vi "WVDIAL+HSRL_v4.5.vi"() -> ()   [LabVIEW 2012]
uses:
  C:/Users/H2ODial/Desktop/Shared Telescope WV DIAL Code/Libraries and VIs/PowerMeterCommands.dll
  Shared Telescope WV DIAL Code/Libraries and VIs/PowerMeterCommands.dll
  <vilib>/DAQmx/write.llb/DAQmx Write (Digital 1D Bool NChan 1Samp 1Line).vi
  <vilib>/DAQmx/miscellaneous.llb/DAQmx Fill In Error Info.vi
  <vilib>/Analysis/baseanly.llb/Mean (DBL).vi
  NCAR_DIAL_Labview/AMCS_Data.vi
  Shared Telescope WV DIAL Code/Libraries and VIs/Scalar_Data.vi
  <vilib>/Analysis/NI_AALBase.lvlib
  Shared Telescope WV DIAL Code/Libraries and VIs/Scalar_Data_2.vi
  Shared Telescope WV DIAL Code/Libraries and VIs/Scalar_Data_4.vi
  Shared Telescope WV DIAL Code/Libraries and VIs/Scalar_Data_3.vi
  Shared Telescope WV DIAL Code/bristol/CLDevIFace.dll
panel:
  out "FileHour":i32=22
  out "L_Count":i32=26
  out "background start":u32=534
  in  "Tab Control 2":enum32{"WV ND narrow", "WV ND wide"}(tab)
  out "CH3 RingBuffer long":dbl[][](array[numeric])
  out "CH3 RingBuffer short":dbl[][](array[numeric])
  in  "?":T1(tab)=enum."Raw Counts WV offline"
  out "NRB":dbl[][](graph) caption="Water Vapor Number Density"
  out "NRB 2":dbl[][](graph) caption="Water Vapor Number Density"
  out "CH 1 (WV off) counts display":dbl[][](graph)=[[72.12, 61.12, 47.12, 35.12, 44.12, 29.119999999999997, 55.12, 61.12, 47.12, 50.12, 55.12, 52.12, 68.12, 67.12, 90.12, 116.12, 122.12, 143.12, 189.12, 221.12, 229.12, 278.12, 272.12, 337.12, 351.12, 384.12, 391.12, 406.12, 455.12, 483.12, 506.12, 561.12, 539.12, 595.12, 572.12, 618.12, 622.12, 629.12, 627.12, 625.12, 613.12, 546.12, 551.12, 501.12, 476.12, 497.12, 468.12, 447.12, 391.12, 371.12, 370.12, 307.12, 290.12, 246.12, 236.12, 202.12, 237.12, 195.12, 179.12, 160.12, 142.12, 148.12, 128.12, 146.12, 132.12, 115.12, 128.12, 110.12, 91.12, 101.12, 91.12, 110.12, 101.12, 107.12, 70.12, 79.12, 81.12, 83.12, 73.12, 85.12, 77.12, 81.12, 80.12, 59.12, 76.12, 83.12, 62.12, 78.12, 75.12, 67.12, 38.12, 41.12, 47.12, 63.12, 51.12, 54.12, 58.12, 30.119999999999997, 23.119999999999997, 28.119999999999997, 23.119999999999997, 27.119999999999997, 16.119999999999997, 32.12, 40.12, 31.119999999999997, 19.119999999999997, 23.119999999999997, 26.119999999999997, 22.119999999999997, 29.119999999999997, 21.119999999999997, 8.119999999999997, 24.119999999999997, 18.119999999999997, 19.119999999999997, 33.12, 17.119999999999997, 24.119999999999997, 19.119999999999997, 12.119999999999997, 14.119999999999997, 17.119999999999997, 9.119999999999997, 24.119999999999997, 22.119999999999997, 31.119999999999997, 17.119999999999997, 9.119999999999997, 17.119999999999997, 24.119999999999997, 13.119999999999997, 4.119999999999997, 26.119999999999997, 16.119999999999997, 18.119999999999997, 11.119999999999997, 14.119999999999997, 9.119999999999997, 24.119999999999997, 6.119999999999997, 12.119999999999997, 7.119999999999997, 22.119999999999997, 3.1199999999999974, 9.119999999999997, 8.119999999999997, 16.119999999999997, 11.119999999999997, 10.119999999999997, 4.119999999999997, 0.11999999999999744, 8.119999999999997, 17.119999999999997, 3.1199999999999974, 15.119999999999997, 8.119999999999997, 4.119999999999997, 10.119999999999997, -1.8800000000000026, 7.119999999999997, 10.119999999999997, 5.119999999999997, -7.880000000000003, 2.1199999999999974, 6.119999999999997, 4.119999999999997, 13.119999999999997, 21.119999999999997, 11.119999999999997, 10.119999999999997, 3.1199999999999974, 18.119999999999997, 20.119999999999997, 10.119999999999997, 13.119999999999997, -4.880000000000003, 5.119999999999997, 9.119999999999997, 6.119999999999997, -4.880000000000003, 0.11999999999999744, 1.1199999999999974, 8.119999999999997, 5.119999999999997, 4.119999999999997, 2.1199999999999974, 3.1199999999999974, 21.119999999999997, 8.119999999999997, -0.8800000000000026, 1.1199999999999974, 9.119999999999997, 8.119999999999997, 8.119999999999997, 5.119999999999997, 1.1199999999999974, 2.1199999999999974, 2.1199999999999974, -4.880000000000003, 7.119999999999997, 2.1199999999999974, 9.119999999999997, 1.1199999999999974, -1.8800000000000026, -2.8800000000000026, -2.8800000000000026, 3.1199999999999974, 8.119999999999997, 8.119999999999997, -0.8800000000000026, 2.1199999999999974, 12.119999999999997, 8.119999999999997, -1.8800000000000026, 10.119999999999997, 1.1199999999999974, 9.119999999999997, 3.1199999999999974, 14.119999999999997, 11.119999999999997, 3.1199999999999974, 3.1199999999999974, -0.8800000000000026, -2.8800000000000026, 1.1199999999999974, 2.1199999999999974, -0.8800000000000026, 9.119999999999997, 4.119999999999997, 5.119999999999997, -7.880000000000003, -2.8800000000000026, 1.1199999999999974, -2.8800000000000026, 13.119999999999997, 26.119999999999997, 0.11999999999999744, 1.1199999999999974, 1.1199999999999974, 7.119999999999997, 3.1199999999999974, -2.8800000000000026, -8.880000000000003, 5.119999999999997, -2.8800000000000026, 2.1199999999999974, 0.11999999999999744, -1.8800000000000026, -4.880000000000003, 0.11999999999999744, 3.1199999999999974, 2.1199999999999974, 0.11999999999999744, 2.1199999999999974, 11.119999999999997, -7.880000000000003, 6.119999999999997, 10.119999999999997, 2.1199999999999974, 5.119999999999997, 2.1199999999999974, -6.880000000000003, 6.119999999999997, 8.119999999999997, 6.119999999999997, 9.119999999999997, -7.880000000000003, -0.8800000000000026, 6.119999999999997, 1.1199999999999974, 3.1199999999999974, -6.880000000000003, -7.880000000000003, 7.119999999999997, 2.1199999999999974, 5.119999999999997, 1.1199999999999974, -8.880000000000003, 0.11999999999999744, 0.11999999999999744, 8.119999999999997, 1.1199999999999974, 0.11999999999999744, 13.119999999999997, 0.11999999999999744, -0.8800000000000026, -2.8800000000000026, 2.1199999999999974, 5.119999999999997, 16.119999999999997, 10.119999999999997, 16.119999999999997, 6.119999999999997, -1.8800000000000026, 3.1199999999999974, -6.880000000000003, 7.119999999999997, -3.8800000000000026, -2.8800000000000026, -2.8800000000000026, -0.8800000000000026, -12.880000000000003, 2.1199999999999974, -4.880000000000003, -0.8800000000000026, -2.8800000000000026, 7.119999999999997, -5.880000000000003, -5.880000000000003, 2.1199999999999974, -7.880000000000003, 8.119999999999997, -3.8800000000000026, 1.1199999999999974, 0.11999999999999744, 5.119999999999997, -0.8800000000000026, 0.11999999999999744, 6.119999999999997, -2.8800000000000026, -4.880000000000003, -1.8800000000000026, 1.1199999999999974, -6.880000000000003, -0.8800000000000026, 1.1199999999999974, 8.119999999999997, 6.119999999999997, 9.119999999999997, 11.119999999999997, -2.8800000000000026, -5.880000000000003, -1.8800000000000026, 11.119999999999997, 13.119999999999997, 4.119999999999997, -7.880000000000003, 6.119999999999997, -5.880000000000003, -6.880000000000003, 2.1199999999999974, 4.119999999999997, 1.1199999999999974, 0.11999999999999744, 4.119999999999997, 1.1199999999999974, 12.119999999999997, -5.880000000000003, 4.119999999999997, -3.8800000000000026, 2.1199999999999974, 4.119999999999997, 8.119999999999997, 3.1199999999999974, 3.1199999999999974, 13.119999999999997, 1.1199999999999974, 11.119999999999997, -12.880000000000003, 5.119999999999997, -0.8800000000000026, -2.8800000000000026, -0.8800000000000026, -9.880000000000003, 7.119999999999997, -3.8800000000000026, 10.119999999999997, -2.8800000000000026, 4.119999999999997, 3.1199999999999974, 5.119999999999997, -2.8800000000000026, 5.119999999999997, 3.1199999999999974, 7.119999999999997, -11.880000000000003, 5.119999999999997, -0.8800000000000026, -2.8800000000000026, 0.11999999999999744, 1.1199999999999974, 13.119999999999997, 7.119999999999997, 2.1199999999999974, 1.1199999999999974, 1.1199999999999974, -0.8800000000000026, -5.880000000000003, 7.119999999999997, 6.119999999999997, -0.8800000000000026, -2.8800000000000026, 0.11999999999999744, -1.8800000000000026, -9.880000000000003, 2.1199999999999974, -1.8800000000000026, -3.8800000000000026, 3.1199999999999974, -3.8800000000000026, 2.1199999999999974, 2.1199999999999974, -2.8800000000000026, -4.880000000000003, -2.8800000000000026, 2.1199999999999974, -7.880000000000003, 13.119999999999997, 0.11999999999999744, 4.119999999999997, 3.1199999999999974, -0.8800000000000026, -8.880000000000003, 2.1199999999999974, -1.8800000000000026, -1.8800000000000026, 4.119999999999997, 2.1199999999999974, 2.1199999999999974, -6.880000000000003, -6.880000000000003, -8.880000000000003, -0.8800000000000026, -0.8800000000000026, 1.1199999999999974, -0.8800000000000026, -1.8800000000000026, 0.11999999999999744, 4.119999999999997, -2.8800000000000026, -4.880000000000003, -3.8800000000000026, -3.8800000000000026, 5.119999999999997, 5.119999999999997, 2.1199999999999974, -5.880000000000003, -0.8800000000000026, -7.880000000000003, -1.8800000000000026, -6.880000000000003, -7.880000000000003, 10.119999999999997, 8.119999999999997, 4.119999999999997, 5.119999999999997, 3.1199999999999974, -0.8800000000000026, -1.8800000000000026, -12.880000000000003, -7.880000000000003, 2.1199999999999974, 1.1199999999999974, -4.880000000000003, -7.880000000000003, 1.1199999999999974, 0.11999999999999744, -3.8800000000000026, 0.11999999999999744, -5.880000000000003, 0.11999999999999744, 3.1199999999999974, 16.119999999999997, 2.1199999999999974, 3.1199999999999974, 0.11999999999999744, -2.8800000000000026, 2.1199999999999974, 6.119999999999997, 1.1199999999999974, -4.880000000000003, 3.1199999999999974, 15.119999999999997, -13.880000000000003, 9.119999999999997, -0.8800000000000026, -2.8800000000000026, 10.119999999999997, 7.119999999999997, 4.119999999999997, -1.8800000000000026, 11.119999999999997, 8.119999999999997, 0.11999999999999744, 3.1199999999999974, 8.119999999999997, 1.1199999999999974, 2.1199999999999974, -11.880000000000003, 3.1199999999999974, 10.119999999999997, -2.8800000000000026, 3.1199999999999974, 7.119999999999997, -2.8800000000000026, -2.8800000000000026, -2.8800000000000026, -1.8800000000000026, 5.119999999999997, 0.11999999999999744, -2.8800000000000026, 5.119999999999997, -1.8800000000000026, -4.880000000000003, 0.11999999999999744, -7.880000000000003, -10.880000000000003, -1.8800000000000026, -2.8800000000000026, -3.8800000000000026, 1.1199999999999974, -2.8800000000000026, -0.8800000000000026, -7.880000000000003, -2.8800000000000026, 9.119999999999997, 0.11999999999999744, -5.880000000000003, 6.119999999999997, -1.8800000000000026, -0.8800000000000026, 1.1199999999999974, 5.119999999999997, 12.119999999999997, 14.119999999999997, 9.119999999999997, -2.8800000000000026, -3.8800000000000026, -7.880000000000003, -1.8800000000000026, 9.119999999999997, -8.880000000000003, 5.119999999999997, -2.8800000000000026, -5.880000000000003, -0.8800000000000026, -8.880000000000003, -1.8800000000000026, -5.880000000000003, 12.119999999999997, -2.8800000000000026, 4.119999999999997, 1.1199999999999974, 10.119999999999997, 4.119999999999997, -4.880000000000003, -3.8800000000000026, -1.8800000000000026, 8.119999999999997, 1.1199999999999974, -0.8800000000000026, -5.880000000000003, 3.1199999999999974, -9.880000000000003, -3.8800000000000026, 5.119999999999997, 2.1199999999999974, 9.119999999999997, 0.0]] caption="Water Vapor Number Density"
  out "CH 3 (HSRL comb) counts display":dbl[][](graph)=[[191.68, 101.68, 62.68000000000001, 122.68, 46.68000000000001, 67.68, 96.68, 112.68, 96.68, 178.68, 157.68, 156.68, 268.68, 230.68, 382.68, 361.68, 473.68, 521.6800000000001, 591.6800000000001, 641.6800000000001, 732.6800000000001, 820.6800000000001, 938.6800000000001, 1045.68, 1138.68, 1222.68, 1329.68, 1319.68, 1345.68, 1475.68, 1466.68, 1519.68, 1569.68, 1698.68, 1666.68, 1581.68, 1707.68, 1691.68, 1629.68, 1560.68, 1616.68, 1487.68, 1526.68, 1348.68, 1236.68, 1209.68, 1105.68, 1027.68, 970.6800000000001, 878.6800000000001, 821.6800000000001, 781.6800000000001, 646.6800000000001, 643.6800000000001, 521.6800000000001, 577.6800000000001, 505.68, 511.68, 457.68, 406.68, 391.68, 343.68, 300.68, 360.68, 268.68, 246.68, 294.68, 246.68, 241.68, 249.68, 210.68, 201.68, 201.68, 198.68, 216.68, 177.68, 157.68, 140.68, 184.68, 163.68, 154.68, 156.68, 178.68, 176.68, 137.68, 206.68, 174.68, 182.68, 148.68, 153.68, 116.68, 133.68, 117.68, 118.68, 134.68, 120.68, 110.68, 76.68, 105.68, 75.68, 147.68, 34.68000000000001, 41.68000000000001, 65.68, 54.68000000000001, 87.68, 57.68000000000001, 61.68000000000001, 59.68000000000001, 25.680000000000007, 71.68, 88.68, 31.680000000000007, 32.68000000000001, 51.68000000000001, 66.68, 75.68, 51.68000000000001, 39.68000000000001, 51.68000000000001, 40.68000000000001, 55.68000000000001, 38.68000000000001, 22.680000000000007, 20.680000000000007, 50.68000000000001, 12.680000000000007, 40.68000000000001, 11.680000000000007, 28.680000000000007, 26.680000000000007, 23.680000000000007, 28.680000000000007, 8.680000000000007, 34.68000000000001, 20.680000000000007, 57.68000000000001, -17.319999999999993, 48.68000000000001, 40.68000000000001, 83.68, -1.3199999999999932, 33.68000000000001, 42.68000000000001, 29.680000000000007, 13.680000000000007, 25.680000000000007, 10.680000000000007, 31.680000000000007, 31.680000000000007, 4.680000000000007, 15.680000000000007, 36.68000000000001, 20.680000000000007, -0.3199999999999932, 40.68000000000001, -2.319999999999993, 21.680000000000007, 19.680000000000007, -14.319999999999993, 32.68000000000001, 39.68000000000001, 48.68000000000001, 17.680000000000007, -5.319999999999993, 13.680000000000007, 0.6800000000000068, 23.680000000000007, 26.680000000000007, -14.319999999999993, -7.319999999999993, 15.680000000000007, 20.680000000000007, -19.319999999999993, 14.680000000000007, 38.68000000000001, 5.680000000000007, 11.680000000000007, 18.680000000000007, 12.680000000000007, -5.319999999999993, 40.68000000000001, -11.319999999999993, 15.680000000000007, -17.319999999999993, -12.319999999999993, 9.680000000000007, 13.680000000000007, -23.319999999999993, -6.319999999999993, 28.680000000000007, 8.680000000000007, 24.680000000000007, 34.68000000000001, -24.319999999999993, 24.680000000000007, -32.31999999999999, 13.680000000000007, 29.680000000000007, 9.680000000000007, -16.319999999999993, -4.319999999999993, -15.319999999999993, 22.680000000000007, 13.680000000000007, 17.680000000000007, 21.680000000000007, 30.680000000000007, 1.6800000000000068, 60.68000000000001, -6.319999999999993, 1.6800000000000068, -11.319999999999993, 20.680000000000007, 31.680000000000007, 18.680000000000007, 0.6800000000000068, 16.680000000000007, 21.680000000000007, -11.319999999999993, -3.319999999999993, -8.319999999999993, 12.680000000000007, -10.319999999999993, 31.680000000000007, 11.680000000000007, 32.68000000000001, 21.680000000000007, 26.680000000000007, -24.319999999999993, 0.6800000000000068, -2.319999999999993, -6.319999999999993, -1.3199999999999932, -10.319999999999993, 12.680000000000007, 1.6800000000000068, 7.680000000000007, 14.680000000000007, 1.6800000000000068, -5.319999999999993, -27.319999999999993, 9.680000000000007, -0.3199999999999932, -8.319999999999993, 30.680000000000007, -9.319999999999993, 1.6800000000000068, -4.319999999999993, 18.680000000000007, 26.680000000000007, 3.680000000000007, -12.319999999999993, 14.680000000000007, -12.319999999999993, 58.68000000000001, -10.319999999999993, 18.680000000000007, 13.680000000000007, -12.319999999999993, 31.680000000000007, -37.31999999999999, -23.319999999999993, 8.680000000000007, -5.319999999999993, 28.680000000000007, 17.680000000000007, 12.680000000000007, -4.319999999999993, 25.680000000000007, 18.680000000000007, -10.319999999999993, -4.319999999999993, -23.319999999999993, 10.680000000000007, -20.319999999999993, 8.680000000000007, 22.680000000000007, 10.680000000000007, 39.68000000000001, -20.319999999999993, -16.319999999999993, 13.680000000000007, 13.680000000000007, -27.319999999999993, 10.680000000000007, -8.319999999999993, 65.68, -4.319999999999993, 26.680000000000007, 2.680000000000007, -4.319999999999993, 5.680000000000007, -2.319999999999993, 19.680000000000007, 8.680000000000007, -36.31999999999999, -21.319999999999993, -6.319999999999993, -11.319999999999993, 6.680000000000007, 3.680000000000007, -8.319999999999993, 17.680000000000007, 26.680000000000007, 16.680000000000007, -11.319999999999993, 22.680000000000007, 0.6800000000000068, 13.680000000000007, 10.680000000000007, -23.319999999999993, 11.680000000000007, 16.680000000000007, -17.319999999999993, 9.680000000000007, -45.31999999999999, 8.680000000000007, 45.68000000000001, 16.680000000000007, -24.319999999999993, -26.319999999999993, 13.680000000000007, 2.680000000000007, -2.319999999999993, 1.6800000000000068, 33.68000000000001, -12.319999999999993, 0.6800000000000068, -2.319999999999993, 25.680000000000007, -46.31999999999999, 48.68000000000001, -30.319999999999993, 5.680000000000007, 11.680000000000007, 11.680000000000007, -14.319999999999993, -26.319999999999993, 40.68000000000001, 29.680000000000007, -3.319999999999993, -5.319999999999993, 17.680000000000007, -19.319999999999993, -12.319999999999993, -19.319999999999993, -14.319999999999993, 0.6800000000000068, 1.6800000000000068, 4.680000000000007, 4.680000000000007, -9.319999999999993, 26.680000000000007, -10.319999999999993, -4.319999999999993, -2.319999999999993, 32.68000000000001, 12.680000000000007, -9.319999999999993, 31.680000000000007, 33.68000000000001, -6.319999999999993, 14.680000000000007, 38.68000000000001, -15.319999999999993, -0.3199999999999932, 26.680000000000007, -21.319999999999993, 7.680000000000007, -22.319999999999993, 0.6800000000000068, 30.680000000000007, -11.319999999999993, 18.680000000000007, 8.680000000000007, 2.680000000000007, 18.680000000000007, 7.680000000000007, 31.680000000000007, 25.680000000000007, 37.68000000000001, 3.680000000000007, -22.319999999999993, -7.319999999999993, -22.319999999999993, 2.680000000000007, 23.680000000000007, 12.680000000000007, -38.31999999999999, 3.680000000000007, 27.680000000000007, -0.3199999999999932, -18.319999999999993, 5.680000000000007, -10.319999999999993, 17.680000000000007, -17.319999999999993, 35.68000000000001, 20.680000000000007, 14.680000000000007, -2.319999999999993, -10.319999999999993, 3.680000000000007, -25.319999999999993, 18.680000000000007, -6.319999999999993, -11.319999999999993, 11.680000000000007, 3.680000000000007, 34.68000000000001, -5.319999999999993, -19.319999999999993, 29.680000000000007, -21.319999999999993, 17.680000000000007, -11.319999999999993, 18.680000000000007, 13.680000000000007, -12.319999999999993, 16.680000000000007, -14.319999999999993, 5.680000000000007, -19.319999999999993, -15.319999999999993, 6.680000000000007, 14.680000000000007, -14.319999999999993, 25.680000000000007, 32.68000000000001, -35.31999999999999, 34.68000000000001, 15.680000000000007, -15.319999999999993, 36.68000000000001, -13.319999999999993, 4.680000000000007, 1.6800000000000068, -16.319999999999993, -20.319999999999993, 14.680000000000007, 20.680000000000007, -14.319999999999993, -22.319999999999993, -36.31999999999999, -10.319999999999993, 16.680000000000007, -10.319999999999993, 28.680000000000007, 8.680000000000007, -9.319999999999993, 9.680000000000007, 13.680000000000007, -2.319999999999993, 31.680000000000007, 36.68000000000001, -3.319999999999993, 7.680000000000007, -16.319999999999993, -14.319999999999993, 27.680000000000007, 34.68000000000001, 15.680000000000007, -48.31999999999999, 0.6800000000000068, -11.319999999999993, -7.319999999999993, -15.319999999999993, -13.319999999999993, 15.680000000000007, -27.319999999999993, 0.6800000000000068, -13.319999999999993, -9.319999999999993, -12.319999999999993, 1.6800000000000068, 4.680000000000007, -1.3199999999999932, 17.680000000000007, -6.319999999999993, 15.680000000000007, 9.680000000000007, 51.68000000000001, -13.319999999999993, -0.3199999999999932, 43.68000000000001, -17.319999999999993, 10.680000000000007, 1.6800000000000068, -16.319999999999993, -5.319999999999993, -31.319999999999993, 38.68000000000001, 17.680000000000007, -24.319999999999993, 36.68000000000001, -22.319999999999993, -7.319999999999993, -41.31999999999999, 23.680000000000007, -0.3199999999999932, 38.68000000000001, -12.319999999999993, 40.68000000000001, 16.680000000000007, -0.3199999999999932, 4.680000000000007, -18.319999999999993, -3.319999999999993, -20.319999999999993, 20.680000000000007, -32.31999999999999, -37.31999999999999, -5.319999999999993, -25.319999999999993, -12.319999999999993, 27.680000000000007, -17.319999999999993, -23.319999999999993, 20.680000000000007, 45.68000000000001, -23.319999999999993, 10.680000000000007, -36.31999999999999, 7.680000000000007, -30.319999999999993, 43.68000000000001, 24.680000000000007, -26.319999999999993, 17.680000000000007, -4.319999999999993, -0.3199999999999932, -45.31999999999999, -1.3199999999999932, 8.680000000000007, -13.319999999999993, -27.319999999999993, -14.319999999999993, 10.680000000000007, -17.319999999999993, -39.31999999999999, 20.680000000000007, -38.31999999999999, 8.680000000000007, -5.319999999999993, 27.680000000000007, -5.319999999999993, 13.680000000000007, -5.319999999999993, -14.319999999999993, 24.680000000000007, 8.680000000000007, 1.6800000000000068, 14.680000000000007, 5.680000000000007, 31.680000000000007, -2.319999999999993, 33.68000000000001, -28.319999999999993, 0.0]] caption="Water Vapor Number Density"
  out "CH3 (HSRL combined) smooth S":dbl[](array[numeric])=[96.57850299401198, 56.5485628742515, 55.743173652694615, 60.75365269461079, 68.32101796407187, 79.13089820359284, 91.49317365269464, 103.12341317365271, 117.9422754491018, 136.07401197604787, 156.80904191616764, 183.49467065868262, 215.12191616766466, 251.2985628742515, 292.9602395209581, 339.6967664670659, 389.76263473053893, 444.4722155688622, 499.4991616766466, 554.9482634730538, 610.9767065868263, 666.3225149700597, 722.5261077844309, 775.5335928143711, 824.4602395209581, 870.2566467065868, 910.9826946107785, 946.3719161676647, 976.2416766467067, 996.7252095808384, 1009.2656287425151, 1012.3225149700601, 1009.514131736527, 996.7431736526947, 977.3794011976049, 952.3314970059882, 918.1353892215569, 883.2297005988024, 842.770119760479, 803.6967664670657, 765.9901796407183, 730.4228143712572, 698.6144311377244, 665.4332934131735, 632.464730538922, 597.6563473053891, 562.395868263473, 527.2476646706585, 490.38389221556884, 453.2596407185628, 416.91982035928146, 384.87790419161684, 359.6308982035929, 339.24916167664674, 323.0964670658683, 306.9407784431138, 290.8943712574851, 275.00814371257485, 259.09497005988027, 245.14586826347306, 232.85544910179638, 219.72820359281437, 209.2985628742515, 199.46173652694605, 190.8764071856287, 184.17880239520954, 177.13538922155684, 171.00514970059874, 164.5335928143712, 159.33748502994007, 153.19077844311371, 146.91532934131732, 140.66682634730535, 133.9497604790419, 127.57850299401198, 121.32850299401197, 116.12790419161676, 111.50814371257485, 107.55305389221559, 105.40335329341318, 100.72970059880242, 97.00215568862279, 93.73269461077848, 89.03808383233537, 85.88538922155692, 82.84347305389224, 78.60844311377248, 74.91832335329343, 71.71473053892218, 67.18628742514973, 64.15634730538923, 60.55305389221558, 58.217724550898204, 55.970718562874254, 54.10694610778443, 51.50065868263473, 49.30604790419162, 48.15335329341319, 45.8165269461078, 44.460239520958105, 41.942275449101814, 40.92131736526947, 39.90035928143714, 39.27610778443116, 38.603952095808395, 37.83149700598804, 36.43329341317367, 35.211736526946126, 34.198263473053906, 32.17730538922157, 31.78359281437127, 30.72670658682636, 30.120419161676665, 29.090479041916193, 27.45275449101798, 27.16083832335331, 26.844970059880254, 26.455748502994023, 26.82850299401199, 25.8734131736527, 24.551556886227544, 23.198263473053885, 22.36892215568862, 22.11592814371257, 21.767125748502984, 21.66383233532933, 21.29556886227544, 19.8180239520958, 18.47970059880239, 17.994670658682626, 16.57850299401197, 17.27161676646706, 17.111437125748495, 17.017125748502988, 17.100958083832328, 16.057544910179637, 16.803053892215566, 16.35844311377245, 16.12041916167664, 15.717724550898199, 14.449760479041911, 14.097964071856282, 13.937784431137722, 12.99766467065868, 12.740179640718562, 12.024610778443115, 11.10994011976048, 11.081497005988027, 11.527604790419161, 11.419820359281436, 12.032095808383232, 12.350958083832333, 11.291077844311376, 10.617425149700598, 10.120419161676647, 9.60245508982036, 9.635389221556888, 10.02610778443114, 9.349461077844314, 8.891377245508984, 8.46622754491018, 7.355449101796408, 7.225209580838324, 7.153353293413174, 7.925808383233534, 8.484191616766466, 7.698263473053894, 8.123413173652695, 7.041077844311378, 7.35994011976048, 7.412335329341318, 6.8404790419161685, 6.994670658682637, 6.331497005988025, 7.01562874251497, 6.918323353293413, 6.858443113772456, 6.587485029940119, 6.332994011976048, 6.319520958083834, 5.9048502994011995, 5.970718562874254, 5.045568862275452, 5.148862275449105, 5.349461077844313, 5.244670658682637, 6.243173652694611, 6.478203592814372, 6.171317365269461, 5.891377245508982, 5.395868263473056, 4.359940119760481, 4.858443113772457, 4.732694610778444, 4.392874251497008, 5.433293413173654, 4.508143712574853, 4.328502994011979, 4.924311377245511, 4.232694610778445, 4.409341317365271, 4.756646706586827, 4.835988023952097, 4.984191616766468, 5.324011976047905, 4.69676646706587, 4.080000000000002, 3.255149700598805, 2.2850898203592838, 3.121916167664673, 2.8554491017964096, 3.1114371257485054, 3.2626347305389243, 2.801556886227547, 1.982694610778445, 1.7686227544910205, 1.1413772455089841, 0.8973652694610804, 1.7386826347305413, 2.3539520958083853, 3.216227544910182, 3.3105389221556907, 3.077005988023955, 2.6773053892215595, 2.3045508982035954, 2.303053892215571, 2.6563473053892235, 2.057544910179643, 1.9782035928143733, 1.376407185628745, 0.844970059880242, 1.2252095808383259, 1.1413772455089846, 1.29107784431138, 1.0829940119760506, 1.2057485029940147, 1.3779041916167691, 0.921317365269464, 1.446766467065871, 1.1204191616766492, 1.1398802395209604, 1.4392814371257507, 1.5755089820359305, 1.5036526946107809, 1.5680239520958112, 1.5051497005988053, 0.9677245508982063, 0.9707185628742541, 0.6518562874251523, 0.6653293413173678, 0.8704191616766495, 0.8240119760479069, 0.5291017964071884, 0.3569461077844339, -0.30473053892215296, -0.3092215568862249, -0.13257485029939847, -0.050239520958081194, 0.28359281437126016, -0.16850299401197344, -0.14155688622754228, 0.4767065868263499, 0.8449700598802421, 1.4647305389221583, 2.258143712574853, 2.856946107784433, 3.120419161676649, 2.608443113772457, 1.3165269461077869, 0.23568862275449384, -0.008323353293410496, -0.22838323353293155, 0.30604790419161926, 0.6563473053892241, 0.5695209580838348, 1.1728143712574877, 1.2596407185628768, 0.8988622754491045, 0.5785029940119788, 0.1907784431137751, -0.5113173652694584, -0.554730538922153, -0.49335329341317097, 0.6368862275449125, 1.9871856287425171, 1.6638323353293438, 2.318023952095811, 1.7521556886227572, 0.8344910179640747, 1.3808982035928172, 0.47670658682635, 0.3344910179640745, 0.5081437125748529, 0.9018562874251522, 1.223712574850302, 0.3644311377245535, 0.2551497005988051, -0.3825748502993984, 0.03359281437126005, 0.6204191616766492, 0.6638323353293438, -0.0023353293413148624, -0.5143113772455064, -0.6355688622754464, 0.024610778443116432, 1.0485628742514996, 1.2087425149700626, 1.011137724550901, 0.37191616766467334, 0.6922754491017991, 0.16233532934132008, 0.7761077844311401, 0.9826946107784456, 0.31802395209581097, 0.44377245508982277, -0.4469461077844284, -0.2822754491017937, -0.45443113772454824, -0.38257485029939853, 0.1862874251497032, -0.2388622754490992, 0.22670658682634998, 0.15485029940120032, 0.20125748502994284, 0.024610778443116488, -0.027784431137721888, -0.4484431137724524, -0.988862275449099, 0.17281437125748766, 0.2222155688622779, 1.002155688622757, 1.6608383233532957, 0.7416766467065893, 0.3674251497006015, -0.28227544910179364, -0.5831736526946081, -0.5697005988023924, -0.5652095808383207, -0.2448502994011949, -0.16401197604790152, -0.021796407185626004, 0.05754491017964346, 0.4662275449101823, 0.19676646706587098, -0.49335329341317097, -0.8092215568862249, -1.1580239520958058, -0.9828742514970034, 0.02910179640718835, 0.14736526946108053, -0.16550898203592546, 0.08748502994012246, -1.4274850299401172, -2.114610778443111, -1.8750898203592792, -2.3571257485029915, -1.4095209580838297, -0.12359281437125474, -0.6385628742514943, -0.49634730538921895, -0.6550299401197578, -0.8122155688622726, -0.7792814371257459, -0.23437125748502746, 0.0006586826347329544, -0.018802395209578465, 0.17580838323353554, -0.7927544910179614, -0.7179041916167637, -1.3211976047904168, -0.5996407185628718, 0.40784431137724786, 0.8689221556886251, 1.3584431137724577, 0.5710179640718589, -0.1131137724550873, -0.9694011976047879, -1.3137125748502967, -0.3571257485029914, 0.4407784431137754, 0.38239520958084117, 0.19976047904191901, -0.6086227544910152, -0.7508383233532909, 0.03508982035928404, 0.13838323353293663, 0.3165269461077869, -0.015808383233530385, -0.5502395209580813, 0.02910179640718824, 0.4722155688622781, 0.11742514970060147, -0.43946107784430866, -1.0307784431137696, -1.1670059880239492, -0.9229940119760451, -0.7463473053892188, -0.8107185628742488, -0.9798802395209553, -0.5113173652694585, -0.06670658682634473, -0.10862275449101527, -0.2568263473053865, -1.0472455089820332, -1.3810778443113745, -0.8571257485029913, -0.3002395209580812, -0.07269461077844042, -0.08616766467065612, -0.9469461077844287, -1.3900598802395185, -0.9319760479041891, -0.7283832335329316, 0.2222155688622781, 0.6189221556886254, 0.7177245508982062, 0.3255089820359307, -0.0667065868263447, -1.3286826347305363, -1.5517365269461052, -0.6685029940119736, -0.3975449101796383, 0.32550898203593065, 0.5814970059880264, 0.08149700598802662, 0.3614371257485056, 0.41233532934132, 0.17580838323353556, 0.7865868263473079, -0.024790419161674015, 0.38988023952096074, -0.07718562874251239, -0.4349700598802369, -0.6325748502993987, -0.4005389221556862, -0.0023353293413149318, 0.008143712574852732, 0.3913772455089847, 0.18928143712575124, -0.17598802395209306, -0.16850299401197333, 0.18628742514970326, -0.2508383233532908, 0.38988023952096074, 0.2446706586826374, 0.8105389221556913, 0.6982634730538947, 0.035089820359283874, 0.07101796407185874, -0.8361676646706562, -0.5921556886227518, 0.5575449101796437, 0.24167664670658967, 0.5216167664670686, 0.28059880239521234, -0.38257485029939864, -0.3256886227544883, -0.3182035928143685, 0.29257485029940394, 0.37640718562874526, 0.31203592814371534, -0.12658682634730267, -0.5367664670658656, -1.4140119760479015, -0.9185029940119734, -1.1400598802395183, -1.0307784431137699, -0.6924550898203566, -0.993353293413171, -0.336167664670656, -0.12808383233532672, -0.02329341317365005, -0.15652694610778173, -0.24335329341317097, -0.366107784431135, -0.20592814371257215, -1.0247904191616741, -1.304730538922153, -2.0113173652694583, -2.0113173652694583, -1.2777844311377216, -0.9454491017964044, -0.8795808383233505, -1.0472455089820332, -0.5307784431137696, -0.40952095808382954, -0.7283832335329314, -1.190958083832333, -1.0786826347305365, -1.2343712574850274, -0.35862275449101566, -0.027784431137721888, -0.6131137724550872, -0.25982035928143454, -0.7523353293413146, -0.06221556886227286, 0.2446706586826374, -0.5951497005987998, 0.3943712574850326, -0.43796407185628466, -0.03227544910179364, -0.2613173652694585, -0.8002395209580812, -1.3960479041916143, -1.7268862275449077, -1.2074251497005961, -1.592155688622752, -0.7762874251496981, -1.7882634730538896, -1.7732934131736504, -1.4963473053892191, -1.2882634730538898, -0.5502395209580812, 0.23568862275449354, 0.4138323353293438, 0.5470658682634756, 1.0455688622754518, 0.7117365269461104, 0.8779041916167689, 0.506646706586829, -0.279281437125746, -0.9095209580838297, -1.2343712574850272, -0.9439520958083806, -0.4753892215568837, -0.6849700598802371, -1.0951497005987998, -0.5547305389221528, -0.008323353293410385, 0.11443113772455371, 0.12041916167664946, -0.39455089820359013, -1.2179041916167639, -0.7508383233532907, -0.1460479041916141, -0.056227544910176994, 0.16083832335329604, 0.38838323353293674, 0.3764071856287451, -0.09814371257484766, 0.10245508982036192, -0.44544910179640457, 0.002155688622757057, 0.909341317365272, 1.1847904191616792, 1.2865868263473081, 0.27011976047904457, 0.42730538922155953, 0.3539520958083858, 0.385389221556889, 0.5755089820359309, -0.5083233532934106, -0.6355688622754465, -0.3526347305389195, -0.42748502994011717]
  out "CH3 (HSRL combined) smooth L":dbl[](array[numeric])=[96.57782268578879, 56.14594524119948, 55.284471968709255, 61.11498044328552, 69.86172099087352, 81.79164276401562, 94.22254237288134, 105.95428943937416, 120.80859191655802, 139.2196088657106, 161.05142112125168, 187.96308996088663, 219.25872229465458, 254.74340286831816, 295.29750977835715, 339.44972620599714, 387.9331029986959, 439.557614080834, 492.626388526727, 545.7593741851365, 598.6410560625811, 650.8597653194263, 702.3239113428945, 752.3959452411998, 799.7212385919167, 845.3190221642766, 887.6149804432855, 925.6192177314208, 958.6068318122551, 983.5452281616683, 998.05109517601, 1003.7929465449799, 1001.847053455019, 990.4963363754885, 973.4963363754883, 949.8855149934805, 917.1824511082133, 879.8979009126463, 837.6052020860495, 792.7179791395049, 748.5243676662326, 706.5592438070411, 668.0256714471974, 632.9888396349417, 601.1919035202087, 570.5113298565839, 539.1003129074313, 505.28805736636207, 470.15409387222905, 434.931799217731, 403.0038331160361, 377.07782268578836, 355.5328422425029, 337.7652411994783, 321.3141329856583, 304.9911212516297, 288.34672750977836, 272.32130378096485, 257.3408604954368, 242.55924380704045, 230.16419817470668, 217.77110821382013, 207.1120469361148, 197.92202086049554, 189.21993481095188, 181.73786179921785, 174.3411864406781, 167.29555410691015, 160.25187744458935, 154.22221642764018, 147.62117340286832, 141.436036505867, 135.21960886571057, 128.45168187744457, 122.80044328552802, 117.3688917861799, 112.34835723598431, 108.21830508474571, 103.87573663624507, 100.31674054758795, 96.02958279009121, 92.06902216427635, 88.6100912646675, 84.78512385919163, 82.11595827900909, 78.76687092568446, 75.46960886571054, 72.14887874837027, 68.71797913950456, 65.30500651890483, 62.1971186440678, 58.821629726206, 56.04196870925686, 53.966675358539774, 51.680821382007835, 49.69516297262062, 48.210482398957, 46.78675358539769, 45.25513689700134, 44.30109517601046, 42.81315514993484, 41.88910039113432, 40.84770534550198, 39.69679269882661, 38.56641460234681, 37.43310299869622, 36.204941329856574, 35.0628292046936, 33.80826597131681, 32.57097783572358, 32.01882659713167, 31.285123859191643, 30.654419817470654, 29.41810951760103, 28.24405475880051, 27.440599739243797, 26.95135593220339, 26.45102998696219, 25.908331160365062, 25.011003911342897, 24.234602346805737, 23.406049543676662, 22.896597131681876, 22.461134289439375, 21.706571056062586, 21.531538461538464, 21.241447196870933, 20.47286831812256, 20.057614080834426, 19.42332464146024, 18.49340286831813, 18.34314211212517, 17.519152542372897, 17.10357235984356, 17.038709256844868, 16.499595827900933, 16.7095045632334, 16.336623207301194, 16.012959582790113, 15.58890482398959, 15.166153846153867, 14.87052151238594, 14.433428943937436, 14.079126466753598, 13.899530638852687, 13.39985658409388, 12.850312907431555, 12.396271186440682, 12.103246414602342, 12.016870925684481, 11.910938722294652, 11.907679269882658, 11.203963494132983, 10.781864406779658, 10.658983050847455, 10.696140808344193, 10.539687092568446, 10.454289439374183, 9.743076923076922, 9.147249022164278, 9.092816166883964, 8.512307692307694, 8.241121251629727, 7.990795306388527, 8.024693611473275, 8.063807040417213, 7.583689700130382, 7.693859191655806, 7.43505867014342, 7.314132985658414, 7.367262059973929, 7.202659713168192, 6.994054758800525, 7.157027379400264, 7.640730117340289, 7.471564537157761, 7.390404172099091, 6.902464146023472, 6.485906127770539, 6.342164276401569, 6.240143415906132, 6.04229465449805, 5.939295958279014, 5.827496740547593, 5.563807040417215, 5.427235984354632, 5.321303780964801, 5.608135593220342, 5.2616558018252935, 5.204289439374185, 5.029908735332463, 4.51915254237288, 4.817718383311605, 4.8503129074315545, 4.795228161668842, 4.866936114732726, 4.5048109517601045, 4.315762711864406, 4.505788787483702, 4.542620599739244, 4.58988265971317, 4.7603520208604975, 4.501225554106912, 4.121825293350717, 4.048161668839635, 4.049791395045632, 4.003833116036505, 3.6361668839634946, 3.225475880052152, 2.966023468057366, 3.0905345501955686, 3.1537679269882672, 3.4057235984354626, 3.0246936114732734, 2.6332333767926985, 2.746010430247718, 2.450052151238593, 2.3770404172099098, 2.4138722294654507, 2.449074315514993, 2.7701303780964786, 2.898552803129073, 2.7968578878748365, 2.467653194263364, 2.3848631029986973, 2.455919165580183, 2.5442503259452414, 2.597705345501956, 2.2691525423728813, 2.211460234680574, 1.8816036505867024, 2.0595697522816176, 2.224823989569754, 2.2183050847457637, 2.374758800521513, 2.011329856584095, 1.962112125162974, 1.7277574967405493, 1.5452281616688417, 1.8050065189048259, 1.6068318122555425, 2.0168709256844854, 2.1873402868318124, 1.804028683181226, 1.919087353324642, 1.579452411994786, 1.4995958279009138, 1.309569752281618, 1.0866232073011743, 1.215371577574968, 1.3362972620599747, 1.6547457627118654, 1.8069621903520212, 1.7147196870925692, 1.4608083441981752, 1.2717601043024775, 1.2750195567144726, 1.0706518904823994, 1.1299739243807048, 1.340208604954368, 1.1078096479791402, 1.2489439374185143, 1.5631551499348122, 1.422346805736638, 1.881929595827902, 1.609439374185138, 1.5732594524119956, 1.6133507170795316, 1.2629595827900923, 1.5533767926988278, 1.3552020860495446, 1.1452933507170804, 1.2812125162972634, 1.1697392438070418, 0.9859061277705361, 1.1237809647979151, 0.9314732724902227, 0.9262581486310311, 0.7900130378096493, 0.7466623207301188, 0.8007692307692322, 0.9507040417209924, 0.9405997392438086, 1.1609387222946557, 1.226453715775751, 1.2329726205997402, 1.2916427640156465, 1.1990743155149945, 0.9298435462842255, 0.5693481095176025, 0.653767926988267, 0.3561799217731434, 0.6273663624511092, 0.730691003911344, 0.5823859191655815, 0.36367666232073137, 0.26100391134289513, 0.22514993481095263, 0.3473794002607571, 0.6795176010430257, 0.6615906127770549, 0.2147196870925699, 0.061199478487615463, 0.2544850065189059, 0.16647979139504684, 0.7222164276401574, 0.8203259452412005, 0.8111994784876152, 0.8222816166883975, 0.8102216427640171, 0.5559843546284239, 0.3610691003911359, 0.15898305084745884, 0.0338200782268591, 0.1289960886571068, -0.21161668839634834, -0.13925684485006382, -0.47074315514993337, -0.591016949152541, -0.17543676662320573, 0.1615906127770549, 0.8193481095176025, 0.7440547588005231, 0.9409256844850078, 0.4334289439374201, -0.001707953063883872, 0.03773142112125308, -0.12393741851368828, 0.13844850065189188, 0.3131551499348121, 0.6857105606258159, 0.7482920469361158, 0.5413168187744469, 0.5325162972620612, 0.33075619295958403, -0.15131681877444444, 0.2166753585397664, 0.05272490221642889, -0.2090091264667523, 0.2952281616688407, 0.12475880052151368, 0.28642764015645494, 0.3568318122555424, -0.02745762711864258, -0.21259452411994617, -0.3742633637548876, -0.011160365058668686, -0.07406779661016809, 0.09607561929595956, -0.1014471968709244, -0.4599869621903506, -0.04179921773141981, -0.52289439374185, -0.43651890482398803, -0.3902346805736622, -0.5770013037809631, -0.1359973924380688, 0.04392438070404332, 0.02697522816167036, 0.01002607561929756, 0.10650586701434292, 0.3512907431551512, 0.261329856584095, 0.3314080834419829, 0.2678487614080848, 0.021760104302478586, 0.37182529335071846, -0.1695697522816152, -0.10079530638852535, -0.3325423728813547, -0.3661147327249009, 0.08662320730117452, 0.17039113428944053, 0.2297131681877457, 0.052724902216428865, 0.044902216427641514, -0.09166883963494009, -0.3273272490221635, -0.12947848761408023, -0.022568448500651497, 0.18897001303781014, 0.25904823989569814, 0.12704041720990966, -0.01930899608865604, -0.29701434159061146, 0.31022164276401726, 0.1671316818774462, 0.45102998696219193, 0.43245110821382166, 0.2958800521512399, 0.4937288135593236, 0.10650586701434303, 0.1967926988265986, -0.21292046936114584, 0.09477183833116126, 0.03414602346805837, -0.25235984354628327, -0.1878226857887864, -0.702164276401563, -0.36741851368969863, -0.1839113428943923, -0.2741981747066478, -0.0417992177314198, -0.08091264667535752, -0.19988265971316715, 0.24666232073011812, 0.24470664928292152, 0.2342764015645385, 0.26458930899608996, -0.12361147327248863, -0.2914732724902201, -0.376544980443284, -0.4309778357235968, -0.2070534550195552, 0.3659582790091282, 0.7082007822685807, 0.5175228161668856, 0.3679139504563249, -0.5372359843546272, -0.9857366362451097, -0.5642894393741837, -0.2859322033898291, 0.2616558018252948, 0.35455019556714606, 0.25578878748370415, 0.19874837027379544, -0.06363754889178452, -0.043754889178616564, -0.042125162972619284, -0.48541069100391054, -0.13860495436766493, -0.3964276401564525, -0.5525554106910027, -0.25333767926988093, -0.27647979139504464, -0.2086831812255527, 0.0647848761408098, 0.002529335071709493, -0.08286831812255367, -0.01637548891786013, 0.11758800521512537, 0.5615254237288151, 0.24829204693611617, 0.32000000000000134, -0.2523598435462828, -0.159139504563232, -0.028109517601041786, 0.04131681877444708, 0.13779661016949246, -0.4319556714471958, -0.5215906127770522, -0.420547588005214, -0.20379400260756056, -0.05288135593220207, 0.5497913950456336, 0.5849934810951773, 0.5621773142112139, 0.5761929595827912, 0.4027900912646684, 0.38486310299869725, 0.16680573663624593, 0.3666101694915264, 0.17593220338983195, -0.2562711864406767, 0.028604954367667676, -0.2826727509778343, -0.2344328552803115, 0.017196870925685802, -0.10829204693611344, 0.17234680573663763, 0.2968578878748384, 0.49340286831812397, 0.5191525423728828, 0.3102216427640171, 0.055332464146024996, 0.013611473272491889, -0.03723598435462702, 0.09053455019556853, -0.07048239895697388, -0.2187874837027366, 0.040990873533248054, -0.027457627118642483, 0.06739243807040571, -0.06559322033898146, -0.023872229465448674, 0.04131681877444714, 0.20657105606258258, 0.28088657105606357, -0.15653194263363612, -0.40327249022164136, -0.2924511082138185, -0.2249804432855264, 0.1514863102998712, 0.4135462842242519, 0.12019556714472128, 0.3656323337679285, 0.19483702737940176, 0.022737940026077152, 0.20461538461538614, 0.0807561929595843, 0.25481095176010554, 0.18897001303781089, -0.043102998696217726, -0.09036505867014194, -0.2683311603650569, 0.027627118644069387, 0.40441981747066635, 0.2874054758800536, 0.19516297262060112, -0.2637679269882647, -0.5580964797913937, -0.5949282920469346, -0.3670925684484992, -0.08352020860495278, 0.14170795306388675, 0.43016949152542483, 0.5709778357235994, 0.7143937418513702, 1.0204563233376807, 0.5413168187744475, 0.3183702737940044, 0.24307692307692474, -0.30353324641460094, -0.1340417209908724, -0.20086049543676554, -0.4296740547587993, -0.46455019556714333, -0.2011864406779647, -0.2741981747066478, -0.23964797913950311, -0.15522816166883818, -0.2647457627118626, -0.3472099087353308, -0.5483181225554093, -0.3703520208604942, -0.3651368970013024, -0.08938722294654361, 0.20917861799217888, 0.09118644067796754, -0.16924380704041583, -0.06331160365058539, -0.16565840938722148, -0.3494915254237274, -0.2816949152542358, 0.02176010430247871, -0.14773142112125043, -0.023546284224248974, 0.15898305084745878, -0.1304563233376782, 0.19157757496740682, 0.46146023468057495, 0.3493350717079545, 0.20363754889178776, 0.2505736636245126, 0.32521512385919304]
  out "CH3 Bin Readings":dbl[](array[numeric])=[573.0, 483.0, 444.0, 504.0, 428.0, 449.0, 478.0, 494.0, 478.0, 560.0, 539.0, 538.0, 650.0, 612.0, 764.0, 743.0, 855.0, 903.0, 973.0, 1023.0, 1114.0, 1202.0, 1320.0, 1427.0, 1520.0, 1604.0, 1711.0, 1701.0, 1727.0, 1857.0, 1848.0, 1901.0, 1951.0, 2080.0, 2048.0, 1963.0, 2089.0, 2073.0, 2011.0, 1942.0, 1998.0, 1869.0, 1908.0, 1730.0, 1618.0, 1591.0, 1487.0, 1409.0, 1352.0, 1260.0, 1203.0, 1163.0, 1028.0, 1025.0, 903.0, 959.0, 887.0, 893.0, 839.0, 788.0, 773.0, 725.0, 682.0, 742.0, 650.0, 628.0, 676.0, 628.0, 623.0, 631.0, 592.0, 583.0, 583.0, 580.0, 598.0, 559.0, 539.0, 522.0, 566.0, 545.0, 536.0, 538.0, 560.0, 558.0, 519.0, 588.0, 556.0, 564.0, 530.0, 535.0, 498.0, 515.0, 499.0, 500.0, 516.0, 502.0, 492.0, 458.0, 487.0, 457.0, 529.0, 416.0, 423.0, 447.0, 436.0, 469.0, 439.0, 443.0, 441.0, 407.0, 453.0, 470.0, 413.0, 414.0, 433.0, 448.0, 457.0, 433.0, 421.0, 433.0, 422.0, 437.0, 420.0, 404.0, 402.0, 432.0, 394.0, 422.0, 393.0, 410.0, 408.0, 405.0, 410.0, 390.0, 416.0, 402.0, 439.0, 364.0, 430.0, 422.0, 465.0, 380.0, 415.0, 424.0, 411.0, 395.0, 407.0, 392.0, 413.0, 413.0, 386.0, 397.0, 418.0, 402.0, 381.0, 422.0, 379.0, 403.0, 401.0, 367.0, 414.0, 421.0, 430.0, 399.0, 376.0, 395.0, 382.0, 405.0, 408.0, 367.0, 374.0, 397.0, 402.0, 362.0, 396.0, 420.0, 387.0, 393.0, 400.0, 394.0, 376.0, 422.0, 370.0, 397.0, 364.0, 369.0, 391.0, 395.0, 358.0, 375.0, 410.0, 390.0, 406.0, 416.0, 357.0, 406.0, 349.0, 395.0, 411.0, 391.0, 365.0, 377.0, 366.0, 404.0, 395.0, 399.0, 403.0, 412.0, 383.0, 442.0, 375.0, 383.0, 370.0, 402.0, 413.0, 400.0, 382.0, 398.0, 403.0, 370.0, 378.0, 373.0, 394.0, 371.0, 413.0, 393.0, 414.0, 403.0, 408.0, 357.0, 382.0, 379.0, 375.0, 380.0, 371.0, 394.0, 383.0, 389.0, 396.0, 383.0, 376.0, 354.0, 391.0, 381.0, 373.0, 412.0, 372.0, 383.0, 377.0, 400.0, 408.0, 385.0, 369.0, 396.0, 369.0, 440.0, 371.0, 400.0, 395.0, 369.0, 413.0, 344.0, 358.0, 390.0, 376.0, 410.0, 399.0, 394.0, 377.0, 407.0, 400.0, 371.0, 377.0, 358.0, 392.0, 361.0, 390.0, 404.0, 392.0, 421.0, 361.0, 365.0, 395.0, 395.0, 354.0, 392.0, 373.0, 447.0, 377.0, 408.0, 384.0, 377.0, 387.0, 379.0, 401.0, 390.0, 345.0, 360.0, 375.0, 370.0, 388.0, 385.0, 373.0, 399.0, 408.0, 398.0, 370.0, 404.0, 382.0, 395.0, 392.0, 358.0, 393.0, 398.0, 364.0, 391.0, 336.0, 390.0, 427.0, 398.0, 357.0, 355.0, 395.0, 384.0, 379.0, 383.0, 415.0, 369.0, 382.0, 379.0, 407.0, 335.0, 430.0, 351.0, 387.0, 393.0, 393.0, 367.0, 355.0, 422.0, 411.0, 378.0, 376.0, 399.0, 362.0, 369.0, 362.0, 367.0, 382.0, 383.0, 386.0, 386.0, 372.0, 408.0, 371.0, 377.0, 379.0, 414.0, 394.0, 372.0, 413.0, 415.0, 375.0, 396.0, 420.0, 366.0, 381.0, 408.0, 360.0, 389.0, 359.0, 382.0, 412.0, 370.0, 400.0, 390.0, 384.0, 400.0, 389.0, 413.0, 407.0, 419.0, 385.0, 359.0, 374.0, 359.0, 384.0, 405.0, 394.0, 343.0, 385.0, 409.0, 381.0, 363.0, 387.0, 371.0, 399.0, 364.0, 417.0, 402.0, 396.0, 379.0, 371.0, 385.0, 356.0, 400.0, 375.0, 370.0, 393.0, 385.0, 416.0, 376.0, 362.0, 411.0, 360.0, 399.0, 370.0, 400.0, 395.0, 369.0, 398.0, 367.0, 387.0, 362.0, 366.0, 388.0, 396.0, 367.0, 407.0, 414.0, 346.0, 416.0, 397.0, 366.0, 418.0, 368.0, 386.0, 383.0, 365.0, 361.0, 396.0, 402.0, 367.0, 359.0, 345.0, 371.0, 398.0, 371.0, 410.0, 390.0, 372.0, 391.0, 395.0, 379.0, 413.0, 418.0, 378.0, 389.0, 365.0, 367.0, 409.0, 416.0, 397.0, 333.0, 382.0, 370.0, 374.0, 366.0, 368.0, 397.0, 354.0, 382.0, 368.0, 372.0, 369.0, 383.0, 386.0, 380.0, 399.0, 375.0, 397.0, 391.0, 433.0, 368.0, 381.0, 425.0, 364.0, 392.0, 383.0, 365.0, 376.0, 350.0, 420.0, 399.0, 357.0, 418.0, 359.0, 374.0, 340.0, 405.0, 381.0, 420.0, 369.0, 422.0, 398.0, 381.0, 386.0, 363.0, 378.0, 361.0, 402.0, 349.0, 344.0, 376.0, 356.0, 369.0, 409.0, 364.0, 358.0, 402.0, 427.0, 358.0, 392.0, 345.0, 389.0, 351.0, 425.0, 406.0, 355.0, 399.0, 377.0, 381.0, 336.0, 380.0, 390.0, 368.0, 354.0, 367.0, 392.0, 364.0, 342.0, 402.0, 343.0, 390.0, 376.0, 409.0, 376.0, 395.0, 376.0, 367.0, 406.0, 390.0, 383.0, 396.0, 387.0, 413.0, 379.0, 415.0, 353.0]
  out "CH2 (molecular) smoothed":dbl[](array[numeric])=[27.15407407407407, 15.154074074074073, 12.274444444444441, 13.200370370370367, 13.404074074074071, 15.29296296296296, 15.367037037037035, 16.848518518518517, 20.265185185185185, 22.357777777777777, 25.255925925925926, 29.27444444444445, 33.53370370370371, 37.95962962962963, 45.50592592592593, 51.94111111111111, 58.209629629629646, 65.83925925925928, 71.66333333333334, 79.7188888888889, 88.08000000000001, 97.94111111111111, 107.96888888888888, 117.43185185185186, 125.44111111111113, 132.60777777777778, 137.9040740740741, 141.75592592592596, 146.52444444444447, 150.58925925925928, 153.9503703703704, 158.38555555555558, 159.4318518518519, 156.79296296296297, 156.25592592592594, 153.70962962962966, 152.09851851851855, 151.48740740740743, 148.13555555555558, 143.37629629629632, 137.16333333333336, 131.97814814814816, 127.47814814814816, 121.30222222222224, 117.24666666666667, 111.97814814814815, 105.9874074074074, 100.5337037037037, 94.68185185185183, 89.12629629629629, 84.90407407407407, 81.7651851851852, 77.94111111111113, 76.8577777777778, 73.53370370370371, 70.4503703703704, 68.01518518518519, 63.487407407407424, 62.839259259259265, 59.635555555555555, 55.904074074074074, 52.95962962962963, 49.172592592592586, 47.34851851851852, 47.617037037037036, 45.95962962962963, 43.47814814814814, 42.39481481481481, 38.172592592592586, 36.06148148148148, 33.931851851851846, 32.691111111111105, 33.72814814814815, 32.22814814814815, 32.26518518518519, 30.01518518518518, 27.450370370370372, 28.73740740740741, 27.64481481481482, 26.681851851851853, 26.163333333333334, 23.357777777777773, 21.617037037037033, 20.079999999999995, 20.69111111111111, 19.848518518518517, 19.30222222222222, 20.05222222222222, 17.505925925925922, 19.357777777777777, 18.839259259259254, 16.70037037037037, 17.487407407407403, 14.496666666666663, 13.496666666666663, 14.209629629629626, 13.848518518518516, 13.67259259259259, 12.820740740740737, 9.931851851851848, 8.663333333333329, 8.05222222222222, 8.829999999999998, 11.117037037037033, 11.839259259259254, 11.42259259259259, 11.468888888888884, 10.644814814814811, 8.746666666666664, 9.079999999999997, 7.681851851851849, 6.691111111111108, 6.968888888888886, 6.728148148148144, 10.0337037037037, 9.718888888888886, 8.570740740740737, 8.061481481481477, 5.820740740740737, 6.654074074074071, 6.255925925925924, 6.589259259259256, 6.885555555555552, 6.607777777777775, 7.755925925925922, 7.552222222222219, 5.894814814814811, 6.617037037037033, 7.089259259259256, 6.848518518518516, 7.005925925925922, 6.200370370370367, 5.718888888888886, 5.524444444444441, 4.5337037037037, 3.922592592592589, 2.9688888888888854, 1.4040740740740707, 0.9966666666666635, 1.5059259259259228, 2.3670370370370337, 2.950370370370367, 3.8207407407407374, 2.5707407407407374, 1.765185185185182, 1.1818518518518486, 1.9596296296296265, 1.052222222222219, 1.4040740740740707, 2.348518518518515, 0.8485185185185152, 2.8948148148148114, 4.367037037037034, 4.876296296296293, 5.978148148148144, 7.496666666666663, 5.5337037037037, 4.765185185185182, 5.04296296296296, 2.7466666666666635, 2.802222222222219, 1.8485185185185156, 2.1818518518518486, 2.2559259259259226, 1.635555555555552, 2.5707407407407374, 1.737407407407404, 2.1170370370370337, 3.5059259259259226, 2.765185185185182, 1.7374074074074044, 1.4688888888888858, 0.06148148148147819, 0.20962962962962634, 0.8022222222222188, 0.6077777777777745, 1.6262962962962932, 2.1170370370370337, 2.357777777777774, 2.228148148148145, 2.6818518518518486, 3.144814814814812, 2.728148148148145, 3.376296296296293, 1.7374074074074042, 1.5614814814814781, 1.1170370370370337, 0.089259259259256, 1.3299999999999967, 0.66333333333333, 0.4966666666666633, 0.2837037037037003, -0.5125925925925959, 0.3948148148148115, 0.8114814814814783, 2.228148148148145, 2.91333333333333, 3.598518518518515, 3.3855555555555523, 2.7929629629629598, 1.5707407407407377, 0.9411111111111079, 0.7466666666666634, 0.8485185185185152, 1.41333333333333, 1.5337037037037005, 3.0614814814814784, 2.5337037037037002, 2.154074074074071, 0.8577777777777744, 0.13555555555555227, 0.9874074074074042, 1.7188888888888858, 2.7929629629629598, 3.922592592592589, 1.9318518518518486, 0.06148148148147814, -1.6977777777777812, -2.984814814814818, -1.8922222222222254, -1.1422222222222254, 0.27444444444444116, 0.34851851851851523, 1.191111111111108, 0.6448148148148116, 0.14481481481481165, -0.39222222222222547, -1.1422222222222254, -0.873703703703707, -0.5033333333333365, -1.4570370370370402, -2.521851851851855, -2.531111111111114, -4.355185185185189, -3.5959259259259295, -2.5681481481481514, -2.0033333333333365, -0.8922222222222255, -0.9385185185185219, -0.46629629629629965, 0.02444444444444116, 0.00592592592592267, -1.4200000000000035, -2.7348148148148184, -2.142222222222226, -2.08666666666667, -0.9477777777777812, -0.07740740740741073, -1.345925925925929, 0.07074074074073744, -0.15148148148148477, 0.00592592592592267, 1.2188888888888858, -0.049629629629632854, 0.2096296296296264, -1.4570370370370402, -1.7811111111111144, -0.5588888888888923, 0.22814814814814488, 1.4596296296296263, 0.07074074074073744, -1.2718518518518551, -2.4570370370370402, -3.08666666666667, -2.845925925925929, -2.6329629629629663, -0.2811111111111144, -1.4755555555555586, -0.6700000000000033, -1.5496296296296328, -3.9385185185185216, -2.0496296296296332, -2.8551851851851886, -0.003333333333336741, 0.5985185185185153, 1.765185185185182, 1.8299999999999965, 0.1355555555555523, 0.14481481481481168, -1.1514814814814849, -0.5311111111111144, -0.27185185185185506, 0.4411111111111079, 0.7559259259259226, 0.02444444444444116, -0.31814814814815146, -0.8274074074074108, -1.4477777777777812, -0.14222222222222558, -0.9570370370370404, -0.5774074074074107, 0.1818518518518486, -2.2070370370370402, -0.3088888888888921, -0.6422222222222256, -0.03111111111111442, 1.0707407407407374, 0.66333333333333, 0.2096296296296264, -2.5033333333333365, -0.9662962962962995, -1.1422222222222254, -0.7070370370370405, -0.20703703703704024, -0.8922222222222256, -1.660740740740744, -1.5125925925925958, -0.5588888888888921, -1.5218518518518551, -0.9940740740740773, -2.021851851851855, -1.845925925925929, -1.7255555555555588, -1.7440740740740774, -0.20703703703704035, 0.5522222222222188, 0.7837037037037005, -0.11444444444444779, -0.7533333333333367, -0.39222222222222547, -0.2533333333333367, 2.0429629629629598, 1.5799999999999965, 0.8948148148148115, 2.6448148148148114, 0.7374074074074042, 2.3299999999999965, 3.6633333333333296, 1.8577777777777746, 2.422592592592589, 0.8114814814814781, -0.0681481481481514, 1.3855555555555523, 1.1540740740740707, 0.9596296296296262, 0.34851851851851506, -0.7162962962962997, -1.8644444444444477, -1.7348148148148181, -1.4662962962962995, -1.5403703703703737, -0.6144444444444478, -1.0218518518518551, -0.9940740740740774, -2.6329629629629663, -1.5681481481481518, -0.3088888888888922, -0.2903703703703736, 0.9503703703703672, -0.873703703703707, -1.623703703703707, -1.1977777777777807, -1.9570370370370402, 1.2281481481481449, 1.8299999999999967, 1.7096296296296263, 3.42259259259259, 1.2929629629629598, 0.8207407407407376, -0.32740740740741064, -1.3922222222222254, -0.17925925925926278, -1.1422222222222256, -1.1792592592592626, 0.1540740740740707, -1.9477777777777812, -0.06814814814815146, 0.09851851851851523, -0.04037037037037361, 0.5337037037037005, 0.9781481481481449, -0.45703703703704024, -1.4940740740740772, -2.512592592592596, -4.253333333333337, -3.188518518518522, -2.4385185185185225, -2.0496296296296332, -1.5959259259259293, -0.2811111111111144, -0.4940740740740772, -0.08666666666666989, -0.5033333333333365, -1.7162962962962993, -0.9662962962962997, -1.9940740740740774, -0.8829629629629663, -1.6885185185185216, -3.225555555555559, -0.9200000000000033, -0.7718518518518551, 1.3855555555555523, 1.4966666666666633, 0.6911111111111079, 0.22814814814814485, -0.15148148148148471, 0.7188888888888856, 0.7744444444444412, 2.468888888888886, 2.3577777777777746, 0.4874074074074042, 0.45037037037036715, -0.873703703703707, -0.09592592592592908, 1.6448148148148116, 0.10777777777777442, -0.15148148148148483, -1.1977777777777812, -1.8829629629629663, -0.7533333333333365, -1.170000000000003, -0.003333333333336519, 0.1633333333333299, 1.0429629629629595, 1.8207407407407372, 0.48740740740740407, 0.4781481481481448, -0.7903703703703737, -1.984814814814818, -1.6792592592592626, -0.3274074074074107, -0.13296296296296617, 1.5985185185185151, 1.2929629629629595, -0.6700000000000034, -1.2440740740740774, -4.021851851851855, -4.021851851851856, -3.808888888888892, -1.6792592592592623, 1.3855555555555523, 1.1262962962962928, 1.9411111111111077, -1.0588888888888923, -2.771851851851855, -2.521851851851855, -2.8274074074074105, -1.2996296296296328, -2.475555555555559, -2.808888888888892, -1.2070370370370402, -1.3829629629629663, -0.9662962962962997, -2.151481481481485, -3.799629629629633, -2.901481481481485, -2.271851851851855, 0.28370370370370035, -0.19777777777778105, -1.4570370370370402, -0.2625925925925958, -3.484814814814818, -2.9940740740740774, -2.0311111111111146, -2.577407407407411, -1.1422222222222254, 0.5337037037037006, -0.18851851851852164, -0.6977777777777809, 1.6818518518518486, 0.6448148148148114, 1.0707407407407374, 1.2929629629629595, -1.410740740740744, -2.095925925925929, -0.947777777777781, -0.8829629629629662, 1.1170370370370337, 0.9874074074074042, -0.5033333333333365, 0.47814814814814494, -0.41074074074074407, 0.30222222222221895, -0.14222222222222558, -0.04037037037037372, -0.32740740740741076, 0.015185185185181749, 0.66333333333333, -0.7070370370370404, -0.47555555555555884, -0.8644444444444476, 0.9781481481481448, 1.1170370370370337, 1.922592592592589, 0.6540740740740709, -1.3644444444444477, -1.5218518518518551, -2.5033333333333365, -1.2533333333333367, -0.5866666666666699, -0.8366666666666699, -2.327407407407411, -4.095925925925929, -4.207037037037041, -4.08666666666667, -2.3551851851851886, -0.623703703703707, -0.6885185185185217, 0.5337037037037005, -0.45703703703704035, -0.18851851851852186, 0.07074074074073738, -0.9755555555555588, 0.15407407407407084, -0.2162962962962996, -0.22555555555555884, 0.7466666666666634, 1.0244444444444412, 1.6170370370370337, 0.6448148148148115, -0.30888888888889215, -1.170000000000003, -1.845925925925929, -1.9200000000000033, -2.4014814814814844, -2.8274074074074105, -2.170000000000003, -2.1237037037037068, -1.558888888888892, 0.23740740740740418, -1.0218518518518551, -1.2625925925925958, -1.3829629629629663, -1.2348148148148181, -1.2162962962962995, -1.4200000000000033, -0.8644444444444477, -3.345925925925929, -3.262592592592596, -1.6885185185185219, -2.4477777777777807, -0.8181481481481514, -0.4755555555555588, -1.1329629629629663, 0.7466666666666634, 1.8855555555555523, 1.552222222222219, 2.5151851851851816, 1.1540740740740707, 0.5799999999999966, 1.1170370370370337, -0.06814814814815151, -0.4570370370370404, -1.2348148148148181, -1.6700000000000033, -0.16074074074074407, 0.41333333333333, -0.14222222222222547, -0.6885185185185217, -2.7903703703703737, -2.1051851851851886, -0.3922222222222256, 0.5429629629629596, 1.9966666666666635, -0.15148148148148466]
  out "CH 2 Bin Readings":dbl[](array[numeric])=[302.0, 240.0, 258.0, 278.0, 271.0, 264.0, 249.0, 268.0, 276.0, 300.0, 262.0, 269.0, 256.0, 264.0, 251.0, 306.0, 248.0, 300.0, 265.0, 314.0, 325.0, 308.0, 322.0, 355.0, 351.0, 376.0, 361.0, 352.0, 359.0, 386.0, 366.0, 382.0, 359.0, 404.0, 400.0, 355.0, 377.0, 432.0, 371.0, 363.0, 367.0, 348.0, 368.0, 383.0, 357.0, 330.0, 327.0, 371.0, 348.0, 323.0, 342.0, 348.0, 331.0, 308.0, 343.0, 309.0, 323.0, 266.0, 285.0, 313.0, 307.0, 295.0, 283.0, 272.0, 275.0, 291.0, 312.0, 298.0, 254.0, 280.0, 264.0, 273.0, 260.0, 264.0, 273.0, 255.0, 277.0, 266.0, 234.0, 282.0, 276.0, 263.0, 246.0, 228.0, 245.0, 257.0, 252.0, 253.0, 257.0, 257.0, 294.0, 258.0, 246.0, 258.0, 259.0, 239.0, 270.0, 247.0, 253.0, 245.0, 256.0, 255.0, 282.0, 243.0, 227.0, 256.0, 264.0, 253.0, 245.0, 234.0, 259.0, 274.0, 272.0, 261.0, 250.0, 245.0, 251.0, 261.0, 214.0, 236.0, 240.0, 256.0, 254.0, 257.0, 256.0, 286.0, 270.0, 257.0, 249.0, 256.0, 254.0, 254.0, 233.0, 239.0, 230.0, 247.0, 238.0, 269.0, 254.0, 232.0, 247.0, 254.0, 216.0, 260.0, 269.0, 252.0, 217.0, 249.0, 243.0, 258.0, 262.0, 228.0, 257.0, 236.0, 206.0, 263.0, 224.0, 248.0, 230.0, 227.0, 263.0, 241.0, 224.0, 245.0, 247.0, 261.0, 238.0, 272.0, 249.0, 262.0, 249.0, 241.0, 232.0, 243.0, 244.0, 245.0, 268.0, 240.0, 261.0, 289.0, 261.0, 224.0, 250.0, 229.0, 229.0, 230.0, 242.0, 241.0, 269.0, 227.0, 254.0, 249.0, 241.0, 228.0, 248.0, 256.0, 238.0, 238.0, 255.0, 224.0, 237.0, 253.0, 282.0, 245.0, 230.0, 227.0, 265.0, 232.0, 245.0, 244.0, 242.0, 238.0, 262.0, 285.0, 211.0, 252.0, 249.0, 248.0, 227.0, 216.0, 278.0, 220.0, 238.0, 238.0, 230.0, 247.0, 218.0, 249.0, 237.0, 255.0, 217.0, 270.0, 238.0, 215.0, 252.0, 247.0, 236.0, 225.0, 254.0, 233.0, 221.0, 258.0, 251.0, 251.0, 228.0, 249.0, 259.0, 250.0, 245.0, 233.0, 249.0, 250.0, 222.0, 263.0, 243.0, 245.0, 224.0, 216.0, 222.0, 242.0, 246.0, 242.0, 235.0, 241.0, 262.0, 231.0, 219.0, 228.0, 246.0, 234.0, 223.0, 223.0, 233.0, 241.0, 239.0, 224.0, 216.0, 242.0, 220.0, 235.0, 233.0, 251.0, 217.0, 216.0, 230.0, 233.0, 251.0, 250.0, 260.0, 240.0, 244.0, 257.0, 258.0, 234.0, 274.0, 271.0, 221.0, 227.0, 255.0, 257.0, 218.0, 257.0, 239.0, 233.0, 245.0, 215.0, 234.0, 237.0, 223.0, 245.0, 251.0, 210.0, 212.0, 259.0, 249.0, 232.0, 235.0, 227.0, 258.0, 238.0, 243.0, 223.0, 244.0, 220.0, 221.0, 232.0, 264.0, 248.0, 247.0, 225.0, 237.0, 267.0, 241.0, 239.0, 209.0, 228.0, 219.0, 237.0, 248.0, 235.0, 248.0, 225.0, 231.0, 238.0, 259.0, 259.0, 244.0, 229.0, 222.0, 245.0, 261.0, 231.0, 234.0, 249.0, 215.0, 233.0, 242.0, 252.0, 256.0, 253.0, 247.0, 225.0, 204.0, 263.0, 236.0, 256.0, 235.0, 231.0, 242.0, 225.0, 270.0, 263.0, 286.0, 243.0, 249.0, 244.0, 251.0, 233.0, 244.0, 224.0, 252.0, 226.0, 245.0, 247.0, 259.0, 212.0, 283.0, 268.0, 264.0, 246.0, 253.0, 243.0, 246.0, 239.0, 205.0, 255.0, 236.0, 222.0, 233.0, 207.0, 220.0, 237.0, 230.0, 238.0, 236.0, 225.0, 238.0, 212.0, 221.0, 219.0, 266.0, 249.0, 215.0, 232.0, 228.0, 221.0, 225.0, 249.0, 230.0, 230.0, 256.0, 251.0, 237.0, 229.0, 225.0, 266.0, 252.0, 263.0, 239.0, 231.0, 230.0, 244.0, 245.0, 227.0, 239.0, 225.0, 228.0, 253.0, 267.0, 228.0, 253.0, 244.0, 236.0, 242.0, 218.0, 248.0, 211.0, 235.0, 224.0, 238.0, 259.0, 277.0, 259.0, 240.0, 258.0, 267.0, 245.0, 252.0, 245.0, 232.0, 244.0, 247.0, 238.0, 273.0, 250.0, 221.0, 223.0, 243.0, 255.0, 230.0, 242.0, 243.0, 242.0, 232.0, 241.0, 267.0, 237.0, 240.0, 242.0, 218.0, 235.0, 247.0, 273.0, 228.0, 227.0, 244.0, 222.0, 259.0, 224.0, 232.0, 277.0, 224.0, 217.0, 227.0, 219.0, 238.0, 244.0, 240.0, 251.0, 240.0, 270.0, 238.0, 227.0, 240.0, 229.0, 243.0, 239.0, 216.0, 224.0, 235.0, 244.0, 249.0, 249.0, 260.0, 220.0, 223.0, 255.0, 246.0, 251.0, 240.0, 220.0, 220.0, 242.0, 271.0, 244.0, 245.0, 230.0, 247.0, 275.0, 232.0, 241.0, 224.0, 238.0, 245.0, 260.0, 256.0, 243.0, 245.0, 234.0, 220.0, 241.0, 227.0, 248.0, 225.0, 259.0, 240.0, 218.0, 266.0, 259.0, 232.0, 246.0, 218.0, 252.0, 247.0, 254.0, 257.0, 271.0, 240.0, 261.0]
  in  "stop":bool
  in  "Reset Average":bool=TRUE
  in  "Save Data?":bool=TRUE
  in  "Collect Data?":bool=TRUE
  in  "ILX Address":i32=6 min=0 step=1
  in  "Lambda On DBR Current":dbl=171.13999999999868
  in  "Lambda Off DBR Current":dbl=172.9499999999997
  in  "Tab Control":T2(tab)=enum."OD"
  out "NRB plot":cluster{"Y":dbl[], "Y":dbl[]}[](graph)=[{"Y"=[], "Y"=[0.0375, 0.075, 0.11249999999999999, 0.15, 0.1875, 0.225, 0.26249999999999996, 0.3, 0.33749999999999997, 0.37499999999999994, 0.4125, 0.44999999999999996, 0.48749999999999993, 0.525, 0.5625, 0.6, 0.6375, 0.6749999999999999, 0.7124999999999999, 0.75, 0.7875, 0.825, 0.8624999999999999, 0.8999999999999999, 0.9374999999999999, 0.975, 1.0125, 1.05, 1.0875000000000001, 1.125, 1.1625, 1.2, 1.2375, 1.2750000000000001, 1.3125, 1.35, 1.3875, 1.425, 1.4625000000000001, 1.5, 1.5375, 1.575, 1.6125, 1.6500000000000001, 1.6875, 1.725, 1.7625, 1.8, 1.8375, 1.875, 1.9125, 1.95, 1.9875, 2.025, 2.0625, 2.1, 2.1375, 2.175, 2.2125, 2.25, 2.2875, 2.325, 2.3625, 2.4, 2.4375, 2.475, 2.5125, 2.55, 2.5875, 2.625, 2.6625, 2.7, 2.7375, 2.775, 2.8125, 2.85, 2.8875, 2.925, 2.9625, 3.0, 3.0375, 3.075, 3.1125, 3.15, 3.1875, 3.225, 3.2625, 3.3, 3.3375, 3.375, 3.4125, 3.45, 3.4875, 3.525, 3.5625, 3.6, 3.6374999999999997, 3.675, 3.7125, 3.75, 3.7875, 3.8249999999999997, 3.8625, 3.9, 3.9375, 3.975, 4.012499999999999, 4.05, 4.0874999999999995, 4.124999999999999, 4.1625, 4.199999999999999, 4.2375, 4.2749999999999995, 4.312499999999999, 4.35, 4.387499999999999, 4.425, 4.4624999999999995, 4.499999999999999, 4.5375, 4.574999999999999, 4.6125, 4.6499999999999995, 4.687499999999999, 4.725, 4.762499999999999, 4.8, 4.8374999999999995, 4.874999999999999, 4.9125, 4.949999999999999, 4.9875, 5.0249999999999995, 5.062499999999999, 5.1, 5.137499999999999, 5.175, 5.2124999999999995, 5.249999999999999, 5.2875, 5.324999999999999, 5.3625, 5.3999999999999995, 5.437499999999999, 5.475, 5.512499999999999, 5.55, 5.5874999999999995, 5.624999999999999, 5.6625, 5.699999999999999, 5.7375, 5.7749999999999995, 5.812499999999999, 5.85, 5.887499999999999, 5.925, 5.9624999999999995, 5.999999999999999, 6.0375, 6.074999999999999, 6.1125, 6.1499999999999995, 6.187499999999999, 6.225, 6.262499999999999, 6.3, 6.3374999999999995, 6.374999999999999, 6.4125, 6.449999999999999, 6.4875, 6.5249999999999995, 6.562499999999999, 6.6, 6.637499999999999, 6.675, 6.7124999999999995, 6.749999999999999, 6.7875, 6.824999999999999, 6.8625, 6.8999999999999995, 6.937499999999999, 6.975, 7.012499999999999, 7.05, 7.0874999999999995, 7.124999999999999, 7.1625, 7.199999999999999, 7.237499999999999, 7.2749999999999995, 7.312499999999999, 7.35, 7.387499999999999, 7.424999999999999, 7.4624999999999995, 7.499999999999999, 7.5375, 7.574999999999999, 7.612499999999999, 7.6499999999999995, 7.687499999999999, 7.725, 7.762499999999999, 7.799999999999999, 7.8374999999999995, 7.874999999999999, 7.9125, 7.949999999999999, 7.987499999999999, 8.025, 8.0625, 8.1, 8.1375, 8.174999999999999, 8.212499999999999, 8.25, 8.2875, 8.325, 8.362499999999999, 8.399999999999999, 8.4375, 8.475, 8.5125, 8.549999999999999, 8.587499999999999, 8.625, 8.6625, 8.7, 8.737499999999999, 8.774999999999999, 8.8125, 8.85, 8.8875, 8.924999999999999, 8.962499999999999, 9.0, 9.0375, 9.075, 9.112499999999999, 9.149999999999999, 9.1875, 9.225, 9.2625, 9.299999999999999, 9.337499999999999, 9.375, 9.4125, 9.45, 9.487499999999999, 9.524999999999999, 9.5625, 9.6, 9.6375, 9.674999999999999, 9.712499999999999, 9.75, 9.7875, 9.825, 9.862499999999999, 9.899999999999999, 9.9375, 9.975, 10.0125, 10.049999999999999, 10.087499999999999, 10.125, 10.1625, 10.2, 10.237499999999999, 10.274999999999999, 10.3125, 10.35, 10.3875, 10.424999999999999, 10.462499999999999, 10.5, 10.5375, 10.575, 10.612499999999999, 10.649999999999999, 10.6875, 10.725, 10.7625, 10.799999999999999, 10.837499999999999, 10.875, 10.9125, 10.95, 10.987499999999999, 11.024999999999999, 11.0625, 11.1, 11.1375, 11.174999999999999, 11.212499999999999, 11.25, 11.2875, 11.325, 11.362499999999999, 11.399999999999999, 11.4375, 11.475, 11.5125, 11.549999999999999, 11.587499999999999, 11.625, 11.6625, 11.7, 11.737499999999999, 11.774999999999999, 11.8125, 11.85, 11.8875, 11.924999999999999, 11.962499999999999, 12.0, 12.0375, 12.075, 12.112499999999999, 12.149999999999999, 12.1875, 12.225, 12.2625, 12.299999999999999, 12.337499999999999, 12.375, 12.4125, 12.45, 12.487499999999999, 12.524999999999999, 12.5625, 12.6, 12.6375, 12.674999999999999, 12.712499999999999, 12.75, 12.7875, 12.825, 12.862499999999999, 12.899999999999999, 12.9375, 12.975, 13.0125, 13.049999999999999, 13.087499999999999, 13.125, 13.1625, 13.2, 13.237499999999999, 13.274999999999999, 13.3125, 13.35, 13.3875, 13.424999999999999, 13.462499999999999, 13.5, 13.5375, 13.575, 13.612499999999999, 13.649999999999999, 13.6875, 13.725, 13.7625, 13.799999999999999, 13.837499999999999, 13.875, 13.9125, 13.95, 13.987499999999999, 14.024999999999999, 14.0625, 14.1, 14.1375, 14.174999999999999, 14.212499999999999, 14.25, 14.2875, 14.325, 14.362499999999999, 14.399999999999999, 14.437499999999998, 14.475, 14.5125, 14.549999999999999, 14.587499999999999, 14.624999999999998, 14.6625, 14.7, 14.737499999999999, 14.774999999999999, 14.812499999999998, 14.85, 14.8875, 14.924999999999999, 14.962499999999999, 14.999999999999998, 15.0375, 15.075, 15.112499999999999, 15.149999999999999, 15.187499999999998, 15.225, 15.2625, 15.299999999999999, 15.337499999999999, 15.374999999999998, 15.4125, 15.45, 15.487499999999999, 15.524999999999999, 15.562499999999998, 15.6, 15.6375, 15.674999999999999, 15.712499999999999, 15.749999999999998, 15.7875, 15.825, 15.862499999999999, 15.899999999999999, 15.937499999999998, 15.975, 16.0125, 16.05, 16.087500000000002, 16.125, 16.1625, 16.2, 16.2375, 16.275000000000002, 16.3125, 16.35, 16.3875, 16.425, 16.462500000000002, 16.5, 16.5375, 16.575, 16.6125, 16.650000000000002, 16.6875, 16.725, 16.7625, 16.8, 16.837500000000002, 16.875, 16.9125, 16.95, 16.9875, 17.025000000000002, 17.0625, 17.1, 17.1375, 17.175, 17.212500000000002, 17.25, 17.2875, 17.325, 17.3625, 17.400000000000002, 17.4375, 17.475, 17.5125, 17.55, 17.587500000000002, 17.625, 17.6625, 17.7, 17.7375, 17.775000000000002, 17.8125, 17.85, 17.8875, 17.925, 17.962500000000002, 18.0, 18.0375, 18.075, 18.1125, 18.150000000000002, 18.1875, 18.225, 18.2625, 18.3, 18.337500000000002, 18.375, 18.4125, 18.45, 18.4875, 18.525000000000002, 18.5625, 18.6, 18.6375, 18.675, 18.712500000000002, 18.75, 18.7875, 18.825, 18.8625, 18.900000000000002, 18.9375, 18.975, 19.0125, 19.05, 19.087500000000002, 19.125, 19.1625, 19.2, 19.2375, 19.275000000000002, 19.3125, 19.35, 19.3875, 19.425, 19.462500000000002, 19.5, 19.5375, 19.575, 19.6125, 19.650000000000002, 19.6875, 19.725, 19.7625, 19.8, 19.837500000000002, 19.875, 19.9125, 19.95, 19.9875, 20.025000000000002, 20.0625, 20.1, 20.1375, 20.175, 20.212500000000002, 20.25, 20.2875, 20.325, 20.3625, 20.400000000000002, 20.4375, 20.475, 20.5125, 20.55, 20.587500000000002, 20.625, 20.6625, 20.7, 20.7375, 20.775000000000002, 20.8125, 20.85, 20.8875, 20.925, 20.962500000000002, 21.0]}, ...(2 in all)]
  in  "background length":i32=25
  out "Correction":cluster{"Y":dbl[], "Y":dbl[]}[](graph)=[{"Y"=[], "Y"=[0.0375, 0.075, 0.11249999999999999, 0.15, 0.1875, 0.225, 0.26249999999999996, 0.3, 0.33749999999999997, 0.37499999999999994, 0.4125, 0.44999999999999996, 0.48749999999999993, 0.525, 0.5625, 0.6, 0.6375, 0.6749999999999999, 0.7124999999999999, 0.75, 0.7875, 0.825, 0.8624999999999999, 0.8999999999999999, 0.9374999999999999, 0.975, 1.0125, 1.05, 1.0875000000000001, 1.125, 1.1625, 1.2, 1.2375, 1.2750000000000001, 1.3125, 1.35, 1.3875, 1.425, 1.4625000000000001, 1.5, 1.5375, 1.575, 1.6125, 1.6500000000000001, 1.6875, 1.725, 1.7625, 1.8, 1.8375, 1.875, 1.9125, 1.95, 1.9875, 2.025, 2.0625, 2.1, 2.1375, 2.175, 2.2125, 2.25, 2.2875, 2.325, 2.3625, 2.4, 2.4375, 2.475, 2.5125, 2.55, 2.5875, 2.625, 2.6625, 2.7, 2.7375, 2.775, 2.8125, 2.85, 2.8875, 2.925, 2.9625, 3.0, 3.0375, 3.075, 3.1125, 3.15, 3.1875, 3.225, 3.2625, 3.3, 3.3375, 3.375, 3.4125, 3.45, 3.4875, 3.525, 3.5625, 3.6, 3.6374999999999997, 3.675, 3.7125, 3.75, 3.7875, 3.8249999999999997, 3.8625, 3.9, 3.9375, 3.975, 4.012499999999999, 4.05, 4.0874999999999995, 4.124999999999999, 4.1625, 4.199999999999999, 4.2375, 4.2749999999999995, 4.312499999999999, 4.35, 4.387499999999999, 4.425, 4.4624999999999995, 4.499999999999999, 4.5375, 4.574999999999999, 4.6125, 4.6499999999999995, 4.687499999999999, 4.725, 4.762499999999999, 4.8, 4.8374999999999995, 4.874999999999999, 4.9125, 4.949999999999999, 4.9875, 5.0249999999999995, 5.062499999999999, 5.1, 5.137499999999999, 5.175, 5.2124999999999995, 5.249999999999999, 5.2875, 5.324999999999999, 5.3625, 5.3999999999999995, 5.437499999999999, 5.475, 5.512499999999999, 5.55, 5.5874999999999995, 5.624999999999999, 5.6625, 5.699999999999999, 5.7375, 5.7749999999999995, 5.812499999999999, 5.85, 5.887499999999999, 5.925, 5.9624999999999995, 5.999999999999999, 6.0375, 6.074999999999999, 6.1125, 6.1499999999999995, 6.187499999999999, 6.225, 6.262499999999999, 6.3, 6.3374999999999995, 6.374999999999999, 6.4125, 6.449999999999999, 6.4875, 6.5249999999999995, 6.562499999999999, 6.6, 6.637499999999999, 6.675, 6.7124999999999995, 6.749999999999999, 6.7875, 6.824999999999999, 6.8625, 6.8999999999999995, 6.937499999999999, 6.975, 7.012499999999999, 7.05, 7.0874999999999995, 7.124999999999999, 7.1625, 7.199999999999999, 7.237499999999999, 7.2749999999999995, 7.312499999999999, 7.35, 7.387499999999999, 7.424999999999999, 7.4624999999999995, 7.499999999999999, 7.5375, 7.574999999999999, 7.612499999999999, 7.6499999999999995, 7.687499999999999, 7.725, 7.762499999999999, 7.799999999999999, 7.8374999999999995, 7.874999999999999, 7.9125, 7.949999999999999, 7.987499999999999, 8.025, 8.0625, 8.1, 8.1375, 8.174999999999999, 8.212499999999999, 8.25, 8.2875, 8.325, 8.362499999999999, 8.399999999999999, 8.4375, 8.475, 8.5125, 8.549999999999999, 8.587499999999999, 8.625, 8.6625, 8.7, 8.737499999999999, 8.774999999999999, 8.8125, 8.85, 8.8875, 8.924999999999999, 8.962499999999999, 9.0, 9.0375, 9.075, 9.112499999999999, 9.149999999999999, 9.1875, 9.225, 9.2625, 9.299999999999999, 9.337499999999999, 9.375, 9.4125, 9.45, 9.487499999999999, 9.524999999999999, 9.5625, 9.6, 9.6375, 9.674999999999999, 9.712499999999999, 9.75, 9.7875, 9.825, 9.862499999999999, 9.899999999999999, 9.9375, 9.975, 10.0125, 10.049999999999999, 10.087499999999999, 10.125, 10.1625, 10.2, 10.237499999999999, 10.274999999999999, 10.3125, 10.35, 10.3875, 10.424999999999999, 10.462499999999999, 10.5, 10.5375, 10.575, 10.612499999999999, 10.649999999999999, 10.6875, 10.725, 10.7625, 10.799999999999999, 10.837499999999999, 10.875, 10.9125, 10.95, 10.987499999999999, 11.024999999999999, 11.0625, 11.1, 11.1375, 11.174999999999999, 11.212499999999999, 11.25, 11.2875, 11.325, 11.362499999999999, 11.399999999999999, 11.4375, 11.475, 11.5125, 11.549999999999999, 11.587499999999999, 11.625, 11.6625, 11.7, 11.737499999999999, 11.774999999999999, 11.8125, 11.85, 11.8875, 11.924999999999999, 11.962499999999999, 12.0, 12.0375, 12.075, 12.112499999999999, 12.149999999999999, 12.1875, 12.225, 12.2625, 12.299999999999999, 12.337499999999999, 12.375, 12.4125, 12.45, 12.487499999999999, 12.524999999999999, 12.5625, 12.6, 12.6375, 12.674999999999999, 12.712499999999999, 12.75, 12.7875, 12.825, 12.862499999999999, 12.899999999999999, 12.9375, 12.975, 13.0125, 13.049999999999999, 13.087499999999999, 13.125, 13.1625, 13.2, 13.237499999999999, 13.274999999999999, 13.3125, 13.35, 13.3875, 13.424999999999999, 13.462499999999999, 13.5, 13.5375, 13.575, 13.612499999999999, 13.649999999999999, 13.6875, 13.725, 13.7625, 13.799999999999999, 13.837499999999999, 13.875, 13.9125, 13.95, 13.987499999999999, 14.024999999999999, 14.0625, 14.1, 14.1375, 14.174999999999999, 14.212499999999999, 14.25, 14.2875, 14.325, 14.362499999999999, 14.399999999999999, 14.437499999999998, 14.475, 14.5125, 14.549999999999999, 14.587499999999999, 14.624999999999998, 14.6625, 14.7, 14.737499999999999, 14.774999999999999, 14.812499999999998, 14.85, 14.8875, 14.924999999999999, 14.962499999999999, 14.999999999999998, 15.0375, 15.075, 15.112499999999999, 15.149999999999999, 15.187499999999998, 15.225, 15.2625, 15.299999999999999, 15.337499999999999, 15.374999999999998, 15.4125, 15.45, 15.487499999999999, 15.524999999999999, 15.562499999999998, 15.6, 15.6375, 15.674999999999999, 15.712499999999999, 15.749999999999998, 15.7875, 15.825, 15.862499999999999, 15.899999999999999, 15.937499999999998, 15.975, 16.0125, 16.05, 16.087500000000002, 16.125, 16.1625, 16.2, 16.2375, 16.275000000000002, 16.3125, 16.35, 16.3875, 16.425, 16.462500000000002, 16.5, 16.5375, 16.575, 16.6125, 16.650000000000002, 16.6875, 16.725, 16.7625, 16.8, 16.837500000000002, 16.875, 16.9125, 16.95, 16.9875, 17.025000000000002, 17.0625, 17.1, 17.1375, 17.175, 17.212500000000002, 17.25, 17.2875, 17.325, 17.3625, 17.400000000000002, 17.4375, 17.475, 17.5125, 17.55, 17.587500000000002, 17.625, 17.6625, 17.7, 17.7375, 17.775000000000002, 17.8125, 17.85, 17.8875, 17.925, 17.962500000000002, 18.0, 18.0375, 18.075, 18.1125, 18.150000000000002, 18.1875, 18.225, 18.2625, 18.3, 18.337500000000002, 18.375, 18.4125, 18.45, 18.4875, 18.525000000000002, 18.5625, 18.6, 18.6375, 18.675, 18.712500000000002, 18.75, 18.7875, 18.825, 18.8625, 18.900000000000002, 18.9375, 18.975, 19.0125, 19.05, 19.087500000000002, 19.125, 19.1625, 19.2, 19.2375, 19.275000000000002, 19.3125, 19.35, 19.3875, 19.425, 19.462500000000002, 19.5, 19.5375, 19.575, 19.6125, 19.650000000000002, 19.6875, 19.725, 19.7625, 19.8, 19.837500000000002, 19.875, 19.9125, 19.95, 19.9875, 20.025000000000002, 20.0625, 20.1, 20.1375, 20.175, 20.212500000000002, 20.25, 20.2875, 20.325, 20.3625, 20.400000000000002, 20.4375, 20.475, 20.5125, 20.55, 20.587500000000002, 20.625, 20.6625, 20.7, 20.7375, 20.775000000000002, 20.8125, 20.85, 20.8875, 20.925, 20.962500000000002, 21.0]}, ...(2 in all)]
  in  "dead time":dbl=3.7e-08
  out "CH1 RingBuffer long":dbl[][](array[numeric])
  out "CH1 RingBuffer short":dbl[][](array[numeric])
  in  "Weather":T3(tab)=enum."Pulse Energy (Micro Joule)"
  out "Temperature (C)":dbl(graph)=25.047466422466428
  out "Pressure (mb)":dbl(graph)=836.4285714285714
  out "Relative Humdity (%)":dbl(graph)=19.406288156288156
  out "Pulse Energy (Micro Joule)":T4(graph)={"Online Pulse Energy"=5.150377142857143, "Pulse Energy Offline"=5.149567142857142}
  out "?":cluster{"mean":dbl, "mean":dbl}(graph)={"mean"=9486.874343717187, "mean"=106774.93874693735}
  out "Index":i32=27
  out "CH1 (WV off) smooth L":dbl[](array[numeric])=[35.98431137724552, 30.072634730538933, 28.075628742514983, 27.2702395209581, 27.622035928143728, 29.193892215568876, 30.83161676646708, 33.14299401197606, 36.39149700598802, 40.587604790419164, 45.54419161676646, 52.31664670658683, 60.18191616766468, 68.84359281437128, 79.6624550898204, 91.78520958083837, 105.48580838323355, 120.41694610778444, 137.1804191616766, 155.6834131736526, 175.8076646706586, 197.31814371257474, 218.71035928143704, 239.6579640718562, 259.5531736526945, 277.86604790419153, 294.18940119760475, 310.17592814371255, 322.60556886227545, 333.04119760479045, 342.1564670658683, 346.40946107784436, 349.0307185628743, 348.75227544910183, 343.78520958083834, 337.0546706586827, 327.3405988023953, 315.1834131736527, 303.05467065868265, 289.4139520958083, 278.2747305389221, 267.6669461077843, 257.9723353293412, 248.45886227544898, 237.50077844311366, 226.1414970059879, 214.37502994011965, 202.59658682634714, 189.211856287425, 175.33610778443102, 161.62952095808373, 148.89449101796401, 139.81065868263465, 132.8735329341317, 126.78371257485026, 121.6968862275449, 114.84359281437128, 108.6130538922156, 102.28970059880244, 96.20586826347309, 91.58161676646712, 86.68491017964078, 82.71784431137729, 79.08610778443119, 75.8181437125749, 73.13401197604794, 70.55167664670664, 68.44838323353298, 66.09209580838328, 63.900479041916206, 61.65197604790423, 59.00676646706589, 56.90497005988025, 54.06215568862275, 51.57862275449101, 49.09958083832334, 46.62053892215568, 45.03221556886226, 43.20886227544909, 41.731317365269454, 40.18341317365269, 38.88850299401197, 38.01425149700599, 37.19389221556887, 36.15796407185629, 34.90946107784432, 33.366047904191625, 31.518742514970068, 29.452874251497015, 27.91694610778444, 26.634011976047912, 25.548682634730543, 24.851077844311384, 23.915449101796412, 22.451377245508993, 21.385508982035937, 20.312155688622763, 19.193892215568873, 18.677425149700603, 17.973832335329345, 17.491796407185632, 17.340598802395213, 17.253772455089823, 17.084610778443118, 16.768742514970064, 16.240299401197607, 15.330119760479043, 15.023233532934135, 14.433413173652696, 13.909461077844313, 13.470838323353295, 13.16994011976048, 13.147485029940121, 12.979820359281437, 12.575628742514972, 11.7837125748503, 11.03071856287425, 10.755269461077843, 10.613053892215566, 10.798682634730536, 10.804670658682634, 10.574131736526946, 10.687904191616767, 10.291197604790417, 10.276227544910178, 9.821137724550896, 9.366047904191614, 9.126526946107782, 8.668443113772453, 8.55766467065868, 8.593592814371256, 8.50826347305389, 8.244790419161674, 8.2088622754491, 7.672934131736525, 7.514251497005985, 7.469341317365267, 7.108562874251494, 7.0651497005988, 6.804670658682633, 6.66694610778443, 6.8091616766467045, 6.8286227544910165, 6.677425149700597, 6.634011976047902, 6.297185628742514, 6.0771257485029935, 6.220838323353293, 5.90497005988024, 5.909461077844311, 5.651976047904191, 5.2103592814371265, 5.110059880239521, 5.0741317365269465, 5.0531736526946105, 5.1429940119760476, 4.9603592814371265, 4.544191616766467, 4.404970059880238, 4.304670658682634, 4.23880239520958, 4.207365269461078, 4.141497005988024, 3.8765269461077843, 3.8450898203592816, 4.018742514970061, 4.069640718562875, 3.952874251497006, 3.916946107784431, 3.842095808383233, 3.777724550898203, 3.66694610778443, 3.8196407185628733, 3.8450898203592807, 3.5067664670658676, 3.6190419161676637, 3.583113772455089, 3.1968862275449093, 3.4154491017964057, 3.4274251497005976, 3.1968862275449093, 3.1684431137724545, 3.268742514970059, 3.0142514970059873, 2.9633532934131726, 3.0052694610778437, 3.06065868263473, 2.994790419161676, 3.0935928143712568, 2.9648502994011965, 2.68191616766467, 2.6968862275449093, 2.5666467065868255, 2.599580838323352, 2.3765269461077834, 2.3555688622754483, 2.4004790419161663, 2.1414970059880227, 2.2507784431137714, 2.23880239520958, 2.2178443113772444, 2.3376047904191606, 2.261257485029939, 2.2477844311377235, 2.2388023952095795, 2.2807185628742506, 2.12502994011976, 2.277724550898203, 2.190898203592814, 2.1968862275449097, 2.12502994011976, 1.9304191616766462, 1.8196407185628736, 1.7971856287425148, 1.7702395209580832, 1.916946107784431, 1.8046706586826347, 1.653473053892215, 1.8121556886227541, 1.8001796407185622, 1.741796407185628, 1.8570658682634726, 1.7642514970059875, 1.5636526946107783, 1.481317365269461, 1.2268263473053889, 1.0546706586826344, 1.0097604790419161, 1.168443113772455, 1.2597604790419161, 1.4678443113772452, 1.1789221556886225, 1.225329341317365, 1.3645508982035925, 1.2627544910179638, 1.5531736526946105, 1.346586826347305, 1.3929940119760476, 1.5127544910179638, 1.1504790419161672, 1.1774251497005983, 1.0202395209580835, 0.8989820359281435, 1.0262275449101796, 0.7986826347305388, 0.8465868263473052, 0.7552694610778441, 1.0831137724550894, 1.3376047904191615, 1.1908982035928144, 1.2986826347305387, 0.978323353293413, 0.9528742514970058, 0.8899999999999997, 0.9453892215568861, 1.1894011976047902, 1.0831137724550897, 1.1953892215568862, 1.0801197604790418, 0.7028742514970058, 0.973832335329341, 0.9588622754491013, 1.0127544910179638, 1.225329341317365, 1.3346107784431136, 1.3091616766467062, 1.2956886227544908, 1.5486826347305385, 1.4034730538922155, 1.357065868263473, 1.1489820359281435, 0.858562874251497, 0.7328143712574848, 0.7388023952095806, 0.8106586826347302, 0.8316167664670655, 0.6684431137724549, 0.6594610778443113, 0.6804191616766467, 0.6265269461077844, 0.8615568862275447, 0.6564670658682631, 0.6834131736526944, 0.822634730538922, 0.6579640718562875, 0.8181437125748504, 0.8226347305389221, 0.6310179640718562, 0.6100598802395207, 0.7163473053892213, 0.6399999999999998, 0.5277245508982035, 0.49479041916167643, 0.2702395209580836, 0.46035928143712546, 0.5292215568862272, 0.6175449101796404, 0.698383233532934, 0.6145508982035925, 0.6040718562874251, 0.34209580838323345, 0.3450898203592813, 0.3720359281437122, 0.31365269461077816, 0.5531736526946105, 0.5112574850299398, 0.2717365269461078, 0.1879041916167664, 0.105568862275449, 0.04119760479041901, 0.442395209580838, 0.7986826347305387, 0.7986826347305388, 0.5771257485029938, 0.42742514970059875, 0.28820359281437113, 0.49628742514970053, 0.8600598802395207, 0.7777245508982034, 0.7627544910179639, 0.3615568862275447, 0.22682634730538914, 0.2822155688622754, 0.2268263473053892, 0.5292215568862275, 0.40497005988023943, 0.27323353293413155, 0.44988023952095796, 0.26425149700598793, 0.18341317365269463, 0.0382035928143713, -0.30910179640718566, -0.21628742514970073, -0.05610778443113795, -0.11000000000000021, 0.1819161676646705, 0.15646706586826342, 0.27473053892215565, 0.6235329341317366, 0.3705389221556885, 0.23431137724550888, 0.2807185628742514, 0.16844311377245505, 0.041197604790419035, -0.039640718562874405, -0.2806586826347307, -0.44532934131736557, -0.23275449101796422, -0.4034131736526949, -0.25970059880239554, -0.121976047904192, 0.0441916167664666, 0.3885029940119758, 0.5112574850299397, 0.35856287425149663, -0.10101796407185654, -0.21029940119760507, -0.28964071856287443, -0.2881437125748505, 0.10556886227544894, 0.26125748502994006, 0.11904191616766456, 0.18491017964071849, 0.07263473053892204, 0.03520958083832323, 0.25377245508982027, -0.005209580838323458, 0.16994011976047896, 0.026227544910179437, -0.4138922155688625, -0.16239520958083853, -0.3150898203592818, -0.11898203592814396, 0.07862275449101772, -0.05760479041916185, 0.13101796407185623, 0.13999999999999996, 0.10107784431137722, 0.37652694610778437, 0.31215568862275445, 0.1639520958083832, 0.33161676646706584, 0.048682634730538826, -0.030658682634730622, -0.009700598802395311, -0.12497005988023957, 0.138502994011976, 0.009760479041916167, 0.06814371257485029, 0.30467065868263465, 0.19389221556886221, 0.4558682634730538, 0.3450898203592813, 0.19239520958083822, 0.34658682634730514, -0.06808383233532964, -0.026167664670658917, -0.06359281437125772, -0.3315568862275451, -0.1489221556886229, -0.22077844311377265, -0.11748502994011994, -0.0800598802395211, -0.12197604790419167, -0.04113772455089824, -0.06359281437125752, 0.033712574850299354, 0.4094610778443113, 0.3465868263473053, 0.14898203592814369, 0.13401197604790413, -0.08155688622754495, -0.10550898203592819, -0.07706586826347316, -0.03964071856287435, -0.030658682634730636, 0.16994011976047893, 0.38101796407185623, 0.43191616766467056, 0.24179640718562861, 0.23880239520958074, 0.030718562874251343, -0.0950299401197606, 0.09209580838323334, -0.1848502994011978, -0.12347305389221573, -0.04562874251497022, -0.30910179640718577, -0.16389221556886238, -0.04263473053892228, -0.43335329341317375, -0.04712574850299417, 0.018742514970059687, -0.11748502994011997, 0.23580838323353276, 0.16694610778443103, 0.26125748502994, 0.4603592814371257, 0.26125748502994006, -0.01568862275449112, -0.06359281437125751, -0.19982035928143718, 0.005269461077844241, 0.24179640718562864, 0.11005988023952086, -0.014191616766467144, -0.06808383233532944, -0.17886227544910188, -0.15640718562874267, 0.08910179640718545, 0.2343113772455087, 0.11904191616766438, 0.26275449101796383, 0.32113772455089806, 0.15197604790419156, 0.35107784431137723, 0.36005988023952085, 0.11305389221556875, 0.1385029940119759, -0.1234730538922156, -0.27017964071856293, 0.07113772455089817, 0.2852095808383233, 0.2507784431137724, 0.2657485029940119, -0.08754491017964078, -0.16988023952095804, -0.11149700598802394, -0.17586826347305384, -0.24772455089820355, -0.28514970059880246, -0.20131736526946115, -0.06658682634730548, -0.029161676646706727, -0.33455089820359296, -0.3016167664670661, -0.3914371257485032, -0.06808383233532952, 0.27622754491017953, 0.4917964071856288, 0.5097604790419161, 0.08461077844311374, -0.16089820359281443, -0.2582035928143714, -0.33604790419161695, -0.19532934131736546, 0.003772455089820159, 0.04119760479041894, 0.21784431137724536, 0.32413173652694605, 0.4079640718562873, 0.26874251497005974, 0.25826347305389213, 0.2088622754491017, 0.20437125748502985, 0.17592814371257479, -0.0037125748502994382, 0.2163473053892215, -0.041137724550898286, 0.02473053892215556, 0.3136526946107784, 0.19538922155688618, 0.5576646706586826, 0.5591616766467067, 0.5247305389221557, 0.4783233532934132, 0.005269461077844317, 0.0681437125748503, 0.20437125748502988, 0.16694610778443109, 0.45137724550898195, 0.6534730538922155, 0.5037724550898204, 0.6160479041916167, 0.6070658682634731, 0.24329341317365255, 0.31365269461077816, 0.2522754491017962, 0.442395209580838, 0.596586826347305, 0.3570658682634728, 0.3046706586826345, -0.1878443113772457, -0.395928143712575, -0.5755688622754493, -0.6564071856287428, -0.46029940119760504, -0.25221556886227564, -0.09802395209580855, -0.10700598802395223, -0.17736526946107792, -0.2896407185628743, -0.2147904191616768, -0.1638922155688624, -0.05610778443113789, 0.027724550898203432, 0.16994011976047893, 0.23281437125748494, 0.15347305389221538, 0.029221556886227393, -0.11598802395209594, -0.1743712574850301, 0.06964071856287415, 0.25676646706586814, 0.33311377245508966, 0.4229341317365268, 0.2971856287425148, 0.2073652694610777, 0.1624550898203592, 0.1519760479041915, 0.3585628742514969, 0.20437125748502985, -0.020179640718562986, -0.22526946107784446, -0.7327544910179642]
  out "CH1  Bin Readings":dbl[](array[numeric])=[106.0, 95.0, 81.0, 69.0, 78.0, 63.0, 89.0, 95.0, 81.0, 84.0, 89.0, 86.0, 102.0, 101.0, 124.0, 150.0, 156.0, 177.0, 223.0, 255.0, 263.0, 312.0, 306.0, 371.0, 385.0, 418.0, 425.0, 440.0, 489.0, 517.0, 540.0, 595.0, 573.0, 629.0, 606.0, 652.0, 656.0, 663.0, 661.0, 659.0, 647.0, 580.0, 585.0, 535.0, 510.0, 531.0, 502.0, 481.0, 425.0, 405.0, 404.0, 341.0, 324.0, 280.0, 270.0, 236.0, 271.0, 229.0, 213.0, 194.0, 176.0, 182.0, 162.0, 180.0, 166.0, 149.0, 162.0, 144.0, 125.0, 135.0, 125.0, 144.0, 135.0, 141.0, 104.0, 113.0, 115.0, 117.0, 107.0, 119.0, 111.0, 115.0, 114.0, 93.0, 110.0, 117.0, 96.0, 112.0, 109.0, 101.0, 72.0, 75.0, 81.0, 97.0, 85.0, 88.0, 92.0, 64.0, 57.0, 62.0, 57.0, 61.0, 50.0, 66.0, 74.0, 65.0, 53.0, 57.0, 60.0, 56.0, 63.0, 55.0, 42.0, 58.0, 52.0, 53.0, 67.0, 51.0, 58.0, 53.0, 46.0, 48.0, 51.0, 43.0, 58.0, 56.0, 65.0, 51.0, 43.0, 51.0, 58.0, 47.0, 38.0, 60.0, 50.0, 52.0, 45.0, 48.0, 43.0, 58.0, 40.0, 46.0, 41.0, 56.0, 37.0, 43.0, 42.0, 50.0, 45.0, 44.0, 38.0, 34.0, 42.0, 51.0, 37.0, 49.0, 42.0, 38.0, 44.0, 32.0, 41.0, 44.0, 39.0, 26.0, 36.0, 40.0, 38.0, 47.0, 55.0, 45.0, 44.0, 37.0, 52.0, 54.0, 44.0, 47.0, 29.0, 39.0, 43.0, 40.0, 29.0, 34.0, 35.0, 42.0, 39.0, 38.0, 36.0, 37.0, 55.0, 42.0, 33.0, 35.0, 43.0, 42.0, 42.0, 39.0, 35.0, 36.0, 36.0, 29.0, 41.0, 36.0, 43.0, 35.0, 32.0, 31.0, 31.0, 37.0, 42.0, 42.0, 33.0, 36.0, 46.0, 42.0, 32.0, 44.0, 35.0, 43.0, 37.0, 48.0, 45.0, 37.0, 37.0, 33.0, 31.0, 35.0, 36.0, 33.0, 43.0, 38.0, 39.0, 26.0, 31.0, 35.0, 31.0, 47.0, 60.0, 34.0, 35.0, 35.0, 41.0, 37.0, 31.0, 25.0, 39.0, 31.0, 36.0, 34.0, 32.0, 29.0, 34.0, 37.0, 36.0, 34.0, 36.0, 45.0, 26.0, 40.0, 44.0, 36.0, 39.0, 36.0, 27.0, 40.0, 42.0, 40.0, 43.0, 26.0, 33.0, 40.0, 35.0, 37.0, 27.0, 26.0, 41.0, 36.0, 39.0, 35.0, 25.0, 34.0, 34.0, 42.0, 35.0, 34.0, 47.0, 34.0, 33.0, 31.0, 36.0, 39.0, 50.0, 44.0, 50.0, 40.0, 32.0, 37.0, 27.0, 41.0, 30.0, 31.0, 31.0, 33.0, 21.0, 36.0, 29.0, 33.0, 31.0, 41.0, 28.0, 28.0, 36.0, 26.0, 42.0, 30.0, 35.0, 34.0, 39.0, 33.0, 34.0, 40.0, 31.0, 29.0, 32.0, 35.0, 27.0, 33.0, 35.0, 42.0, 40.0, 43.0, 45.0, 31.0, 28.0, 32.0, 45.0, 47.0, 38.0, 26.0, 40.0, 28.0, 27.0, 36.0, 38.0, 35.0, 34.0, 38.0, 35.0, 46.0, 28.0, 38.0, 30.0, 36.0, 38.0, 42.0, 37.0, 37.0, 47.0, 35.0, 45.0, 21.0, 39.0, 33.0, 31.0, 33.0, 24.0, 41.0, 30.0, 44.0, 31.0, 38.0, 37.0, 39.0, 31.0, 39.0, 37.0, 41.0, 22.0, 39.0, 33.0, 31.0, 34.0, 35.0, 47.0, 41.0, 36.0, 35.0, 35.0, 33.0, 28.0, 41.0, 40.0, 33.0, 31.0, 34.0, 32.0, 24.0, 36.0, 32.0, 30.0, 37.0, 30.0, 36.0, 36.0, 31.0, 29.0, 31.0, 36.0, 26.0, 47.0, 34.0, 38.0, 37.0, 33.0, 25.0, 36.0, 32.0, 32.0, 38.0, 36.0, 36.0, 27.0, 27.0, 25.0, 33.0, 33.0, 35.0, 33.0, 32.0, 34.0, 38.0, 31.0, 29.0, 30.0, 30.0, 39.0, 39.0, 36.0, 28.0, 33.0, 26.0, 32.0, 27.0, 26.0, 44.0, 42.0, 38.0, 39.0, 37.0, 33.0, 32.0, 21.0, 26.0, 36.0, 35.0, 29.0, 26.0, 35.0, 34.0, 30.0, 34.0, 28.0, 34.0, 37.0, 50.0, 36.0, 37.0, 34.0, 31.0, 36.0, 40.0, 35.0, 29.0, 37.0, 49.0, 20.0, 43.0, 33.0, 31.0, 44.0, 41.0, 38.0, 32.0, 45.0, 42.0, 34.0, 37.0, 42.0, 35.0, 36.0, 22.0, 37.0, 44.0, 31.0, 37.0, 41.0, 31.0, 31.0, 31.0, 32.0, 39.0, 34.0, 31.0, 39.0, 32.0, 29.0, 34.0, 26.0, 23.0, 32.0, 31.0, 30.0, 35.0, 31.0, 33.0, 26.0, 31.0, 43.0, 34.0, 28.0, 40.0, 32.0, 33.0, 35.0, 39.0, 46.0, 48.0, 43.0, 31.0, 30.0, 26.0, 32.0, 43.0, 25.0, 39.0, 31.0, 28.0, 33.0, 25.0, 32.0, 28.0, 46.0, 31.0, 38.0, 35.0, 44.0, 38.0, 29.0, 30.0, 32.0, 42.0, 35.0, 33.0, 28.0, 37.0, 24.0, 30.0, 39.0, 36.0, 43.0]
  out "CH1 (WV off) smooth S":dbl[](array[numeric])=[33.81641460234679, 28.068696219035196, 25.82782268578879, 25.14757496740548, 25.46993481095176, 26.53088657105605, 28.2440547588005, 30.32032594524117, 33.03023468057362, 36.78153846153842, 41.19385919165576, 46.96602346805734, 53.96276401564537, 61.83303780964801, 71.23264667535858, 82.1055280312908, 94.18016949152549, 107.69222946544986, 122.68994784876143, 138.59053455019557, 155.7332985658409, 173.64659713168174, 191.72058670143403, 209.94222946544963, 227.8027249022162, 244.92202086049525, 260.7587222946544, 275.7398174706648, 288.699400260756, 299.72319426336355, 308.56804432855256, 314.2362320730114, 317.614654498044, 318.24698826597097, 316.0872750977833, 311.96993481095143, 304.90376792698794, 295.20526727509747, 283.7769752281614, 270.1299739243805, 256.38160365058656, 242.93766623207287, 230.16224250325928, 218.73916558018234, 208.31739243807027, 198.61041720990866, 188.4226727509778, 177.3724771838331, 165.042294654498, 152.37475880052148, 141.45526727509775, 132.12052151238595, 125.16354628422428, 119.59933507170801, 113.77273794002613, 108.44483702737946, 102.47026075619301, 96.70950456323342, 91.57325945241205, 86.55370273794009, 82.25350717079537, 78.2424250325946, 74.50709256844858, 71.27143415906134, 68.4151760104303, 65.6117209908736, 63.11400260756197, 60.85715775749678, 58.49698826597133, 56.36106910039115, 54.35389830508475, 52.0660886571056, 50.01393741851368, 47.89073011734026, 45.7297131681877, 43.69385919165576, 41.77501955671442, 39.97612777053449, 38.472216427640106, 36.9813428943937, 35.44874837027375, 34.28219035202082, 33.02925684485002, 32.01393741851365, 30.93408083441978, 29.90279009126463, 28.797183833116, 27.346727509778326, 25.96341590612775, 24.609113428943925, 23.350638852672752, 22.322607561929605, 21.441903520208623, 20.351290743155175, 19.431147327249057, 18.750899608865744, 18.106505867014373, 17.58108213820081, 16.970260756192985, 16.45331160365061, 16.056636245110845, 15.832385919165603, 15.729387222946569, 15.488187744458955, 15.112698826597157, 14.705267275097805, 14.122151238591936, 13.643989569752296, 13.1384485006519, 12.640404172099094, 12.264915254237295, 11.971564537157764, 11.770782268578884, 11.533820078226864, 11.344445893089965, 11.090534550195567, 10.90018252933507, 10.811199478487612, 10.56152542372881, 10.442229465449799, 10.22221642764015, 9.89105606258148, 9.731016949152535, 9.41550195567144, 9.207548891786171, 9.033820078226851, 8.857483702737934, 8.654419817470657, 8.412568448500647, 8.169739243807035, 8.029908735332459, 7.78642764015645, 7.632581486310297, 7.387796610169491, 6.981342894393742, 6.877692307692307, 6.724172099087353, 6.608461538461537, 6.615632333767925, 6.437992177314209, 6.251551499348107, 6.1681095176010405, 6.047835723598433, 5.936688396349412, 5.910286831812256, 5.722868318122556, 5.5227379400260785, 5.4793872229465475, 5.211460234680576, 5.176584093872232, 5.137796610169493, 4.954941329856586, 4.9624380704041755, 4.7945762711864415, 4.766219035202087, 4.816740547588006, 4.648878748370274, 4.544576271186442, 4.397574967405477, 4.268174706649283, 4.224172099087353, 4.173976531942634, 3.953637548891785, 3.778604954367665, 3.729713168187743, 3.6583311603650572, 3.718956975228161, 3.7042894393741843, 3.557288135593219, 3.548161668839634, 3.337926988265969, 3.2613298565840907, 3.29327249022164, 3.238187744458928, 3.231668839634939, 3.1534419817470636, 3.0686962190351985, 2.9451629726205955, 2.9601564537157716, 2.9670013037809606, 2.8216297262059933, 2.8089178617992134, 2.820977835723594, 2.602920469361144, 2.6850586701434125, 2.6560495436766596, 2.6821251629726177, 2.7577444589308966, 2.738513689700127, 2.6374706649282884, 2.5452281616688364, 2.5484876140808312, 2.491773142112122, 2.5413168187744426, 2.4331029986962163, 2.3509647979139476, 2.3359713168187715, 2.2502477183833083, 2.29881355932203, 2.275019556714469, 2.1355149934810926, 2.083363754889177, 2.0015514993481087, 2.087275097783571, 2.146271186440677, 2.234276401564536, 2.1987483702737927, 2.052073011734028, 2.0259973924380694, 1.93831812255541, 1.8164146023468053, 1.8278226857887874, 1.827822685788787, 1.7867535853976526, 1.8199999999999992, 1.8891003911342883, 1.733298565840938, 1.6681095176010423, 1.7456844850065174, 1.653767926988265, 1.5895567144719676, 1.5595697522816157, 1.4956844850065187, 1.3992046936114735, 1.4024641460234684, 1.3581355932203394, 1.1935332464146025, 1.2228683181225553, 1.290013037809648, 1.3529204693611474, 1.4656975228161668, 1.399530638852673, 1.2834941329856582, 1.180169491525423, 1.1456192959582785, 1.147900912646675, 1.1482268578878745, 1.1609387222946546, 1.0947718383311602, 1.0628292046936112, 1.1283441981747067, 1.1521382007822678, 1.1280182529335065, 1.074563233376792, 0.9350586701434153, 0.8861668839634935, 0.8920338983050841, 1.042620599739243, 1.0944458930899599, 1.0077444589308988, 0.9849282920469353, 0.8366232073011726, 0.8138070404172094, 0.8437940026075612, 0.8747588005215123, 0.8789960886571057, 0.9608083441981747, 0.9839504563233378, 1.0608735332464145, 1.0752151238591914, 1.140078226857888, 1.2033116036505869, 1.0915123859191656, 1.0696740547588002, 1.0162190352020855, 0.9894915254237281, 1.0129595827900906, 1.035775749674054, 0.8734550195567138, 0.7310169491525418, 0.6596349413298559, 0.5523989569752277, 0.5706518904823985, 0.7316688396349408, 0.7639374185136891, 0.8111994784876138, 0.8053324641460232, 0.7372099087353321, 0.6149804432855278, 0.6117209908735328, 0.7049413298565838, 0.6596349413298563, 0.7222164276401561, 0.6668057366362452, 0.5680443285528031, 0.5748891786179922, 0.62606258148631, 0.6143285528031286, 0.5928161668839632, 0.6113950456323337, 0.555658409387223, 0.5670664928292047, 0.5165449804432855, 0.4386440677966102, 0.44418513689700134, 0.45331160365058654, 0.5977053455019554, 0.5608735332464144, 0.5393611473272488, 0.4624380704041721, 0.32000000000000006, 0.2753455019556715, 0.35813559322033883, 0.41745762711864387, 0.431147327249022, 0.5325162972620598, 0.42853976531942656, 0.31674054758800535, 0.32586701434159077, 0.3649804432855279, 0.4220208604954364, 0.5155671447196869, 0.45526727509778336, 0.36823989569752286, 0.3379269882659716, 0.3063102998696222, 0.45657105606258164, 0.36530638852672753, 0.3516166883963494, 0.3053324641460234, 0.1567014341590613, 0.2482920469361148, 0.29457627118644075, 0.33303780964797924, 0.44059973924380713, 0.3851890482398958, 0.3190221642764016, 0.3480312907431552, 0.2508996088657106, 0.27208604954367666, 0.2231942633637548, 0.10943937418513681, 0.08694915254237276, 0.13975228161668848, 0.12573663624511083, 0.23688396349413293, 0.32423728813559327, 0.2570925684485005, 0.27371577574967393, 0.23916558018252937, 0.1593089960886571, 0.21374185136897006, 0.12769230769230777, 0.09835723598435467, 0.06804432855280318, 0.034471968709256826, 0.08792698826597127, 0.0879269882659713, 0.06804432855280311, -0.009530638852672819, 0.1557235984354626, 0.11889178617992152, 0.21960886571056049, 0.2668709256844849, 0.04099087353324648, 0.047509778357236014, -0.0359322033898306, -0.002359843546284185, 0.05956975228161669, 0.09411994784876146, 0.1544198174706649, 0.22645371577574966, 0.153116036505867, 0.03740547588005215, -0.005619295958278924, -0.0056192959582789526, 0.007418513689700167, 0.1902737940026077, 0.23329856584093886, 0.05337679269882671, 0.22254237288135592, 0.0752151238591916, 0.11335071707953043, 0.18245110821381982, 0.0814080834419816, 0.19353324641460215, 0.2773011734028682, 0.14105606258148629, 0.1615906127770534, 0.18799217731421114, 0.05370273794002615, 0.3294524119947848, 0.3450977835723599, 0.3395567144719688, 0.25546284224250326, 0.11758800521512394, 0.13844850065189057, 0.01915254237288146, 0.0918383311603651, 0.14170795306388526, 0.07977835723598428, 0.19581486310299862, 0.20331160365058668, 0.331734028683181, 0.31282920469361125, 0.28121251629726185, 0.16745762711864387, 0.01589308996088657, -0.022894393741851322, -0.053207301173402805, 0.031212516297262023, -0.04342894393741858, -0.0013820078226858962, -0.04245110821382014, -0.0659191655801826, -0.08123859191655802, -0.12491525423728816, -0.0030117340286832245, -0.010508474576271173, -0.06950456323337684, -0.04277705345501958, -0.20053455019556715, -0.2168318122555411, -0.07015645371577575, -0.011812255541069037, 0.05435462842242508, 0.1681095176010431, 0.1612646675358541, 0.18440677966101704, 0.23134289439374203, 0.23036505867014362, 0.23003911342894384, 0.1433376792698825, 0.08336375488917844, -0.03984354628422443, -0.029087353324641428, 0.009048239895697544, -0.0329986962190352, 0.10552803129074309, 0.08988265971316817, 0.07065189048239899, 0.1045501955671447, 0.007418513689700189, 0.027301173402868292, 0.11921773142112134, 0.23232073011734028, 0.2381877444589308, 0.14496740547587997, 0.07586701434159038, -0.09916558018252938, -0.07830508474576273, 0.0576140808344198, 0.05663624511082137, 0.18440677966101687, 0.1358409387222946, 0.09574967405475876, 0.09705345501955669, 0.12052151238591916, 0.09477183833116032, 0.031864406779661, 0.08368970013037809, -0.020938722294654485, 0.12443285528031288, 0.10422425032594518, 0.025345501955671368, 0.035123859191655726, -0.033650586701434254, 0.015567144719686982, -0.025827900912646817, -0.029739243807040613, -0.10340286831812265, -0.06298565840938729, 0.08336375488917872, 0.047509778357236125, 0.031212516297262155, -0.046036505867014216, -0.1311082138200782, -0.049947848761408065, 0.01361147327249021, 0.01393741851368965, -0.011486310299869651, -0.06754889178618, 0.01947848761408079, 0.09933507170795307, 0.11009126466753594, 0.1847327249022165, 0.16582790091264682, 0.140730117340287, 0.20983050847457638, 0.25741851368970026, 0.2029856584093873, 0.1368187744458931, 0.015241199478487642, -0.09916558018252934, -0.054837027379400265, -0.031043024771838346, 0.008070404172099036, -0.01670143415906131, 0.004810951760104168, 0.04881355932203374, 0.09509778357235975, 0.12019556714471963, 0.011003911342894385, -0.01930899608865709, -0.05907431551499347, -0.061681877444589285, -0.04473272490221639, -0.06591916558018247, -0.17445893089960876, -0.10731421121251626, -0.11644067796610168, -0.11481095176010435, 0.08531942633637528, 0.01165580182529314, 0.12899608865710535, 0.1759322033898303, 0.08336375488917849, 0.14887874837027368, 0.13910039113428935, 0.11693611473272482, 0.1322555410691003, 0.08238591916558004, 0.07619295958279002, 0.07554106910039103, 0.07554106910039102, 0.009700130378096486, -0.09329856584093871, -0.13958279009126462, -0.07504563233376782, 0.06771838331160371, 0.055006518904824046, -0.0036636245110820975, -0.07732724902216424, -0.14088657105606264, -0.07015645371577581, 0.010352020860495316, 0.10226857887874805, 0.09346805736636213, 0.030560625814862866, -0.12980443285528065, -0.27452411994784887, -0.22139504563233392, -0.15392438070404188, 0.00155149934810948, 0.06641460234680566, 0.11400260756192958, 0.1175880052151239, 0.18799217731421128, 0.2583963494132987, 0.10715775749674075, 0.0507692307692309, -0.0157235984354627, -0.026805736636245026, 0.06674054758800518, 0.04881355932203387, 0.1078096479791395, 0.029908735332464135, 0.008070404172099102, 0.07651890482398958, -0.002685788787483715, 0.04425032594524128, 0.01002607561929595, -0.05646675358539768, -0.13306388526727517, -0.2631160365058671]
  out "CH0 (WV on) smoothed":dbl[](array[numeric])=[37.478888888888896, 32.09, 30.284444444444453, 29.599259259259263, 29.552962962962965, 31.052962962962965, 31.72888888888889, 34.821481481481484, 37.92333333333333, 41.052962962962965, 46.302962962962965, 50.117777777777775, 56.534444444444446, 63.39555555555556, 72.05296296296297, 82.21037037037038, 93.59925925925927, 106.76592592592593, 119.06222222222223, 133.28444444444443, 146.14555555555557, 158.50666666666666, 172.46037037037036, 186.127037037037, 199.69185185185182, 214.3122222222222, 227.61777777777775, 240.27518518518517, 252.4788888888889, 262.84, 269.3122222222222, 274.9696296296296, 277.66407407407405, 278.3862962962963, 277.1085185185185, 272.9233333333333, 267.83074074074074, 262.02518518518514, 255.57148148148147, 246.12703703703698, 236.27518518518514, 224.4233333333333, 213.60851851851848, 202.53444444444443, 189.77518518518517, 175.5159259259259, 160.58074074074074, 143.0251851851852, 126.41407407407408, 109.92333333333333, 94.56222222222222, 85.07148148148147, 77.62703703703704, 72.6825925925926, 68.84, 64.87703703703704, 61.17333333333333, 58.20111111111112, 55.73814814814815, 51.87703703703704, 48.867777777777775, 46.94185185185185, 44.812222222222225, 44.22888888888889, 42.85851851851852, 40.44185185185186, 38.043703703703706, 36.67333333333334, 34.99740740740741, 33.46037037037037, 32.50666666666667, 30.525185185185187, 28.580740740740744, 27.59925925925926, 26.756666666666668, 26.21037037037037, 25.747407407407405, 25.293703703703702, 24.728888888888886, 24.654814814814813, 24.284444444444443, 23.765925925925927, 23.18259259259259, 22.904814814814817, 22.515925925925924, 21.60851851851852, 20.312222222222225, 17.914074074074072, 16.275185185185183, 14.645555555555557, 13.710370370370372, 12.691851851851855, 11.84, 11.414074074074076, 10.849259259259261, 10.756666666666668, 10.756666666666668, 10.664074074074076, 10.071481481481483, 9.83074074074074, 9.858518518518519, 9.108518518518519, 8.960370370370372, 8.654814814814815, 7.552962962962963, 7.4325925925925915, 6.728888888888887, 6.562222222222221, 7.284444444444443, 7.377037037037036, 7.941851851851851, 8.33074074074074, 7.645555555555555, 7.284444444444443, 7.460370370370369, 6.775185185185185, 6.395555555555555, 5.756666666666666, 5.164074074074073, 5.1825925925925915, 5.08074074074074, 5.636296296296296, 5.062222222222221, 4.543703703703703, 4.571481481481481, 4.654814814814814, 5.293703703703703, 5.1825925925925915, 5.219629629629629, 4.802962962962962, 4.339999999999999, 4.552962962962962, 4.423333333333332, 4.608518518518517, 4.5992592592592585, 4.432592592592592, 4.127037037037036, 3.543703703703703, 3.062222222222222, 2.4048148148148147, 2.4233333333333333, 1.7751851851851852, 1.8122222222222224, 2.4788888888888887, 2.506666666666666, 2.784444444444444, 3.191851851851851, 2.7659259259259255, 3.2011111111111106, 3.0807407407407403, 2.6270370370370366, 3.4325925925925924, 3.0066666666666664, 3.7381481481481478, 3.441851851851851, 2.645555555555555, 2.377037037037037, 1.9603703703703705, 2.451111111111111, 1.9881481481481484, 1.941851851851852, 1.802962962962963, 1.3307407407407408, 1.7196296296296296, 1.765925925925926, 2.0807407407407403, 2.164074074074074, 2.3862962962962957, 2.2288888888888887, 2.1362962962962957, 2.395555555555555, 2.0529629629629627, 1.5992592592592587, 1.7288888888888887, 1.7381481481481478, 1.9788888888888887, 2.284444444444444, 2.349259259259259, 1.488148148148148, 1.21037037037037, 1.886296296296296, 1.5807407407407406, 2.312222222222222, 2.4696296296296296, 2.506666666666667, 2.1825925925925924, 2.284444444444444, 2.265925925925926, 1.3955555555555557, 1.7196296296296296, 1.5807407407407408, 1.654814814814815, 1.8955555555555557, 1.5992592592592594, 1.5899999999999999, 1.3585185185185185, 0.9233333333333331, 1.1548148148148147, 1.2844444444444445, 1.1918518518518517, 1.2196296296296296, 0.9048148148148147, 0.5344444444444444, 0.9511111111111108, 1.3492592592592592, 1.4048148148148145, 1.7196296296296294, 0.9603703703703703, 0.8029629629629631, 1.3862962962962961, 1.1455555555555554, 1.9048148148148147, 2.0344444444444445, 1.6455555555555557, 1.4974074074074077, 0.9511111111111111, 0.7288888888888889, 0.39555555555555555, 0.9696296296296295, 1.265925925925926, 1.525185185185185, 1.9881481481481482, 0.9788888888888889, 0.8400000000000001, 1.0066666666666666, 0.37703703703703695, 1.0529629629629629, 1.3399999999999999, 1.2474074074074073, 1.7844444444444445, 1.451111111111111, 0.9325925925925926, 1.127037037037037, 1.4048148148148147, 1.4140740740740738, 1.4788888888888887, 1.0437037037037036, 0.4140740740740741, 0.5437037037037037, 1.0807407407407406, 0.9974074074074072, 1.1362962962962961, 0.9974074074074072, -0.14148148148148149, 0.07148148148148148, -0.21555555555555556, -0.2062962962962963, 0.5437037037037037, 0.2011111111111111, 0.3214814814814815, 0.14555555555555555, 0.2381481481481481, 0.5251851851851852, 0.21962962962962962, 0.7381481481481481, 0.4696296296296297, 0.6177777777777778, 1.0714814814814815, 1.1362962962962964, 1.265925925925926, 0.7474074074074074, 0.5807407407407408, 0.09925925925925924, 0.25666666666666665, 0.6825925925925926, 0.6548148148148147, 1.6548148148148145, 1.8585185185185185, 2.2011111111111106, 2.3122222222222217, 1.775185185185185, 1.2844444444444443, 0.41407407407407404, 0.30296296296296293, -0.002592592592592591, 0.34925925925925927, 0.4974074074074074, 0.5807407407407408, 0.9881481481481481, 0.7937037037037037, 1.5251851851851852, 1.7751851851851854, 1.367777777777778, 1.0437037037037038, -0.1044444444444445, -0.058148148148148115, 0.2566666666666667, 0.12703703703703703, 0.7844444444444444, 0.7844444444444445, 0.8677777777777778, 1.4325925925925924, 1.8585185185185185, 0.9788888888888887, 0.09925925925925927, 0.5714814814814813, -0.3544444444444447, 0.1733333333333331, 0.4603703703703701, -0.6044444444444445, -0.7988888888888889, -0.5581481481481481, 0.03444444444444433, 0.38629629629629625, 1.201111111111111, 0.7196296296296295, 0.7381481481481482, 0.6455555555555557, 0.08074074074074078, 0.6825925925925926, 0.17333333333333334, 0.45111111111111113, 1.052962962962963, 1.3770370370370368, 1.6825925925925924, 1.8585185185185182, 2.284444444444444, 2.127037037037037, 2.1733333333333333, 1.5899999999999999, 1.164074074074074, 0.6733333333333333, 0.14555555555555555, 0.5159259259259259, 0.5807407407407408, 1.1455555555555557, 1.2659259259259261, 1.1362962962962966, 0.9233333333333335, -0.03962962962962957, -0.2248148148148148, 0.31222222222222196, 0.562222222222222, 0.8029629629629627, 0.9974074074074072, 0.6918518518518519, 0.5344444444444445, 0.8307407407407408, 1.275185185185185, 1.164074074074074, 1.3585185185185185, 1.3955555555555554, 0.6548148148148147, 0.6177777777777778, -0.3451851851851852, -0.07666666666666666, 0.6918518518518518, 0.6270370370370371, 1.627037037037037, 1.2011111111111112, 1.0251851851851852, 1.1733333333333333, 0.7474074074074074, 1.0251851851851852, 1.0714814814814815, 1.2566666666666666, 0.9048148148148147, 0.2844444444444444, 0.03444444444444446, -0.6229629629629629, -0.02111111111111108, 0.12703703703703706, 0.6455555555555554, 1.0437037037037036, 0.3307407407407406, 0.13629629629629614, -0.13222222222222224, -0.011851851851851891, 0.8492592592592593, 0.8029629629629629, -0.021111111111111025, -0.29888888888888887, -0.7803703703703705, -0.08592592592592602, 0.052962962962962934, 0.377037037037037, 0.59, 0.24740740740740744, -0.002592592592592591, -0.34518518518518515, -0.6322222222222222, -0.9840740740740741, -0.6137037037037038, -0.7711111111111112, -0.39148148148148154, 0.21037037037037037, 0.7288888888888889, 0.9603703703703704, 1.09, 0.7937037037037037, 0.664074074074074, 0.6177777777777779, -0.002592592592592591, -0.07666666666666669, -0.38222222222222224, 0.12703703703703695, 0.5344444444444444, 0.7844444444444443, 0.877037037037037, 0.6270370370370371, 0.4048148148148148, 0.5066666666666666, 0.302962962962963, -0.09518518518518516, -0.447037037037037, -0.28962962962962957, 0.07148148148148152, 0.01592592592592597, 0.40481481481481474, 0.38629629629629625, 0.4233333333333334, 0.5622222222222222, 0.6177777777777778, 0.20111111111111116, 0.006666666666666668, 0.03444444444444444, -0.14148148148148149, 0.4788888888888887, 0.5529629629629628, 0.6918518518518517, 1.1362962962962961, 0.7288888888888889, 0.6362962962962962, 0.5251851851851851, 0.09925925925925924, -0.02111111111111113, 0.5992592592592593, 0.7196296296296296, 0.9974074074074075, 0.8770370370370371, 0.42333333333333334, 0.6270370370370371, 0.4325925925925926, 0.44185185185185183, 0.6548148148148147, 0.33999999999999997, 0.6825925925925925, 0.4603703703703703, 0.3214814814814815, 1.1177777777777775, 1.0344444444444443, 1.6918518518518517, 1.6455555555555554, 1.3307407407407408, 0.849259259259259, 0.5622222222222222, 0.627037037037037, 0.14555555555555555, 0.18259259259259256, 0.39555555555555555, 0.34925925925925927, 0.17333333333333328, 0.6362962962962964, -0.1137037037037037, 0.31222222222222223, 1.025185185185185, 0.7659259259259257, 1.2474074074074073, 0.22888888888888864, -0.1414814814814815, -0.002592592592592591, 0.6362962962962961, 0.8214814814814814, 0.14555555555555533, 0.09925925925925905, -0.5118518518518519, 0.09925925925925924, 0.6733333333333333, 0.8122222222222222, 0.7659259259259259, 0.7937037037037037, 0.7474074074074074, 0.8677777777777778, 1.2381481481481482, 0.9603703703703704, 0.6085185185185186, 0.15481481481481482, -0.798888888888889, -0.4192592592592593, -0.021111111111111136, 0.44185185185185183, 1.2937037037037038, 0.6918518518518519, 0.8585185185185185, 0.42333333333333323, 0.21962962962962954, 0.5437037037037036, 0.42333333333333334, 0.7288888888888889, 0.43259259259259253, -0.0396296296296296, -0.4192592592592592, -0.4562962962962963, -0.12296296296296294, -0.24333333333333332, 0.3862962962962963, 0.06222222222222222, 0.37703703703703706, 0.7844444444444445, 0.7288888888888889, 1.4881481481481482, 1.1825925925925926, 1.4603703703703705, 1.441851851851852, 0.9325925925925926, 0.8307407407407408, 0.7844444444444445, 0.34925925925925927, 0.3862962962962963, 0.47888888888888886, 0.5622222222222222, 0.6918518518518518, 1.127037037037037, 1.7288888888888887, 1.6825925925925926, 2.525185185185185, 1.4974074074074073, 0.2288888888888887, -0.36370370370370386, -1.0303703703703702, -0.03962962962962968, 0.42333333333333323, 1.275185185185185, 1.3399999999999999, 0.6640740740740738, 1.4974074074074069, 0.6085185185185182, -0.011851851851852002, 0.5344444444444443, -0.17851851851851855, -0.09518518518518523, -0.10444444444444445, -0.8914814814814815, -0.6322222222222222, -0.38222222222222224, -0.08592592592592595, 0.3585185185185185, 0.08074074074074074, -0.14148148148148149, -0.11370370370370371, 0.052962962962962906, 0.06222222222222218, 0.7937037037037037, 0.701111111111111, 0.24740740740740744, 0.06222222222222221, -0.8081481481481483, -0.6137037037037038, -0.33592592592592596, 0.052962962962962906, 0.6177777777777778, 0.21962962962962956, -0.2155555555555556, -0.11370370370370375, 0.127037037037037]
  out "CH 0 Bin Readings":dbl[](array[numeric])=[73.0, 73.0, 64.0, 68.0, 69.0, 54.0, 62.0, 61.0, 59.0, 70.0, 63.0, 73.0, 76.0, 79.0, 100.0, 93.0, 104.0, 130.0, 150.0, 152.0, 142.0, 182.0, 183.0, 223.0, 237.0, 220.0, 245.0, 264.0, 299.0, 280.0, 281.0, 285.0, 303.0, 310.0, 318.0, 305.0, 318.0, 311.0, 299.0, 320.0, 290.0, 280.0, 278.0, 249.0, 243.0, 221.0, 211.0, 193.0, 168.0, 153.0, 164.0, 147.0, 130.0, 146.0, 133.0, 120.0, 115.0, 100.0, 97.0, 84.0, 76.0, 80.0, 86.0, 71.0, 85.0, 87.0, 87.0, 69.0, 72.0, 69.0, 76.0, 55.0, 69.0, 74.0, 77.0, 80.0, 50.0, 50.0, 58.0, 51.0, 58.0, 52.0, 53.0, 51.0, 50.0, 64.0, 59.0, 48.0, 53.0, 70.0, 64.0, 47.0, 56.0, 54.0, 47.0, 47.0, 51.0, 50.0, 46.0, 32.0, 37.0, 41.0, 22.0, 39.0, 44.0, 34.0, 50.0, 34.0, 33.0, 52.0, 36.0, 35.0, 48.0, 41.0, 34.0, 47.0, 31.0, 33.0, 21.0, 40.0, 34.0, 40.0, 43.0, 32.0, 38.0, 42.0, 26.0, 34.0, 39.0, 47.0, 38.0, 29.0, 35.0, 37.0, 38.0, 26.0, 36.0, 30.0, 37.0, 31.0, 35.0, 36.0, 38.0, 40.0, 43.0, 36.0, 26.0, 33.0, 36.0, 38.0, 31.0, 27.0, 39.0, 31.0, 33.0, 30.0, 37.0, 41.0, 34.0, 41.0, 37.0, 34.0, 27.0, 21.0, 22.0, 23.0, 32.0, 32.0, 44.0, 39.0, 28.0, 26.0, 20.0, 40.0, 33.0, 30.0, 26.0, 32.0, 44.0, 34.0, 57.0, 33.0, 32.0, 41.0, 27.0, 39.0, 33.0, 26.0, 31.0, 25.0, 25.0, 31.0, 35.0, 33.0, 44.0, 21.0, 30.0, 41.0, 29.0, 30.0, 46.0, 28.0, 34.0, 30.0, 32.0, 47.0, 33.0, 28.0, 22.0, 29.0, 34.0, 28.0, 34.0, 41.0, 29.0, 44.0, 25.0, 43.0, 22.0, 17.0, 38.0, 32.0, 40.0, 33.0, 33.0, 25.0, 21.0, 30.0, 28.0, 27.0, 33.0, 33.0, 31.0, 29.0, 44.0, 29.0, 37.0, 30.0, 36.0, 31.0, 18.0, 33.0, 30.0, 28.0, 31.0, 37.0, 29.0, 27.0, 35.0, 28.0, 29.0, 29.0, 25.0, 32.0, 30.0, 36.0, 28.0, 38.0, 26.0, 27.0, 36.0, 48.0, 35.0, 27.0, 31.0, 35.0, 34.0, 32.0, 32.0, 38.0, 36.0, 32.0, 30.0, 24.0, 30.0, 35.0, 35.0, 33.0, 38.0, 18.0, 30.0, 34.0, 47.0, 29.0, 26.0, 35.0, 36.0, 49.0, 33.0, 24.0, 34.0, 34.0, 40.0, 32.0, 31.0, 34.0, 31.0, 16.0, 33.0, 23.0, 34.0, 32.0, 36.0, 42.0, 28.0, 31.0, 29.0, 28.0, 33.0, 33.0, 36.0, 31.0, 29.0, 27.0, 33.0, 30.0, 34.0, 31.0, 33.0, 43.0, 27.0, 24.0, 46.0, 34.0, 30.0, 29.0, 32.0, 28.0, 38.0, 40.0, 33.0, 31.0, 33.0, 31.0, 27.0, 33.0, 22.0, 22.0, 39.0, 42.0, 27.0, 33.0, 38.0, 36.0, 35.0, 35.0, 27.0, 30.0, 44.0, 28.0, 35.0, 27.0, 32.0, 29.0, 31.0, 42.0, 29.0, 37.0, 39.0, 32.0, 37.0, 32.0, 34.0, 28.0, 38.0, 28.0, 29.0, 28.0, 43.0, 25.0, 38.0, 18.0, 29.0, 36.0, 25.0, 42.0, 36.0, 31.0, 32.0, 29.0, 44.0, 30.0, 46.0, 24.0, 37.0, 31.0, 29.0, 37.0, 24.0, 37.0, 21.0, 29.0, 29.0, 29.0, 25.0, 42.0, 48.0, 30.0, 27.0, 32.0, 44.0, 27.0, 32.0, 33.0, 30.0, 23.0, 30.0, 29.0, 35.0, 26.0, 22.0, 30.0, 33.0, 35.0, 32.0, 34.0, 34.0, 33.0, 34.0, 27.0, 33.0, 36.0, 33.0, 30.0, 29.0, 30.0, 24.0, 40.0, 28.0, 35.0, 23.0, 40.0, 27.0, 28.0, 19.0, 32.0, 25.0, 45.0, 29.0, 34.0, 32.0, 32.0, 43.0, 38.0, 29.0, 33.0, 36.0, 33.0, 27.0, 34.0, 36.0, 32.0, 31.0, 35.0, 19.0, 30.0, 35.0, 37.0, 22.0, 32.0, 24.0, 34.0, 11.0, 38.0, 44.0, 36.0, 32.0, 32.0, 32.0, 24.0, 27.0, 34.0, 36.0, 30.0, 34.0, 30.0, 37.0, 19.0, 39.0, 32.0, 35.0, 34.0, 33.0, 29.0, 28.0, 35.0, 29.0, 33.0, 33.0, 28.0, 47.0, 33.0, 38.0, 30.0, 36.0, 38.0, 41.0, 23.0, 37.0, 23.0, 37.0, 26.0, 23.0, 33.0, 46.0, 37.0, 36.0, 35.0, 28.0, 29.0, 38.0, 38.0, 36.0, 37.0, 29.0, 35.0, 32.0, 33.0, 28.0, 37.0, 35.0, 27.0, 25.0, 21.0, 31.0, 34.0, 31.0, 31.0, 30.0, 25.0, 31.0, 35.0, 26.0, 28.0, 27.0, 30.0, 21.0, 29.0, 31.0, 31.0, 39.0, 31.0, 33.0, 38.0, 27.0, 37.0, 39.0, 30.0, 27.0, 24.0, 27.0, 23.0, 26.0, 31.0, 30.0, 31.0, 29.0, 31.0, 32.0]
  out "Range Corrected Altitude Array":dbl[](array[numeric])=[1406.25, 5625.0, 12656.25, 22500.0, 35156.25, 50625.0, 68906.25, 90000.0, 113906.25, 140625.0, 170156.25, 202500.0, 237656.25, 275625.0, 316406.25, 360000.0, 406406.25, 455625.0, 507656.25, 562500.0, 620156.25, 680625.0, 743906.25, 810000.0, 878906.25, 950625.0, 1025156.25, 1102500.0, 1182656.25, 1265625.0, 1351406.25, 1440000.0, 1531406.25, 1625625.0, 1722656.25, 1822500.0, 1925156.25, 2030625.0, 2138906.25, 2250000.0, 2363906.25, 2480625.0, 2600156.25, 2722500.0, 2847656.25, 2975625.0, 3106406.25, 3240000.0, 3376406.25, 3515625.0, 3657656.25, 3802500.0, 3950156.25, 4100625.0, 4253906.25, 4410000.0, 4568906.25, 4730625.0, 4895156.25, 5062500.0, 5232656.25, 5405625.0, 5581406.25, 5760000.0, 5941406.25, 6125625.0, 6312656.25, 6502500.0, 6695156.25, 6890625.0, 7088906.25, 7290000.0, 7493906.25, 7700625.0, 7910156.25, 8122500.0, 8337656.25, 8555625.0, 8776406.25, 9000000.0, 9226406.25, 9455625.0, 9687656.25, 9922500.0, 10160156.25, 10400625.0, 10643906.25, 10890000.0, 11138906.25, 11390625.0, 11645156.25, 11902500.0, 12162656.25, 12425625.0, 12691406.25, 12960000.0, 13231406.25, 13505625.0, 13782656.25, 14062500.0, 14345156.25, 14630625.0, 14918906.25, 15210000.0, 15503906.25, 15800625.0, 16100156.25, 16402500.0, 16707656.25, 17015625.0, 17326406.25, 17640000.0, 17956406.25, 18275625.0, 18597656.25, 18922500.0, 19250156.25, 19580625.0, 19913906.25, 20250000.0, 20588906.25, 20930625.0, 21275156.25, 21622500.0, 21972656.25, 22325625.0, 22681406.25, 23040000.0, 23401406.25, 23765625.0, 24132656.25, 24502500.0, 24875156.25, 25250625.0, 25628906.25, 26010000.0, 26393906.25, 26780625.0, 27170156.25, 27562500.0, 27957656.25, 28355625.0, 28756406.25, 29160000.0, 29566406.25, 29975625.0, 30387656.25, 30802500.0, 31220156.25, 31640625.0, 32063906.25, 32490000.0, 32918906.25, 33350625.0, 33785156.25, 34222500.0, 34662656.25, 35105625.0, 35551406.25, 36000000.0, 36451406.25, 36905625.0, 37362656.25, 37822500.0, 38285156.25, 38750625.0, 39218906.25, 39690000.0, 40163906.25, 40640625.0, 41120156.25, 41602500.0, 42087656.25, 42575625.0, 43066406.25, 43560000.0, 44056406.25, 44555625.0, 45057656.25, 45562500.0, 46070156.25, 46580625.0, 47093906.25, 47610000.0, 48128906.25, 48650625.0, 49175156.25, 49702500.0, 50232656.25, 50765625.0, 51301406.25, 51840000.0, 52381406.25, 52925625.0, 53472656.25, 54022500.0, 54575156.25, 55130625.0, 55688906.25, 56250000.0, 56813906.25, 57380625.0, 57950156.25, 58522500.0, 59097656.25, 59675625.0, 60256406.25, 60840000.0, 61426406.25, 62015625.0, 62607656.25, 63202500.0, 63800156.25, 64400625.0, 65003906.25, 65610000.0, 66218906.25, 66830625.0, 67445156.25, 68062500.0, 68682656.25, 69305625.0, 69931406.25, 70560000.0, 71191406.25, 71825625.0, 72462656.25, 73102500.0, 73745156.25, 74390625.0, 75038906.25, 75690000.0, 76343906.25, 77000625.0, 77660156.25, 78322500.0, 78987656.25, 79655625.0, 80326406.25, 81000000.0, 81676406.25, 82355625.0, 83037656.25, 83722500.0, 84410156.25, 85100625.0, 85793906.25, 86490000.0, 87188906.25, 87890625.0, 88595156.25, 89302500.0, 90012656.25, 90725625.0, 91441406.25, 92160000.0, 92881406.25, 93605625.0, 94332656.25, 95062500.0, 95795156.25, 96530625.0, 97268906.25, 98010000.0, 98753906.25, 99500625.0, 100250156.25, 101002500.0, 101757656.25, 102515625.0, 103276406.25, 104040000.0, 104806406.25, 105575625.0, 106347656.25, 107122500.0, 107900156.25, 108680625.0, 109463906.25, 110250000.0, 111038906.25, 111830625.0, 112625156.25, 113422500.0, 114222656.25, 115025625.0, 115831406.25, 116640000.0, 117451406.25, 118265625.0, 119082656.25, 119902500.0, 120725156.25, 121550625.0, 122378906.25, 123210000.0, 124043906.25, 124880625.0, 125720156.25, 126562500.0, 127407656.25, 128255625.0, 129106406.25, 129960000.0, 130816406.25, 131675625.0, 132537656.25, 133402500.0, 134270156.25, 135140625.0, 136013906.25, 136890000.0, 137768906.25, 138650625.0, 139535156.25, 140422500.0, 141312656.25, 142205625.0, 143101406.25, 144000000.0, 144901406.25, 145805625.0, 146712656.25, 147622500.0, 148535156.25, 149450625.0, 150368906.25, 151290000.0, 152213906.25, 153140625.0, 154070156.25, 155002500.0, 155937656.25, 156875625.0, 157816406.25, 158760000.0, 159706406.25, 160655625.0, 161607656.25, 162562500.0, 163520156.25, 164480625.0, 165443906.25, 166410000.0, 167378906.25, 168350625.0, 169325156.25, 170302500.0, 171282656.25, 172265625.0, 173251406.25, 174240000.0, 175231406.25, 176225625.0, 177222656.25, 178222500.0, 179225156.25, 180230625.0, 181238906.25, 182250000.0, 183263906.25, 184280625.0, 185300156.25, 186322500.0, 187347656.25, 188375625.0, 189406406.25, 190440000.0, 191476406.25, 192515625.0, 193557656.25, 194602500.0, 195650156.25, 196700625.0, 197753906.25, 198810000.0, 199868906.25, 200930625.0, 201995156.25, 203062500.0, 204132656.25, 205205625.0, 206281406.25, 207360000.0, 208441406.25, 209525625.0, 210612656.25, 211702500.0, 212795156.25, 213890625.0, 214988906.25, 216090000.0, 217193906.25, 218300625.0, 219410156.25, 220522500.0, 221637656.25, 222755625.0, 223876406.25, 225000000.0, 226126406.25, 227255625.0, 228387656.25, 229522500.0, 230660156.25, 231800625.0, 232943906.25, 234090000.0, 235238906.25, 236390625.0, 237545156.25, 238702500.0, 239862656.25, 241025625.0, 242191406.25, 243360000.0, 244531406.25, 245705625.0, 246882656.25, 248062500.0, 249245156.25, 250430625.0, 251618906.25, 252810000.0, 254003906.25, 255200625.0, 256400156.25, 257602500.0, 258807656.25, 260015625.0, 261226406.25, 262440000.0, 263656406.25, 264875625.0, 266097656.25, 267322500.0, 268550156.25, 269780625.0, 271013906.25, 272250000.0, 273488906.25, 274730625.0, 275975156.25, 277222500.0, 278472656.25, 279725625.0, 280981406.25, 282240000.0, 283501406.25, 284765625.0, 286032656.25, 287302500.0, 288575156.25, 289850625.0, 291128906.25, 292410000.0, 293693906.25, 294980625.0, 296270156.25, 297562500.0, 298857656.25, 300155625.0, 301456406.25, 302760000.0, 304066406.25, 305375625.0, 306687656.25, 308002500.0, 309320156.25, 310640625.0, 311963906.25, 313290000.0, 314618906.25, 315950625.0, 317285156.25, 318622500.0, 319962656.25, 321305625.0, 322651406.25, 324000000.0, 325351406.25, 326705625.0, 328062656.25, 329422500.0, 330785156.25, 332150625.0, 333518906.25, 334890000.0, 336263906.25, 337640625.0, 339020156.25, 340402500.0, 341787656.25, 343175625.0, 344566406.25, 345960000.0, 347356406.25, 348755625.0, 350157656.25, 351562500.0, 352970156.25, 354380625.0, 355793906.25, 357210000.0, 358628906.25, 360050625.0, 361475156.25, 362902500.0, 364332656.25, 365765625.0, 367201406.25, 368640000.0, 370081406.25, 371525625.0, 372972656.25, 374422500.0, 375875156.25, 377330625.0, 378788906.25, 380250000.0, 381713906.25, 383180625.0, 384650156.25, 386122500.0, 387597656.25, 389075625.0, 390556406.25, 392040000.0, 393526406.25, 395015625.0, 396507656.25, 398002500.0, 399500156.25, 401000625.0, 402503906.25, 404010000.0, 405518906.25, 407030625.0, 408545156.25, 410062500.0, 411582656.25, 413105625.0, 414631406.25, 416160000.0, 417691406.25, 419225625.0, 420762656.25, 422302500.0, 423845156.25, 425390625.0, 426938906.25, 428490000.0, 430043906.25, 431600625.0, 433160156.25, 434722500.0, 436287656.25, 437855625.0, 439426406.25, 441000000.0]
  out "Altitude Array (km)":dbl[](array[numeric])=[0.0375, 0.075, 0.11249999999999999, 0.15, 0.1875, 0.225, 0.26249999999999996, 0.3, 0.33749999999999997, 0.37499999999999994, 0.4125, 0.44999999999999996, 0.48749999999999993, 0.525, 0.5625, 0.6, 0.6375, 0.6749999999999999, 0.7124999999999999, 0.75, 0.7875, 0.825, 0.8624999999999999, 0.8999999999999999, 0.9374999999999999, 0.975, 1.0125, 1.05, 1.0875000000000001, 1.125, 1.1625, 1.2, 1.2375, 1.2750000000000001, 1.3125, 1.35, 1.3875, 1.425, 1.4625000000000001, 1.5, 1.5375, 1.575, 1.6125, 1.6500000000000001, 1.6875, 1.725, 1.7625, 1.8, 1.8375, 1.875, 1.9125, 1.95, 1.9875, 2.025, 2.0625, 2.1, 2.1375, 2.175, 2.2125, 2.25, 2.2875, 2.325, 2.3625, 2.4, 2.4375, 2.475, 2.5125, 2.55, 2.5875, 2.625, 2.6625, 2.7, 2.7375, 2.775, 2.8125, 2.85, 2.8875, 2.925, 2.9625, 3.0, 3.0375, 3.075, 3.1125, 3.15, 3.1875, 3.225, 3.2625, 3.3, 3.3375, 3.375, 3.4125, 3.45, 3.4875, 3.525, 3.5625, 3.6, 3.6374999999999997, 3.675, 3.7125, 3.75, 3.7875, 3.8249999999999997, 3.8625, 3.9, 3.9375, 3.975, 4.012499999999999, 4.05, 4.0874999999999995, 4.124999999999999, 4.1625, 4.199999999999999, 4.2375, 4.2749999999999995, 4.312499999999999, 4.35, 4.387499999999999, 4.425, 4.4624999999999995, 4.499999999999999, 4.5375, 4.574999999999999, 4.6125, 4.6499999999999995, 4.687499999999999, 4.725, 4.762499999999999, 4.8, 4.8374999999999995, 4.874999999999999, 4.9125, 4.949999999999999, 4.9875, 5.0249999999999995, 5.062499999999999, 5.1, 5.137499999999999, 5.175, 5.2124999999999995, 5.249999999999999, 5.2875, 5.324999999999999, 5.3625, 5.3999999999999995, 5.437499999999999, 5.475, 5.512499999999999, 5.55, 5.5874999999999995, 5.624999999999999, 5.6625, 5.699999999999999, 5.7375, 5.7749999999999995, 5.812499999999999, 5.85, 5.887499999999999, 5.925, 5.9624999999999995, 5.999999999999999, 6.0375, 6.074999999999999, 6.1125, 6.1499999999999995, 6.187499999999999, 6.225, 6.262499999999999, 6.3, 6.3374999999999995, 6.374999999999999, 6.4125, 6.449999999999999, 6.4875, 6.5249999999999995, 6.562499999999999, 6.6, 6.637499999999999, 6.675, 6.7124999999999995, 6.749999999999999, 6.7875, 6.824999999999999, 6.8625, 6.8999999999999995, 6.937499999999999, 6.975, 7.012499999999999, 7.05, 7.0874999999999995, 7.124999999999999, 7.1625, 7.199999999999999, 7.237499999999999, 7.2749999999999995, 7.312499999999999, 7.35, 7.387499999999999, 7.424999999999999, 7.4624999999999995, 7.499999999999999, 7.5375, 7.574999999999999, 7.612499999999999, 7.6499999999999995, 7.687499999999999, 7.725, 7.762499999999999, 7.799999999999999, 7.8374999999999995, 7.874999999999999, 7.9125, 7.949999999999999, 7.987499999999999, 8.025, 8.0625, 8.1, 8.1375, 8.174999999999999, 8.212499999999999, 8.25, 8.2875, 8.325, 8.362499999999999, 8.399999999999999, 8.4375, 8.475, 8.5125, 8.549999999999999, 8.587499999999999, 8.625, 8.6625, 8.7, 8.737499999999999, 8.774999999999999, 8.8125, 8.85, 8.8875, 8.924999999999999, 8.962499999999999, 9.0, 9.0375, 9.075, 9.112499999999999, 9.149999999999999, 9.1875, 9.225, 9.2625, 9.299999999999999, 9.337499999999999, 9.375, 9.4125, 9.45, 9.487499999999999, 9.524999999999999, 9.5625, 9.6, 9.6375, 9.674999999999999, 9.712499999999999, 9.75, 9.7875, 9.825, 9.862499999999999, 9.899999999999999, 9.9375, 9.975, 10.0125, 10.049999999999999, 10.087499999999999, 10.125, 10.1625, 10.2, 10.237499999999999, 10.274999999999999, 10.3125, 10.35, 10.3875, 10.424999999999999, 10.462499999999999, 10.5, 10.5375, 10.575, 10.612499999999999, 10.649999999999999, 10.6875, 10.725, 10.7625, 10.799999999999999, 10.837499999999999, 10.875, 10.9125, 10.95, 10.987499999999999, 11.024999999999999, 11.0625, 11.1, 11.1375, 11.174999999999999, 11.212499999999999, 11.25, 11.2875, 11.325, 11.362499999999999, 11.399999999999999, 11.4375, 11.475, 11.5125, 11.549999999999999, 11.587499999999999, 11.625, 11.6625, 11.7, 11.737499999999999, 11.774999999999999, 11.8125, 11.85, 11.8875, 11.924999999999999, 11.962499999999999, 12.0, 12.0375, 12.075, 12.112499999999999, 12.149999999999999, 12.1875, 12.225, 12.2625, 12.299999999999999, 12.337499999999999, 12.375, 12.4125, 12.45, 12.487499999999999, 12.524999999999999, 12.5625, 12.6, 12.6375, 12.674999999999999, 12.712499999999999, 12.75, 12.7875, 12.825, 12.862499999999999, 12.899999999999999, 12.9375, 12.975, 13.0125, 13.049999999999999, 13.087499999999999, 13.125, 13.1625, 13.2, 13.237499999999999, 13.274999999999999, 13.3125, 13.35, 13.3875, 13.424999999999999, 13.462499999999999, 13.5, 13.5375, 13.575, 13.612499999999999, 13.649999999999999, 13.6875, 13.725, 13.7625, 13.799999999999999, 13.837499999999999, 13.875, 13.9125, 13.95, 13.987499999999999, 14.024999999999999, 14.0625, 14.1, 14.1375, 14.174999999999999, 14.212499999999999, 14.25, 14.2875, 14.325, 14.362499999999999, 14.399999999999999, 14.437499999999998, 14.475, 14.5125, 14.549999999999999, 14.587499999999999, 14.624999999999998, 14.6625, 14.7, 14.737499999999999, 14.774999999999999, 14.812499999999998, 14.85, 14.8875, 14.924999999999999, 14.962499999999999, 14.999999999999998, 15.0375, 15.075, 15.112499999999999, 15.149999999999999, 15.187499999999998, 15.225, 15.2625, 15.299999999999999, 15.337499999999999, 15.374999999999998, 15.4125, 15.45, 15.487499999999999, 15.524999999999999, 15.562499999999998, 15.6, 15.6375, 15.674999999999999, 15.712499999999999, 15.749999999999998, 15.7875, 15.825, 15.862499999999999, 15.899999999999999, 15.937499999999998, 15.975, 16.0125, 16.05, 16.087500000000002, 16.125, 16.1625, 16.2, 16.2375, 16.275000000000002, 16.3125, 16.35, 16.3875, 16.425, 16.462500000000002, 16.5, 16.5375, 16.575, 16.6125, 16.650000000000002, 16.6875, 16.725, 16.7625, 16.8, 16.837500000000002, 16.875, 16.9125, 16.95, 16.9875, 17.025000000000002, 17.0625, 17.1, 17.1375, 17.175, 17.212500000000002, 17.25, 17.2875, 17.325, 17.3625, 17.400000000000002, 17.4375, 17.475, 17.5125, 17.55, 17.587500000000002, 17.625, 17.6625, 17.7, 17.7375, 17.775000000000002, 17.8125, 17.85, 17.8875, 17.925, 17.962500000000002, 18.0, 18.0375, 18.075, 18.1125, 18.150000000000002, 18.1875, 18.225, 18.2625, 18.3, 18.337500000000002, 18.375, 18.4125, 18.45, 18.4875, 18.525000000000002, 18.5625, 18.6, 18.6375, 18.675, 18.712500000000002, 18.75, 18.7875, 18.825, 18.8625, 18.900000000000002, 18.9375, 18.975, 19.0125, 19.05, 19.087500000000002, 19.125, 19.1625, 19.2, 19.2375, 19.275000000000002, 19.3125, 19.35, 19.3875, 19.425, 19.462500000000002, 19.5, 19.5375, 19.575, 19.6125, 19.650000000000002, 19.6875, 19.725, 19.7625, 19.8, 19.837500000000002, 19.875, 19.9125, 19.95, 19.9875, 20.025000000000002, 20.0625, 20.1, 20.1375, 20.175, 20.212500000000002, 20.25, 20.2875, 20.325, 20.3625, 20.400000000000002, 20.4375, 20.475, 20.5125, 20.55, 20.587500000000002, 20.625, 20.6625, 20.7, 20.7375, 20.775000000000002, 20.8125, 20.85, 20.8875, 20.925, 20.962500000000002, 21.0]
  out "Offline Pulse Energy":dbl=5.1516399999999996
  out "Online Pulse Energy":dbl=5.150377142857143
  in  "Instrument Control":T5(tab)
  in  "Device In":refnum<visa-resource-name>="GPIB0::10::INSTR"
  in  "Settings":T6={"Module"=enum."WV Online TEC", "WV Online TEC"=23.205500000000487, "WV Online LD"=0.175, "WV Offline TEC"=29.665500000000158, "WV Offline LD"=0.17, "WV Etalon TEC"=28.0, "HSRL Etalon TEC"=25.954, "HSRL TEC"=14.283999999999752, "HSRL LD"=0.16} {"HSRL LD" min=0.0 max=0.18 step=0.001 format="%.3p"; "HSRL TEC" min=14.0 max=28.0 step=0.1 format="%.3g"; "WV Offline LD" min=0.0 max=0.18 step=0.001 format="%.3p"; "WV Online LD" min=0.0 max=0.18 step=0.001 format="%.3p"; "HSRL Etalon TEC" format="%.2g"; "WV Etalon TEC" format="%.2g"; "WV Offline TEC" min=16.0 max=30.0 step=0.1 format="%.3g"; "WV Online TEC" min=14.0 max=28.0 step=0.1 format="%.3g"}
  out "Readings":T7={"Pro8000"=TRUE, "WV OnLine TEC"=23.2111759, "WV Online TEC"=TRUE, "WV Online LD"=0.175140634, "WV Online LD"=TRUE, "WV Offline TEC"=29.6786747, "WV Offline TEC"=TRUE, "WV Offline LD"=0.170392588, "WV Offline LD"=TRUE, "WV EtalonTEC"=28.1596336, "WV Etalon TEC"=TRUE, "HSRL Etalon TEC"=25.9497223, "HSRL Etalon TEC"=TRUE, "HSRL TEC"=14.2950993, "HSRL TEC "=TRUE, "HSRL LD"=0.160255864, "HSRL LD"=TRUE} {"HSRL LD" format="%.3p"; "HSRL TEC" format="%.3g"; "WV Offline LD" format="%.3p"; "WV Online LD" format="%.3p"; "HSRL Etalon TEC" format="%.3g"; "WV EtalonTEC" format="%.3g"; "WV Offline TEC" format="%.3g"; "WV OnLine TEC" format="%.3g"}
  in  "Pulse B Polarity":enum32{"Low", "High"}(ring)=enum."High"
  in  "Pulse A Delay(ns)":u32=1040 min=80 max=327600
  in  "Pulse B Delay(ns)":u32=170000 min=80 max=327600 step=1
  in  "Accumulation Delay(ns)":u32=10 min=10 max=1270 step=1
  in  "Sync Pulse Polarity":enum32{"Low", "High"}(ring)=enum."High"
  in  "Pulse A Polarity":enum32{"Low", "High"}(ring)=enum."High"
  in  "Number of Bins":u32=560 min=2 max=4095 step=1
  in  "Number of Accumulates":u32=14285 min=1 max=32767 step=1
  in  "Time Resolution Per Bin(ns)":u32=250 min=5 max=1063 step=1
  out "AMCS_Profile":i32=48167
  in  "WV Online Set (nm)":dbl=828.199 format="%.5f"
  out "WV Online Read (nm)":dbl=828.1990659212818 format="%.5f"
  out "WV Offline Read (nm)":dbl=828.2985780982586 format="%.5f"
  in  "WV Offline Set (nm)":dbl=828.29865 format="%.5f"
  in  "Bristol In":i32=5
  out "Bristol Out":i32
  out "Online_Diff":dbl=6.592128181637236e-05 format="%#_3e"
  out "Oflline_Diff":dbl=-7.190174130755622e-05 format="%#_3e"
  out "WV Online Locked":bool=TRUE
  out "WV Oflline Locked":bool=TRUE
  in  "calculate absorption cross sections":bool
  in  "Online_Tol":dbl=7.5e-05 format="%#_15g"
  in  "Cancel online":bool
  in  "Offline_Tol":dbl=7.5e-05 format="%#_15g"
  in  "Cancel Offline":bool
  in  "temp step size":dbl=0.00025 format="%#_6p"
  in  "HSRL_Tol":dbl=7.5e-05 format="%#_15g"
  out "HSRL_Diff":dbl=-7.235308771669224e-05 format="%#_3e"
  in  "Cancel HSRL":bool
  out "HSRL Locked":bool=TRUE
  out "HSRL Read (nm)":dbl=780.2460476469123 format="%.5f"
  in  "HSRL Set (nm)":dbl=780.24612 format="%#.5f"
  in  "Smoothing Range":dbl=150.0
  in  "Total DIAL Integration Time (Minutes)":i32=3
  in  "Data Reads (number of loops)":i32=1
  in  "Total Aerosol Integration Time (Minutes)":dbl=0.5
  in  "Scalar Wait Time":u32
  out "Smoothed Bins":dbl=4.0
  in  "NewportIn":string
  in  "logging":bool
  out "Newport Device Key":string="1918-R 15120"
  in  "SampleSize":i32=2
  out "NewportRef":refnum<k24>
  in  "Switch Comm Port":refnum<visa-resource-name>="COM3"
  out "FF_On_Ref":refnum<file>
  out "FF_On_Ptr":i64=1870064 format="%.2p"
  out "FF_Off_Ref":refnum<file>
  out "FF_Off_Ptr":i64=1870064 format="%.2p"
  out "NF_On_Ref":refnum<file>
  out "NF_On_Ptr":i64=1870064 format="%.2p"
  out "NF_Off_Ref":refnum<file>
  out "NF_Off_Ptr":i64=1870064 format="%.2p"
  out "DataOpen":bool=TRUE
  out "File Path_Far Field (out)":string="C:\\Users\\H2ODial\\Desktop\\SharedTeleWVData\\170505FF\\22"
  out "File Path_Near Field (out)":string="C:\\Users\\H2ODial\\Desktop\\SharedTeleWVData\\170505NF\\22"
  in  "Data File DIR (in)":string="C:\\Users\\H2ODial\\Desktop\\SharedTeleWVData\\"
  out "TRHP":T8={"Temp C"=25.047466422466428, "RelH %"=19.406288156288156, "Press hPa"=836.4285714285714, "AbH g/m^3"=4.471916971916972}
  in  "WS visa":refnum<visa-resource-name>="COM6"
  in  "WS_On/Off":bool=TRUE
  in  "bins":u32=560 min=2 max=4095 step=1
  out "y offset":u32=10
  in  "ns scale":u32=250
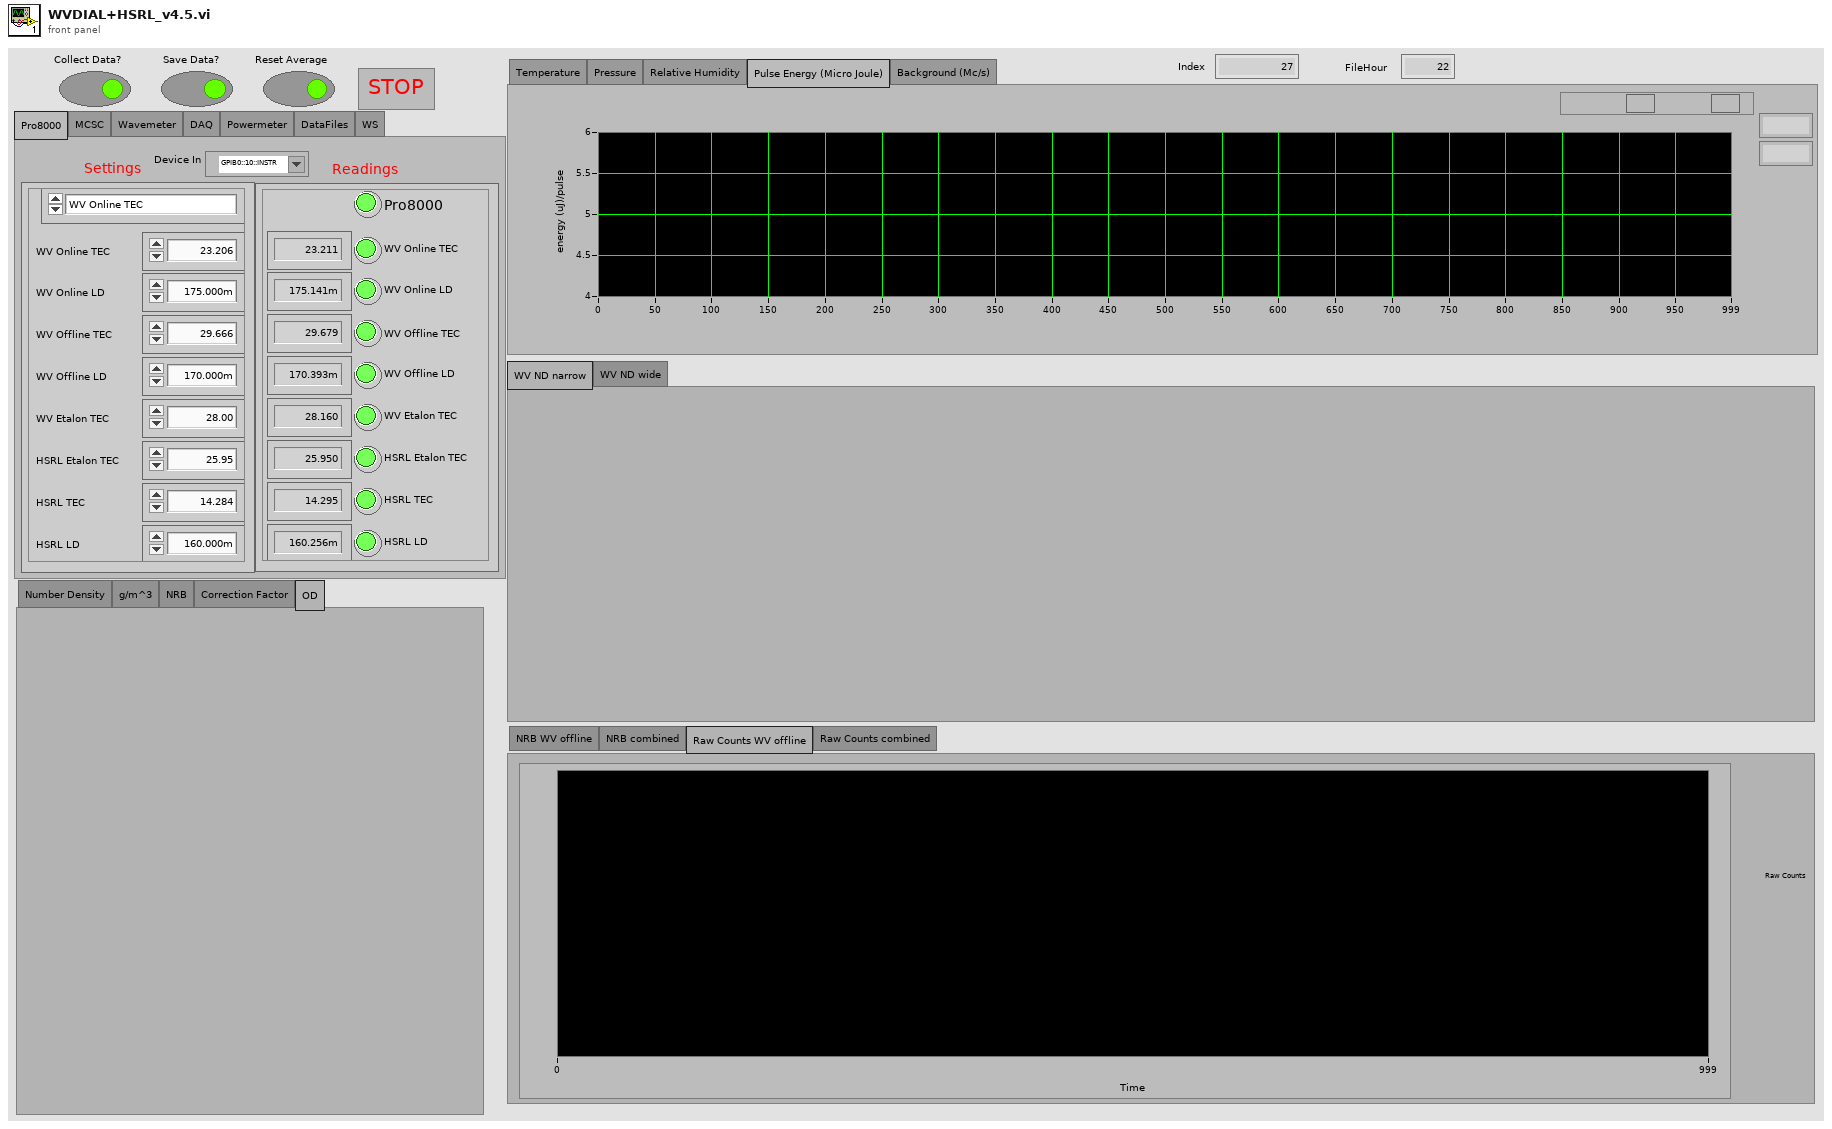
[diagram p1: front panel]
types:
  T1 = enum32{"NRB WV offline", "NRB combined", "Raw Counts WV offline", "Raw Counts combined"}
  T2 = enum32{"Number Density", "g/m^3", "NRB", "Correction Factor", "OD"}
  T3 = enum32{"Temperature", "Pressure", "Relative Humidity", "Pulse Energy (Micro Joule)", "Background (Mc/s)"}
  T4 = cluster{"Online Pulse Energy":dbl, "Pulse Energy Offline":dbl}
  T5 = enum32{"Pro8000", "MCSC", "Wavemeter", "DAQ", "Powermeter", "DataFiles", "WS"}
  T6 = cluster{"Module":enum16{"WV Online TEC", "WV Online LD", "WV Offline TEC", "WV Offline LD", "WV Etalon TEC", "HSRL Etalon TEC", "HSRL TEC", "HSRL LD"}, "WV Online TEC":dbl, "WV Online LD":dbl, "WV Offline TEC":dbl, "WV Offline LD":dbl, "WV Etalon TEC":dbl, "HSRL Etalon TEC":dbl, "HSRL TEC":dbl, "HSRL LD":dbl}
  T7 = cluster{"Pro8000":bool, "WV OnLine TEC":dbl, "WV Online TEC":bool, "WV Online LD":dbl, "WV Online LD":bool, "WV Offline TEC":dbl, "WV Offline TEC":bool, "WV Offline LD":dbl, "WV Offline LD":bool, "WV EtalonTEC":dbl, "WV Etalon TEC":bool, "HSRL Etalon TEC":dbl, "HSRL Etalon TEC":bool, "HSRL TEC":dbl, "HSRL TEC ":bool, "HSRL LD":dbl, "HSRL LD":bool}
  T8 = cluster{"Temp C":dbl, "RelH %":dbl, "Press hPa":dbl, "AbH g/m^3":dbl}
  T9 = enum16{"Open_TL", "Close_TL", "Verify_ID", "TEC_Sensor", "SET", "READ", "ON", "OFF", "Set_Limits", "Read_Limits", "Enable_Status", "Read_Status"}
  T10 = enum16{"Initialize ILX", "Set ON T", "Set Off T", "Set ON I", "Set Off I", "Set On Lim", "Set Off Lim", "Read ILX", "TEC ON/OFF", "LASER ON/OFF", "Status?", "ILX OFF"}
  T11 = enum16{"open", "replace", "create", "open or create", "replace or create", "replace or create with confirmation"}
  T12 = enum16{"WV Online TEC", "WV Online LD", "WV Offline TEC", "WV Offline LD", "WV Etalon TEC", "HSRL Etalon TEC", "HSRL TEC", "HSRL LD"}
  T13 = cluster{"Temp":dbl, "RelH":dbl, "Press":dbl, "AbH":dbl}
  T14 = typedef "LVDateTimeRec.ctl" = cluster{"fractional second":dbl, "second":i32, "minute":i32, "hour":i32, "day of month":i32, "month":i32, "year":i32, "day of week":i32, "day of year":i32, "DST":i32}
  T15 = cluster{"Online Pulse Energy":dbl, "Offline Pulse Energy":dbl}
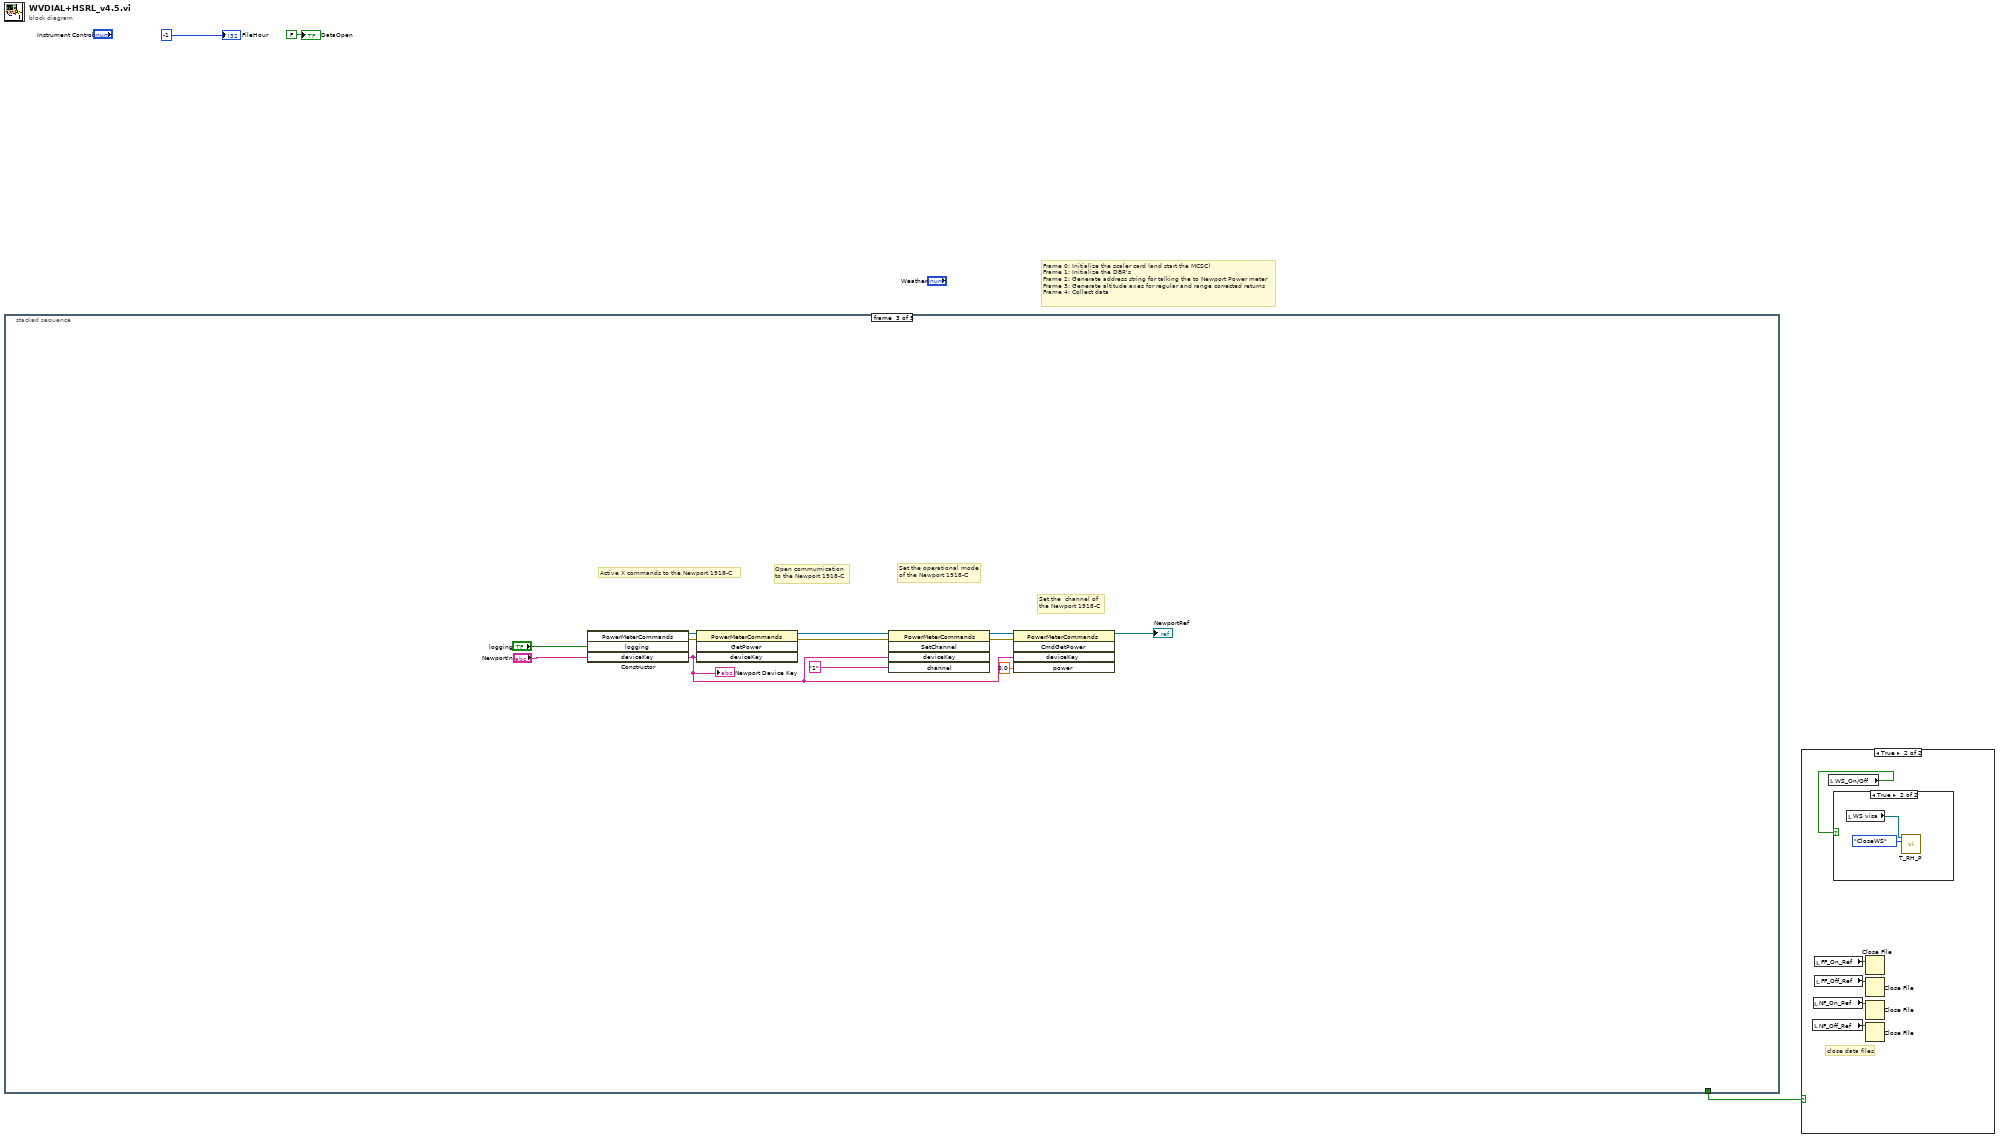
[diagram p0: block diagram]
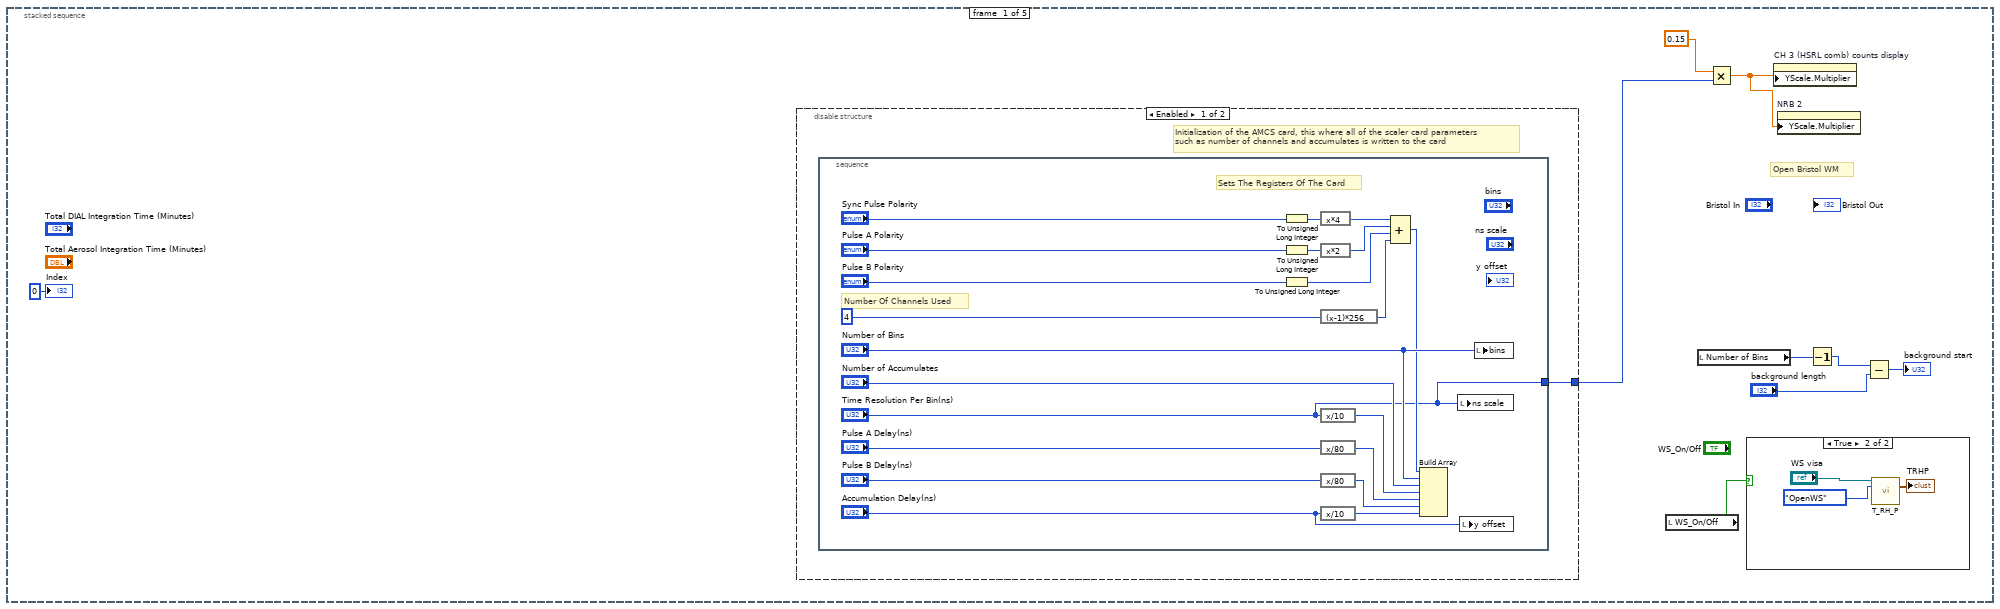
[diagram p4: hidden frame]
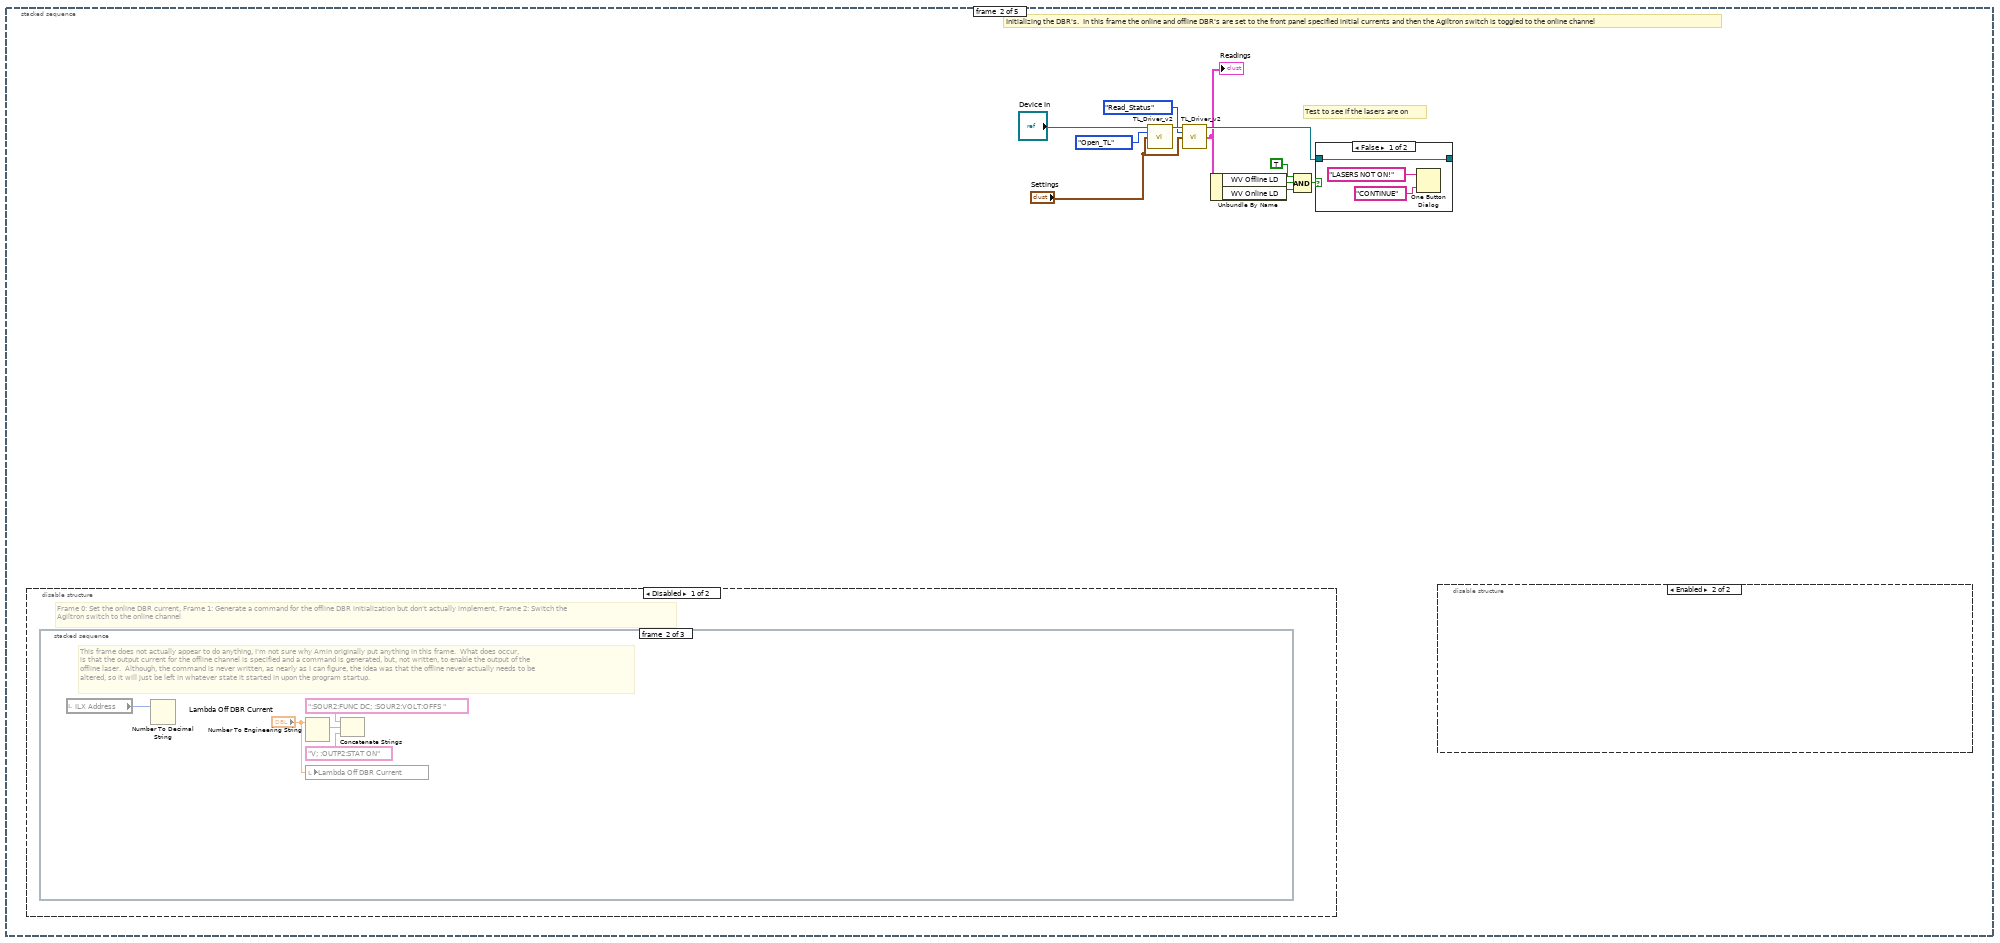
[diagram p7: hidden frame]
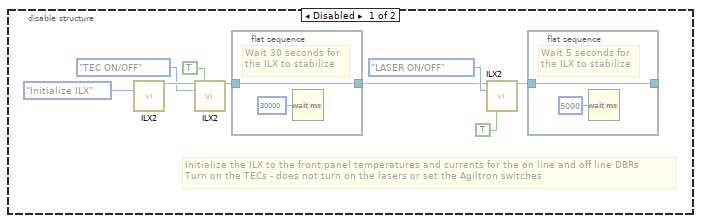
[diagram p9: hidden frame]
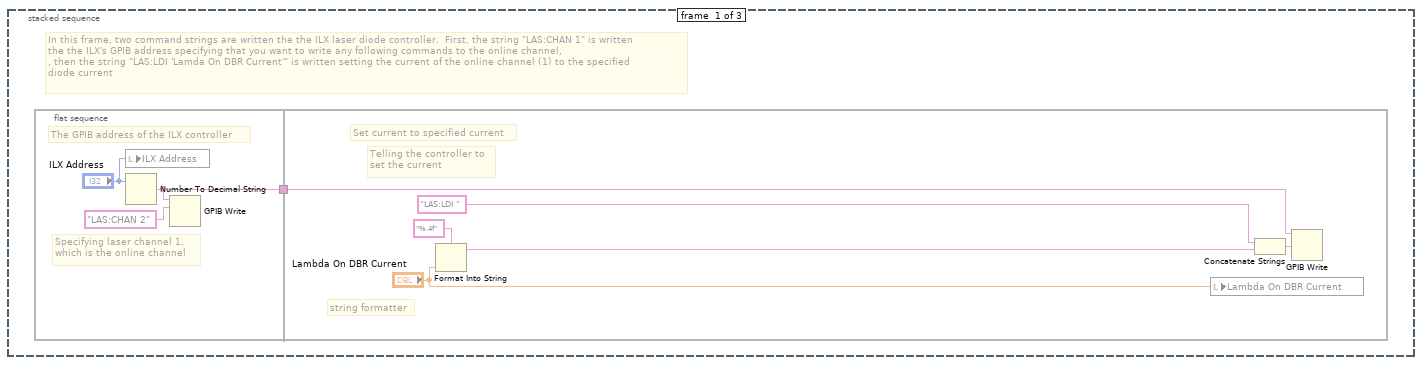
[diagram p10: hidden frame]
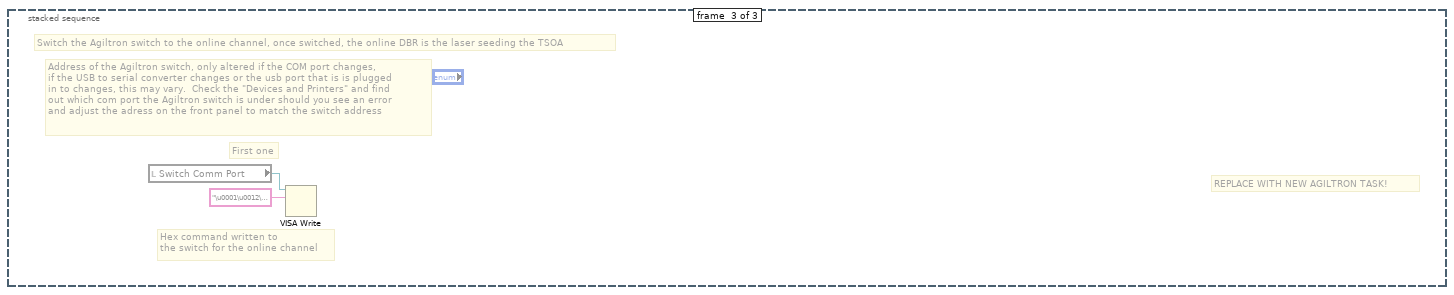
[diagram p11: hidden frame]
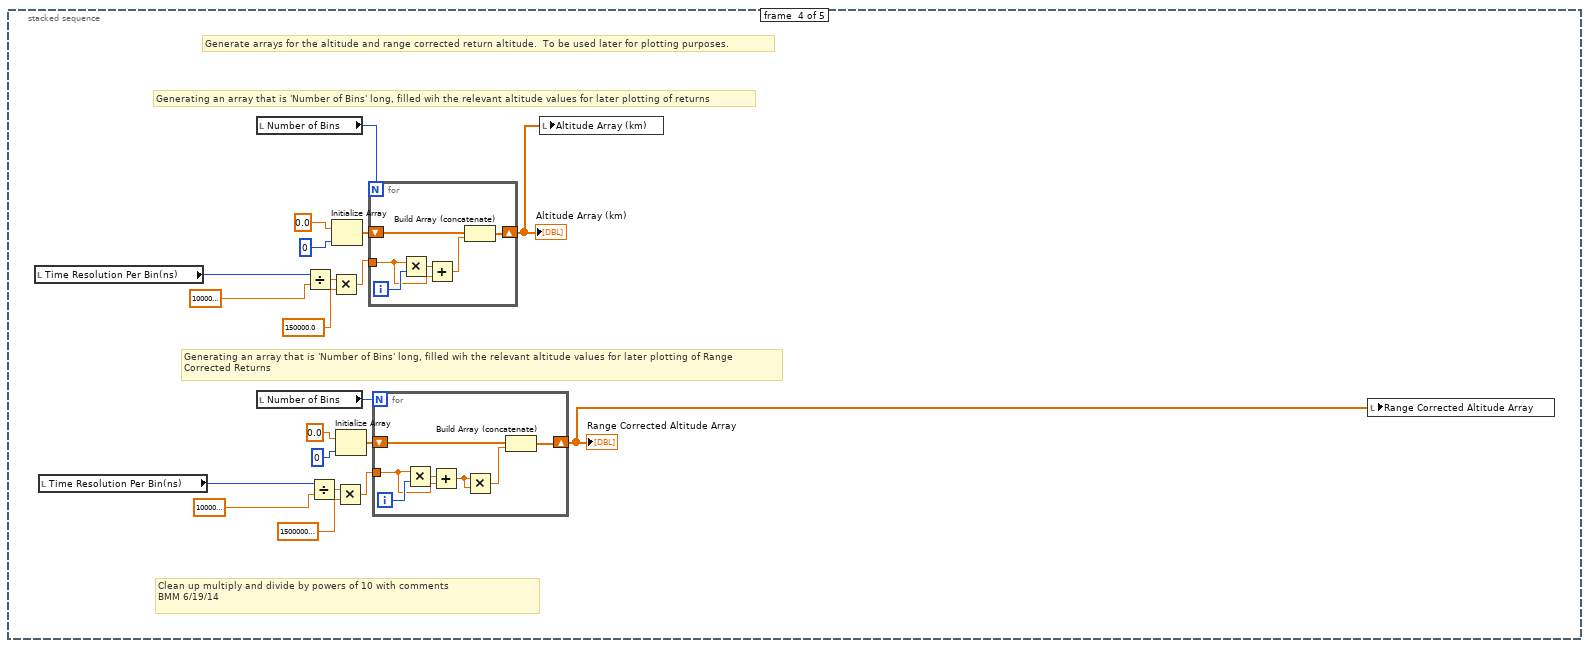
[diagram p13: hidden frame]
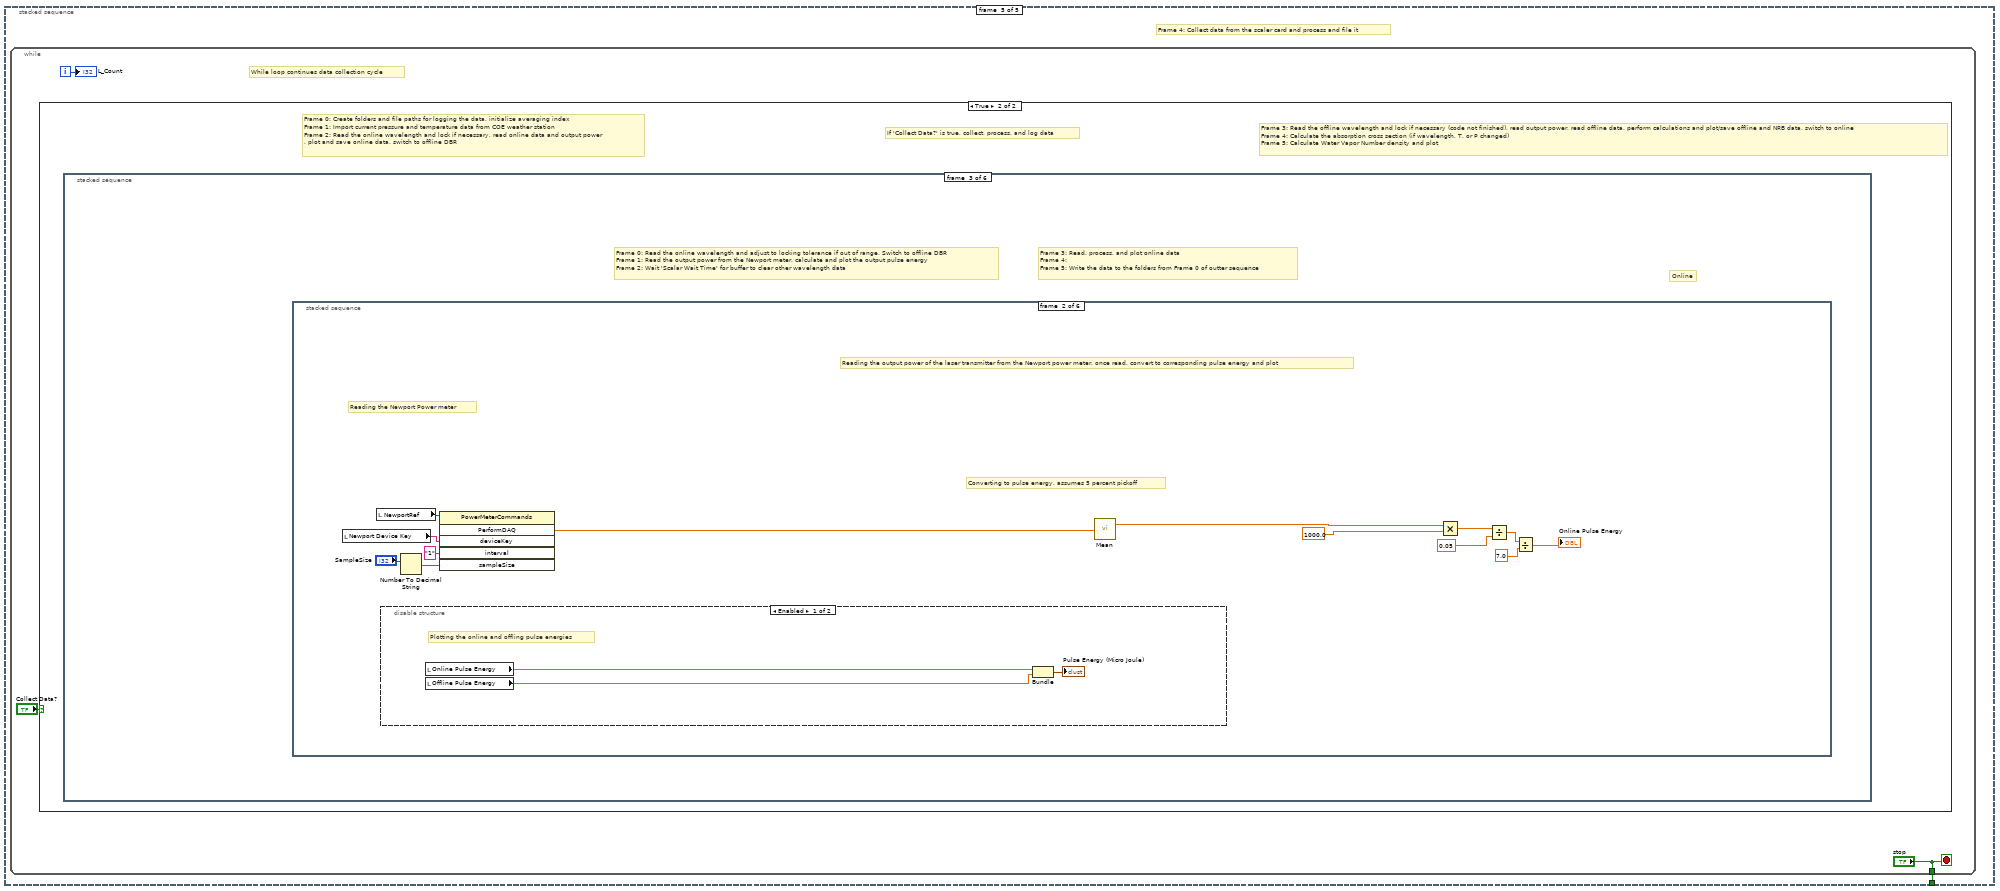
[diagram p14: hidden frame]
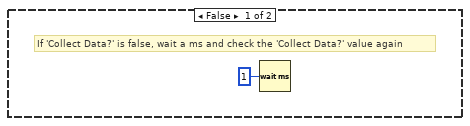
[diagram p15: hidden frame]
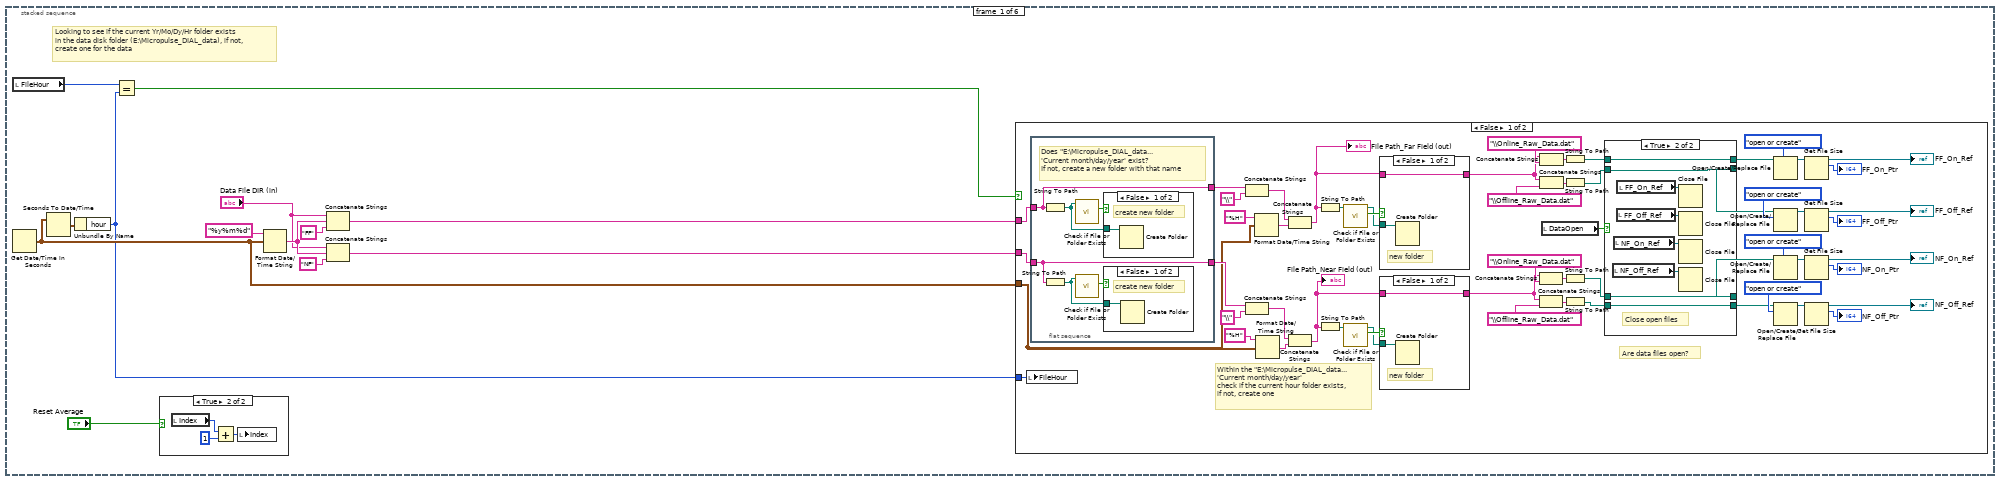
[diagram p16: hidden frame]
diagram:
  # "Frame 0: Initialize the scaler card (and start the MCSC)\nFrame 1: Initialize the DBR's\nFrame 2: Generate address string for talking the to Newport Power meter\nFrame 3: Generate altitude axes for regular and range corrected returns\nFrame 4: Collect data"
  n1 = stacked-sequence {
    tunnel: [_ _ _ _ w128] -> w3
    frame #0 {
      # "Open Bristol WM"
      n2 = disable-structure shown="Enabled" {
        disable-tunnel: [w16 _] -> w5
        frame Enabled {
          # "Initialization of the AMCS card, this where all of the scaler card parameters\nsuch as number of channels and accumulates is written to the card"
          n3 = stacked-sequence {
            tunnel: ["Time Resolution Per Bin(ns)"] -> w16
            frame #0 {
              # "Sets The Registers Of The Card"
              # "Number Of Channels Used"
              n4 = To Unsigned Long Integer(number="Sync Pulse Polarity") -> (unsigned 32bit integer=w18:u32)
              n5 = To Unsigned Long Integer(number="Pulse A Polarity") -> (unsigned 32bit integer=w22:u32)
              n6 = To Unsigned Long Integer(number="Pulse B Polarity") -> (unsigned 32bit integer=w20:u32)
              n7 = expression code="x*4"(w18) -> (w27:u32)
              n8 = expression code="x*2"(w22) -> (w26:u32)
              n9 = expression code="(x-1)*256"(u32 4 ("Number of Channels Used")) -> (w25:u32)
              n10 = expression code="x/10"("Time Resolution Per Bin(ns)") -> (w28:u32)
              n11 = expression code="x/80"("Pulse A Delay(ns)") -> (w35:u32)
              n12 = expression code="x/80"("Pulse B Delay(ns)") -> (w37:u32)
              n13 = expression code="x/10"("Accumulation Delay(ns)") -> (w36:u32)
              n14 = Compound Arithmetic op=ADD(w27, w26, w20, w25) -> (w24:u32)
              n15 = Build Array(w24, "Number of Bins", "Number of Accumulates", w28, w35, w37, w36) -> ()  [unwired: 1 out]
              n16 = local write "ns scale"("Time Resolution Per Bin(ns)") -> ()
              n17 = local write "y offset"("Accumulation Delay(ns)") -> ()
              n18 = local write "bins"("Number of Bins") -> ()
            }
          }
        }
        frame Disabled {
        }
      }
      n19 = local read "WS_On/Off"() -> (w7:bool)
      n20 = local read "Number of Bins"() -> (w11:u32)
      n21 = Multiply(x=0.15, y=w5) -> (x*y=w4:dbl)
      n22 = case shown="True" w7 {
        frame False {
        }
        frame True {
          n23 = call "T_RH_P.vi"("VISA in"="WS visa", "WS_Commands"=enum16{"OpenWS", "ReadTRHP", "CloseWS"}."OpenWS") -> ("TRHP"=→"TRHP":T13)  [unwired: 11 in, 2 out]
        }
      }
      n24 = property on="CH 3 (HSRL comb) counts display" class="IntChart (strict)"("YScale.Multiplier"=w4) -> ()  [unwired: 2 in, 2 out]
      n25 = property on="NRB 2" class="IntChart (strict)"("YScale.Multiplier"=w4) -> ()  [unwired: 2 in, 2 out]
      n26 = Decrement(x=w11) -> (x-1=w10:u32)
      n27 = Subtract(x=w10, y="background length") -> (x-y=→"background start":u32)
      "Index" <- 0 ("Index")
    }
    frame #1 {
      # "Test to see if the lasers are on"
      # "Initializing the DBR's.  In this frame the online and offline DBR's are set to the front panel specified initial currents and then the Agiltron switch is toggled to the online channel"
      n28 = disable-structure shown="Disabled" {
        frame Disabled {
          # "Frame 0: Set the online DBR current, Frame 1: Generate a command for the offline DBR initialization but don't actually implement, Frame 2: Switch the \nAgiltron switch to the online channel"
          n29 = stacked-sequence {
            frame #0 {
              # "In this frame, two command strings are written the the ILX laser diode controller.  First, the string \"LAS:CHAN 1\" is written\nthe the ILX's GPIB address specifying that you want to write any following commands to the online channel,\n, then the string \"LAS:LDI 'Lamda On DBR Current'\" is written setting the current of the online channel (1) to the specified \ndiode current"
              n30 = flat-sequence {
                tunnel: [w68] -> w66
                tunnel: w66 -> [w70]
                frame #0 {
                  # "The GPIB address of the ILX controller"
                  # "Specifying laser channel 1,\nwhich is the online channel"
                  n31 = local write "ILX Address"("ILX Address") -> ()
                  n32 = Number To Decimal String(number="ILX Address") -> (decimal integer string=w68:string)  [unwired: 1 in]
                  n33 = GPIB Write(0:w68, 1:"LAS:CHAN 2") -> ()  [unwired: 3 in, 2 out]
                }
                frame #1 {
                  # "Telling the controller to\nset the current"
                  # "string formatter"
                  # "Set current to specified current"
                  n34 = Format Into String(format string="%.4f" ("Format String"), "Lambda On DBR Current") -> (resulting string=w73:string)  [unwired: 2 in, 1 out]
                  n35 = local write "Lambda On DBR Current"("Lambda On DBR Current") -> ()
                  n36 = Concatenate Strings("LAS:LDI ", w73) -> (w74:string)
                  n37 = GPIB Write(0:w70, 1:w74) -> ()  [unwired: 3 in, 2 out]
                }
              }
            }
            frame #1 {
              # "This frame does not actually appear to do anything, I'm not sure why Amin originally put anything in this frame.  What does occur, \nis that the output current for the offline channel is specified and a command is generated, but, not written, to enable the output of the\noffline laser.  Although, the command is never written, as nearly as I can figure, the idea was that the offline never actually needs to be \naltered, so it will just be left in whatever state it started in upon the program startup."
              n38 = local read "ILX Address"() -> (w76:i32)
              n39 = Number To Decimal String(number=w76) -> ()  [unwired: 1 in, 1 out]
              n40 = Number To Engineering String(4:"Lambda Off DBR Current") -> (0:w80:string)  [unwired: 3 in]
              n41 = local write "Lambda Off DBR Current"("Lambda Off DBR Current") -> ()
              n42 = Concatenate Strings(":SOUR2:FUNC DC; :SOUR2:VOLT:OFFS ", w80, "V; :OUTP2:STAT ON") -> ()  [unwired: 1 out]
            }
            frame #2 {
              # "REPLACE WITH NEW AGILTRON TASK!"
              # "First one"
              # "Address of the Agiltron switch, only altered if the COM port changes,\nif the USB to serial converter changes or the usb port that is is plugged\nin to changes, this may vary.  Check the \"Devices and Printers\" and find \nout which com port the Agiltron switch is under should you see an error \nand adjust the adress on the front panel to match the switch address"
              # "Hex command written to \nthe switch for the online channel"
              # "Switch the Agiltron switch to the online channel, once switched, the online DBR is the laser seeding the TSOA"
              n43 = local read "Switch Comm Port"() -> (w81:refnum<visa-resource-name>)
              n44 = VISA Write(VISA resource name=w81, write buffer="\u0001\u0012\u0000\u0002") -> ()  [unwired: 1 in, 3 out]
            }
          }
        }
        frame Enabled {
        }
      }
      n45 = call "TL_Driver_v2.vi"("Device In"="Device In", "Commands"=T9."Open_TL", "Settings"="Settings") -> ("Device Out"=w46:refnum<visa-resource-name>)  [unwired: 9 in, 3 out]
      n46 = call "TL_Driver_v2.vi"("Device In"=w46, "Commands"=T9."Read_Status", "Settings"="Settings") -> ("Device Out"=w44:refnum<visa-resource-name>, "Readings"=w38:T7)  [unwired: 9 in, 2 out]
      "Readings" <- w38
      n47 = Unbundle By Name(w38) -> ("WV Offline LD"=w41:bool, "WV Online LD"=w42:bool)
      n48 = Compound Arithmetic op=AND(TRUE, w41, w42) -> (w40:bool)
      n49 = case shown="False" w40 {
        tunnel: w44 -> [w49 w52]
        tunnel: [w49 w52] -> _
        frame False {
          n50 = One Button Dialog(message="LASERS NOT ON!", button name ("OK")="CONTINUE") -> ()  [unwired: 1 out]
        }
        frame True {
        }
      }
      n51 = disable-structure shown="Enabled" {
        frame Disabled {
          # "Initialize the ILX to the front panel temperatures and currents for the on line and off line DBRs\nTurn on the TECs - does not turn on the lasers or set the Agiltron switches"
          n52 = call "ILX2.vi"("ILX Command"=T10."Initialize ILX") -> ("Device Out"=w60:refnum<visa-resource-name>)  [unwired: 10 in, 4 out]
          n53 = call "ILX2.vi"("Device In"=w60, "TEC Control"=TRUE, "ILX Command"=T10."TEC ON/OFF") -> ("Device Out"=w57:refnum<visa-resource-name>)  [unwired: 8 in, 4 out]
          n54 = flat-sequence {
            tunnel: w57 -> [w64]
            tunnel: [w64] -> w54
            frame #0 {
              # "Wait 30 seconds for\nthe ILX to stabilize"
              n55 = Wait (ms)(milliseconds to wait=u32 30000) -> ()  [unwired: 1 out]
            }
          }
          n56 = call "ILX2.vi"("Device In"=w54, "ILX Command"=T10."LASER ON/OFF", "Laser Control"=TRUE ("TEC Control")) -> ("Device Out"=w53:refnum<visa-resource-name>)  [unwired: 8 in, 4 out]
          n57 = flat-sequence {
            tunnel: w53 -> [w62]
            tunnel: [w62] -> _
            frame #0 {
              # "Wait 5 seconds for\nthe ILX to stabilize"
              n58 = Wait (ms)(milliseconds to wait=u32 5000) -> ()  [unwired: 1 out]
            }
          }
        }
        frame Enabled {
        }
      }
    }
    frame #2 {
      # "Active X commands to the Newport 1918-C"
      # "Set the  channel of\nthe Newport 1918-C"
      # "Set the operational mode\nof the Newport 1918-C"
      # "Open commumication\nto the Newport 1918-C"
      n59 = constructor class="PowerMeterCommands"("logging"="logging", "deviceKey"="NewportIn") -> (reference out=w94:refnum<k24>, error out=w91:errorcluster, "deviceKey"=w86:string)  [unwired: 3 in, 2 out]
      "Newport Device Key" <- w86
      n60 = invoke class="PowerMeterCommands" method="GetPower"(reference=w94, error in=w91, "deviceKey"=w86) -> (reference out=w93:refnum<k24>, error out=w90:errorcluster)  [unwired: 1 in, 2 out]
      n61 = invoke class="PowerMeterCommands" method="SetChannel"(reference=w93, error in=w90, "deviceKey"=w86, "channel"="1") -> (reference out=w87:refnum<k24>, error out=w89:errorcluster)  [unwired: 1 in, 3 out]
      n62 = invoke class="PowerMeterCommands" method="CmdGetPower"(reference=w87, error in=w89, "deviceKey"=w86, "power"=sgl 0.0) -> (reference out=→"NewportRef":refnum<k24>)  [unwired: 1 in, 4 out]
    }
    frame #3 {
      # "Clean up multiply and divide by powers of 10 with comments\nBMM 6/19/14"
      # "Generating an array that is 'Number of Bins' long, filled wih the relevant altitude values for later plotting of Range \nCorrected Returns"
      # "Generating an array that is 'Number of Bins' long, filled wih the relevant altitude values for later plotting of returns"
      # "Generate arrays for the altitude and range corrected return altitude.  To be used later for plotting purposes."
      n63 = local read "Time Resolution Per Bin(ns)"() -> (w107:u32)
      n64 = local read "Time Resolution Per Bin(ns)"() -> (w97:u32)
      n65 = local read "Number of Bins"() -> (w110:u32)
      n66 = local read "Number of Bins"() -> (w100:u32)
      n67 = Divide(x=w107, y=1000000000.0) -> (x/y=w105:dbl)
      n68 = Divide(x=w97, y=1000000000.0) -> (x/y=w95:dbl)
      n69 = Multiply(x=w105, y=150000.0) -> (x*y=w108:dbl)
      n70 = Initialize Array(0.0, 0) -> (w113:dbl[])
      n71 = Multiply(x=w95, y=150000000.0) -> (x*y=w98:dbl)
      n72 = Initialize Array(0.0, 0) -> (w103:dbl[])
      n73 = for {
        N: w110 -> [_]
        shift-right: [w126] -> w111
        shift-left: w113 -> [w127]
        tunnel: w108 -> [w123]
        i -> [w125]
        n74 = Multiply(x=w123, y=w125) -> (x*y=w124:dbl)
        n75 = Add(x=w124, y=w123) -> (x+y=w122:dbl)
        n76 = Build Array (concatenate)(w127, w122) -> (w126:dbl[])
      }
      "Altitude Array (km)" <- w111
      n77 = for {
        N: w100 -> [_]
        shift-right: [w120] -> w101
        shift-left: w103 -> [w121]
        tunnel: w98 -> [w116]
        i -> [w119]
        n78 = Multiply(x=w116, y=w119) -> (x*y=w117:dbl)
        n79 = Add(x=w117, y=w116) -> (x+y=w115:dbl)
        n80 = Multiply(x=w115, y=w115) -> (x*y=w118:dbl)
        n81 = Build Array (concatenate)(w121, w118) -> (w120:dbl[])
      }
      "Range Corrected Altitude Array" <- w101
      n82 = local write "Altitude Array (km)"(w111) -> ()
      n83 = local write "Range Corrected Altitude Array"(w101) -> ()
    }
    frame #4 {
      # "Frame 4: Collect data from the scaler card and process and file it"
      n84 = while {
        tunnel: ["stop"] -> w128
        i -> [w129]
        stop <- "stop" stop-if-true
        # "While loop continues data collection cycle"
        n85 = case shown="True" "Collect Data?" {
          frame False {
            # "If 'Collect Data?' is false, wait a ms and check the 'Collect Data?' value again"
            n86 = Wait (ms)(milliseconds to wait=u32 1) -> ()  [unwired: 1 out]
          }
          frame True {
            # "Frame 3: Read the offline wavelength and lock if necessary (code not finished), read output power, read offline data, perform calculations and plot/save offline and NRB data, switch to online\nFrame 4: Calculate the absorption cross section (if wavelength, T, or P changed)\nFrame 5: Calculate Water Vapor Number density and plot"
            # "Frame 0: Create folders and file paths for logging the data, initialize averaging index\nFrame 1: Import current pressure and temperature data from COE weather station\nFrame 2: Read the online wavelength and lock if necessary, read online data and output power\n, plot and save online data, switch to offline DBR"
            # "If 'Collect Data?' is true, collect, process, and log data"
            n87 = stacked-sequence {
              frame #0 {
                # "Looking to see if the current Yr/Mo/Dy/Hr folder exists\nin the data disk folder (E:\\Micropulse_DIAL_data), if not,\ncreate one for the data"
                n88 = local read "FileHour"() -> (w142:i32)
                n89 = Get Date/Time In Seconds() -> (seconds since 1Jan1904=w134:timestamp)
                n90 = Seconds To Date/Time(time stamp (now)=w134) -> (date time rec=w144:T14)  [unwired: 1 in]
                n91 = Unbundle By Name(w144) -> ("hour"=w133:i32)
                n92 = Equal?(x=w142, y=w133) -> (x = y?=w143:bool)
                n93 = case shown="True" "Reset Average" {
                  frame False {
                    n94 = local write "Index"(0 ("Index")) -> ()
                  }
                  frame True {
                    n95 = local read "Index"() -> (w232:i32)
                    n96 = Add(x=w232, y=1) -> (x+y=w231:i32)
                    n97 = local write "Index"(w231) -> ()
                  }
                }
                n98 = Format Date/Time String(time format string (%c)="%y%m%d", seconds (now)=w134) -> (date/time string=w138:string)  [unwired: 1 in]
                n99 = Concatenate Strings("Data File DIR (in)", w138, "FF" ("string")) -> (w140:string)
                n100 = Concatenate Strings("Data File DIR (in)", w138, "NF" ("string")) -> (w135:string)
                n101 = case shown="False" w143 {
                  tunnel: w140 -> [w202 _]
                  tunnel: w135 -> [w201 _]
                  tunnel: w134 -> [w188 _]
                  tunnel: w133 -> [w164 _]
                  frame False {
                    # "Are data files open?"
                    # "Within the \"E:\\Micropulse_DIAL_data...\n'Current month/day/year' \ncheck if the current hour folder exists,\nif not, create one"
                    n102 = local write "FileHour"(w164) -> ()
                    n103 = flat-sequence {
                      tunnel: [w222] -> w189
                      tunnel: w202 -> [w221]
                      tunnel: w201 -> [w222]
                      tunnel: [w221] -> w190
                      frame #0 {
                        # "Does \"E:\\Micropulse_DIAL_data...\n'Current month/day/year' exist?\nIf not, create a new folder with that name"
                        n104 = String To Path(string=w221) -> (path=w226:path)
                        n105 = String To Path(string=w222) -> (path=w224:path)
                        n106 = call <vilib>:"Check if File or Folder Exists.vi"("path"=w226) -> ("file or folder exists?"=w225:bool)  [unwired: 8 in, 2 out]
                        n107 = call <vilib>:"Check if File or Folder Exists.vi"("path"=w224) -> ("file or folder exists?"=w223:bool)  [unwired: 8 in, 2 out]
                        n108 = case shown="False" w225 {
                          tunnel: w226 -> [w228 _]
                          frame False {
                            # "create new folder"
                            n109 = Create Folder(path (use dialog)=w228) -> ()  [unwired: 2 in, 3 out]
                          }
                          frame True {
                            # "Folder exists\ndo nothing"
                          }
                        }
                        n110 = case shown="False" w223 {
                          tunnel: w224 -> [w227 _]
                          frame False {
                            # "create new folder"
                            n111 = Create Folder(path (use dialog)=w227) -> ()  [unwired: 2 in, 3 out]
                          }
                          frame True {
                            # "Folder exists\ndo nothing"
                          }
                        }
                      }
                    }
                    n112 = Concatenate Strings(w190, "\\" ("string")) -> (w197:string)
                    n113 = Concatenate Strings(w189, "\\" ("string")) -> (w192:string)
                    n114 = Format Date/Time String(time format string (%c)="%H", seconds (now)=w188) -> (date/time string=w200:string)  [unwired: 1 in]
                    n115 = Format Date/Time String(time format string (%c)="%H", seconds (now)=w188) -> (date/time string=w195:string)  [unwired: 1 in]
                    n116 = Concatenate Strings(w197, w200) -> (w160:string)
                    "File Path_Far Field (out)" <- w160
                    n117 = Concatenate Strings(w192, w195) -> (w161:string)
                    "File Path_Near Field (out)" <- w161
                    n118 = String To Path(string=w160) -> (path=w198:path)
                    n119 = String To Path(string=w161) -> (path=w193:path)
                    n120 = call <vilib>:"Check if File or Folder Exists.vi"("path"=w198) -> ("file or folder exists?"=w187:bool, "dup path"=w185:path)  [unwired: 8 in, 1 out]
                    n121 = call <vilib>:"Check if File or Folder Exists.vi"("path"=w193) -> ("file or folder exists?"=w186:bool, "dup path"=w184:path)  [unwired: 8 in, 1 out]
                    n122 = case shown="False" w187 {
                      tunnel: w185 -> [w219 _]
                      tunnel: w160 -> [w218 w220]
                      tunnel: [w218 w220] -> w158
                      frame False {
                        # "new folder"
                        n123 = Create Folder(path (use dialog)=w219) -> ()  [unwired: 2 in, 3 out]
                      }
                      frame True {
                        # "Folder exists\ndo nothing"
                      }
                    }
                    n124 = case shown="False" w186 {
                      tunnel: w184 -> [w216 _]
                      tunnel: w161 -> [w215 w217]
                      tunnel: [w215 w217] -> w159
                      frame False {
                        # "new folder"
                        n125 = Create Folder(path (use dialog)=w216) -> ()  [unwired: 2 in, 3 out]
                      }
                      frame True {
                        # "Folder exists\ndo nothing"
                      }
                    }
                    n126 = Concatenate Strings(w159, "\\Online_Raw_Data.dat" ("string")) -> (w178:string)
                    n127 = Concatenate Strings(w159, "\\Offline_Raw_Data.dat" ("string")) -> (w177:string)
                    n128 = Concatenate Strings(w158, "\\Online_Raw_Data.dat" ("string")) -> (w183:string)
                    n129 = Concatenate Strings(w158, "\\Offline_Raw_Data.dat" ("string")) -> (w182:string)
                    n130 = local read "DataOpen"() -> (w175:bool)
                    n131 = String To Path(string=w183) -> (path=w174:path)
                    n132 = String To Path(string=w182) -> (path=w173:path)
                    n133 = String To Path(string=w178) -> (path=w172:path)
                    n134 = String To Path(string=w177) -> (path=w171:path)
                    n135 = case shown="True" w175 {
                      tunnel: w174 -> [w206 w210]
                      tunnel: [w206 w210] -> w168
                      tunnel: w173 -> [w205 w209]
                      tunnel: [w205 w209] -> w167
                      tunnel: w172 -> [w204 w208]
                      tunnel: [w204 w208] -> w166
                      tunnel: [w203 w207] -> w165
                      tunnel: w171 -> [w203 w207]
                      frame False {
                        # "No files open\ndo nothing"
                      }
                      frame True {
                        # "Close open files"
                        n136 = local read "NF_Off_Ref"() -> (w212:refnum<file>)
                        n137 = local read "NF_On_Ref"() -> (w211:refnum<file>)
                        n138 = local read "FF_Off_Ref"() -> (w214:refnum<file>)
                        n139 = local read "FF_On_Ref"() -> (w213:refnum<file>)
                        n140 = Close File(refnum=w213) -> ()  [unwired: 1 in, 2 out]
                        n141 = Close File(refnum=w214) -> ()  [unwired: 1 in, 2 out]
                        n142 = Close File(refnum=w211) -> ()  [unwired: 1 in, 2 out]
                        n143 = Close File(refnum=w212) -> ()  [unwired: 1 in, 2 out]
                      }
                    }
                    n144 = Open/Create/Replace File(file path (use dialog)=w168, operation (0:open)=T11."open or create") -> (refnum out=w154:refnum<file>)  [unwired: 4 in, 2 out]
                    n145 = Open/Create/Replace File(file path (use dialog)=w167, operation (0:open)=T11."open or create") -> (refnum out=w155:refnum<file>)  [unwired: 4 in, 2 out]
                    n146 = Open/Create/Replace File(file path (use dialog)=w166, operation (0:open)=T11."open or create") -> (refnum out=w156:refnum<file>)  [unwired: 4 in, 2 out]
                    n147 = Open/Create/Replace File(file path (use dialog)=w165, operation (0:open)=T11."open or create") -> (refnum out=w157:refnum<file>)  [unwired: 4 in, 2 out]
                    n148 = Get File Size(file=w154) -> (refnum out=→"FF_On_Ref":refnum<file>, size (in bytes)=→"FF_On_Ptr":i64)  [unwired: 1 in, 1 out]
                    n149 = Get File Size(file=w155) -> (refnum out=→"FF_Off_Ref":refnum<file>, size (in bytes)=→"FF_Off_Ptr":i64)  [unwired: 1 in, 1 out]
                    n150 = Get File Size(file=w156) -> (refnum out=→"NF_On_Ref":refnum<file>, size (in bytes)=→"NF_On_Ptr":i64)  [unwired: 1 in, 1 out]
                    n151 = Get File Size(file=w157) -> (refnum out=→"NF_Off_Ref":refnum<file>, size (in bytes)=→"NF_Off_Ptr":i64)  [unwired: 1 in, 1 out]
                  }
                  frame True {
                    # "Don't need to do anything!"
                  }
                }
              }
              frame #1 {
                # "Writing and plotting retrieved\nweather parameters"
                # "Matlab script goes online and retrieves most recent press, temp, and relative humidity data \nfrom the weather station on the roof of Cobleigh"
                # "Importing the current weather conditions from the COE weather station"
                n152 = disable-structure shown="Disabled" {
                  frame Disabled {
                    n153 = script code="%try\n%s=urlread('http://www.coe.montana.edu/ee/weather/mostCurrentCSV.php');\n%amin=textscan(s,'%s %s %s %s %s %s %s %s %s %s %s %s %s');\n%data=amin{1}{2};\n%[test remain]=strtok(data,',');\n%remain=str2num(remain);\n%press=remain(3)./1000;\n%temp=remain(5);\n%RH=remain(7);\n%catch\npress=.850;\ntemp=20;\nRH=40;\n%end"() -> ()  [unwired: 1 in, 4 out]
                  }
                  frame Enabled {
                  }
                }
                n154 = local read "WS_On/Off"() -> (w233:bool)
                n155 = case shown="True" w233 {
                  frame False {
                  }
                  frame True {
                    n156 = local read "WS visa"() -> (w238:refnum<visa-resource-name>)
                    n157 = call "T_RH_P.vi"("VISA in"=w238, "WS_Commands"=enum16{"OpenWS", "ReadTRHP", "CloseWS"}."ReadTRHP") -> ("TRHP"=w234:T13)  [unwired: 11 in, 2 out]
                    n158 = local write "TRHP"(w234) -> ()
                    n159 = Unbundle By Name(w234) -> ("Temp"=→"Temperature (C)":dbl, "RelH"=→"Relative Humdity (%)":dbl, "Press"=→"Pressure (mb)":dbl)
                  }
                }
              }
              frame #2 {
                # "Frame 3: Read, process, and plot online data\nFrame 4:\nFrame 5: Write the data to the folders from Frame 0 of outter sequence"
                # "Frame 0: Read the online wavelength and adjust to locking tolerance if out of range, Switch to offline DBR\nFrame 1: Read the output power from the Newport meter, calculate and plot the output pulse energy\nFrame 2: Wait 'Scalar Wait Time' for buffer to clear other wavelength data"
                # "Online"
                n160 = stacked-sequence {
                  frame #0 {
                    # "Read the online wavelength and continue adjusting the online DBR if outside the wavelength tolerance\nuntil it is within tolerance"
                    n161 = while {
                      i -> [w241]
                      stop <- w240 stop-if-true
                      # "Frame 2: Decrement DBR current if above tolerance\nFrame 3: Increment DBR current if below tolerance"
                      # "Frame 0: Read the current wavelength from the wavemeter\nFrame 1: Calculate the difference between desired and actual wavelength"
                      # "Continue reading and adjusting online DBR current until within locking tolerance"
                      n162 = stacked-sequence {
                        tunnel: w241 -> [w243 _ _ _ _]
                        tunnel: [_ _ w259 _ _] -> w240
                        frame #0 {
                          n163 = Equal To 0?(x=w243) -> (x = 0?=w242:bool)
                          n164 = case shown="True" w242 {
                            frame False {
                            }
                            frame True {
                              # "Set the wavemeter switch to WV Online"
                              n165 = flat-sequence {
                                frame #0 {
                                n166 = Build Array(FALSE ("Boolean")) -> (w246:bool[])
                                n167 = call-poly <vilib>:"DAQmx Write.vi"("task/channels in"=refnum<k21> "BristolWM", "data"=w246) -> ()  [unwired: 11 in, 3 out]
                                }
                                frame #1 {
                                n168 = Build Array(FALSE ("Boolean")) -> (w249:bool[])
                                n169 = call-poly <vilib>:"DAQmx Write.vi"("task/channels in"=refnum<k21> "HSRL_WV_switch", "data"=w249) -> ()  [unwired: 11 in, 3 out]
                                }
                              }
                            }
                          }
                        }
                        frame #1 {
                          # "Reading the wavelength from the wavemeter"
                          n170 = flat-sequence {
                            tunnel: [w252] -> w251
                            tunnel: w251 -> [w255]
                            tunnel: [w254] -> w250
                            tunnel: w250 -> [w258]
                            frame #0 {
                              n171 = local read "Bristol In"() -> (w253:i32)
                              n172 = dll-call lib="C:/Users/H2ODial/Desktop/Shared Telescope WV DIAL Code/bristol/CLDevIface.dll" fn="CLOpenUSBSerialDevice"("commPort"=w253) -> ("return type"=w252:i32)  [unwired: 4 in, 2 out]
                            }
                            frame #1 {
                              n173 = dll-call lib="C:/Users/H2ODial/Desktop/Shared Telescope WV DIAL Code/bristol/CLDevIface.dll" fn="CLGetLambdaReading"("devHandle"=w255) -> ("return type"=→"WV Online Read (nm)":dbl, "devHandle"=w254:i32)  [unwired: 3 in, 2 out]
                            }
                            frame #2 {
                              n174 = dll-call lib="C:/Users/H2ODial/Desktop/Shared Telescope WV DIAL Code/bristol/CLDevIface.dll" fn="CLCloseDevice"("commPort"=w258) -> ("return type"=w257:i32)  [unwired: 4 in, 2 out]
                              n175 = local write "Bristol Out"(w257) -> ()
                            }
                          }
                        }
                        frame #2 {
                          # "If WL difference is within tolerance, stop looping, and illuminate 'Wavelength Lock Online' indicator"
                          # "Calculating the difference between the actual and desired online wavelength"
                          n176 = local read "WV Online Read (nm)"() -> (w262:dbl)
                          n177 = local read "Online_Tol"() -> (w267:dbl)
                          n178 = Multiply(x=-1.0, y=w267) -> (x*y=w268:dbl)
                          n179 = Subtract(x=w262, y="WV Online Set (nm)") -> (x-y=w263:dbl)
                          "Online_Diff" <- w263
                          n180 = Greater?(x=w263, y=w268) -> (0:w264:bool)
                          n181 = Less?(x=w263, y=w267) -> (x < y?=w265:bool)
                          n182 = And(x=w264, y=w265) -> (x .and. y?=w261:bool)
                          "WV Online Locked" <- w261
                          n183 = Or(x=w261, y="Cancel online") -> (x .or. y?=w259:bool)
                        }
                        frame #3 {
                          # "If the wavelength difference is greater that 0.0002 nm, decrement the \nDBR current by 0.01 mA"
                          n184 = local read "Online_Diff"() -> (w272:dbl)
                          n185 = Greater Or Equal?(x=w272, y="Online_Tol") -> (x >= y?=w271:bool)
                          n186 = case shown="True" w271 {
                            frame False {
                              # "Wavelength difference is not greater than 0.0002 nm, do nothing"
                            }
                            frame True {
                              # "Generating a command string\nto decrement the current"
                              # "WL difference is greater than 0.0002 nm,\ndecrement the DBR current by 0.01 mA"
                              n187 = local read "Settings"() -> (w279:T6)
                              n188 = local read "temp step size"() -> (w274:dbl)
                              n189 = Unbundle By Name(w279) -> ("WV Online TEC"=w278:dbl)
                              n190 = local read "Device In"() -> (w275:refnum<visa-resource-name>)
                              n191 = Subtract(x=w278, y=w274) -> (x-y=w277:dbl)
                              n192 = Bundle By Name(cluster=w279, "WV Online TEC"=w277, "Module"=T12."WV Online TEC") -> (w281:T6)
                              n193 = call "TL_Driver_v2.vi"("Device In"=w275, "Commands"=T9."SET", "Settings"=w281) -> ("Readings"=w280:T7)  [unwired: 9 in, 3 out]
                              n194 = local write "Settings"(w281) -> ()
                              n195 = local write "Readings"(w280) -> ()
                            }
                          }
                        }
                        frame #4 {
                          # "If WL difference is < 0.0002 nm, increment the DBR current"
                          n196 = local read "Online_Tol"() -> (w283:dbl)
                          n197 = local read "Online_Diff"() -> (w286:dbl)
                          n198 = Multiply(x=-1.0, y=w283) -> (x*y=w282:dbl)
                          n199 = Less Or Equal?(x=w286, y=w282) -> (x <= y?=w285:bool)
                          n200 = case shown="True" w285 {
                            frame False {
                              # "WL difference is no <= to -0.0002 nm, do nothing"
                            }
                            frame True {
                              # "WL difference is < -0.0002,\nincrement the DBR current by 0.01 mA"
                              # "Generating a command string\nto decrement the current"
                              n201 = local read "Settings"() -> (w295:T6)
                              n202 = local read "temp step size"() -> (w288:dbl)
                              n203 = Unbundle By Name(w295) -> ("WV Online TEC"=w292:dbl)
                              n204 = local read "Device In"() -> (w289:refnum<visa-resource-name>)
                              n205 = Add(x=w292, y=w288) -> (x+y=w291:dbl)
                              n206 = Bundle By Name(cluster=w295, "WV Online TEC"=w291, "Module"=T12."WV Online TEC") -> (w294:T6)
                              n207 = call "TL_Driver_v2.vi"("Device In"=w289, "Commands"=T9."SET", "Settings"=w294) -> ("Readings"=w293:T7)  [unwired: 9 in, 3 out]
                              n208 = local write "Settings"(w294) -> ()
                              n209 = local write "Readings"(w293) -> ()
                            }
                          }
                        }
                      }
                    }
                  }
                  frame #1 {
                    # "Converting to pulse energy, assumes 5 percent pickoff"
                    # "Reading the Newport Power meter"
                    # "Reading the output power of the laser transmitter from the Newport power meter, once read, convert to corresponding pulse energy and plot"
                    n210 = local read "Newport Device Key"() -> (w300:string)
                    n211 = local read "NewportRef"() -> (w296:refnum<k24>)
                    n212 = disable-structure shown="Enabled" {
                      frame Enabled {
                        # "Plotting the online and offling pulse energies"
                        n213 = local read "Online Pulse Energy"() -> (w311:dbl)
                        n214 = local read "Offline Pulse Energy"() -> (w310:dbl)
                        n215 = Bundle("Online Pulse Energy"=w311, "Offline Pulse Energy"=w310) -> (→"Pulse Energy (Micro Joule)":T15)  [unwired: 1 in]
                      }
                      frame Disabled {
                      }
                    }
                    n216 = Number To Decimal String(number="SampleSize") -> (decimal integer string=w298:string)  [unwired: 1 in]
                    n217 = invoke class="PowerMeterCommands" method="PerformDAQ"(reference=w296, "deviceKey"=w300, "interval"="1", "sampleSize"=w298) -> ("PerformDAQ"=w301:dbl[])  [unwired: 2 in, 5 out]
                    n218 = call-poly <vilib>:"Mean.vi"("X"=w301) -> ("mean"=w299:dbl)  [unwired: 1 out]
                    n219 = Multiply(x=w299, y=1000.0) -> (x*y=w307:dbl)
                    n220 = Divide(x=w307, y=0.05) -> (x/y=w305:dbl)
                    n221 = Divide(x=w305, y=7.0) -> (x/y=→"Online Pulse Energy":dbl)
                  }
                  frame #2 {
                    # "Wait 'Scalar Wait Time' for the next available batch of scalar card data"
                    n222 = local read "AMCS_Profile"() -> (w312:i32)
                    n223 = disable-structure shown="Disabled" {
                      frame Disabled {
                        # "Waiting 'Scalar Wait Time'"
                        n224 = Wait (ms)(milliseconds to wait="Scalar Wait Time") -> ()  [unwired: 1 out]
                      }
                      frame Enabled {
                      }
                    }
                    n225 = while {
                      tunnel: [w319] -> w313
                      tunnel: [w315] -> _
                      tunnel: w312 -> [w315]
                      stop <- w317 stop-if-true
                      n226 = global read "AMCS_Data.vi" "AMCS_Profile"() -> (w319:i32)
                      n227 = Wait (ms)(milliseconds to wait=u32 10) -> ()  [unwired: 1 out]
                      n228 = Equal?(x=w319, y=w315) -> (x = y?=w318:bool)
                      n229 = case shown="False" w318 {
                        tunnel: [TRUE FALSE] -> w317
                        frame False {
                        }
                        frame True {
                        }
                      }
                    }
                    "AMCS_Profile" <- w313
                  }
                  frame #3 {
                    # "convert time per range bin to meters\nand calculate smoothed bins using\nsmoothing range"
                    # "Plotting online cross section and smoothed online data"
                    # "Calculate the bin by bin mean of the data"
                    # "Collect 'Integration Period (Seconds)' number\nof scalar data"
                    # "Reading, processing, and plotting the online data"
                    n230 = local read "Data Reads (number of loops)"() -> (w347:i32)
                    n231 = for {
                      N: w347 -> [_]
                      tunnel: [w368] -> w359 mode=indexing
                      tunnel: [w367] -> w322 mode=indexing
                      # "Scalar Data is retrieved from Global \nVariable that scaler.vi is writing to,"
                      n232 = global read "AMCS_Data.vi" "AMCS_Data"() -> (w371:u16[][])
                      n233 = disable-structure shown="Disabled" {
                        frame Disabled {
                          n234 = global read "Scalar_Data_3.vi" "Scalar Data 3"() -> ()  [unwired: 1 out]
                          n235 = global read "Scalar_Data.vi" "Scalar Data"() -> ()  [unwired: 1 out]
                        }
                        frame Enabled {
                        }
                      }
                      n236 = Index Array(array=w371, index (row) #1=0 ("index (row)"), index (row) #2=2 ("index (row)")) -> (element #1=w368:u16[], element #2=w367:u16[])  [unwired: 2 in]
                    }
                    n237 = Transpose 2D Array(2D array=w359) -> (transposed array=w363:u16[][])
                    n238 = Transpose 2D Array(2D array=w322) -> (transposed array=w345:u16[][])
                    n239 = for {
                      tunnel: w363 -> [w373] mode=indexing
                      tunnel: [w372] -> w364 mode=indexing
                      n240 = call-poly <vilib>:"Mean.vi"("X"=w373) -> ("mean"=w372:dbl)  [unwired: 1 out]
                    }
                    n241 = for {
                      tunnel: w345 -> [w366] mode=indexing
                      tunnel: [w365] -> w346 mode=indexing
                      n242 = call-poly <vilib>:"Mean.vi"("X"=w366) -> ("mean"=w365:dbl)  [unwired: 1 out]
                    }
                    n243 = local read "bins"() -> (w339:u32)
                    n244 = Array Subset(array=w364, index=1 ("dimension size"), length=w339) -> (w351:dbl[])
                    n245 = Array Subset(array=w346, index=1 ("dimension size"), length=w339) -> (w343:dbl[])
                    n246 = local read "background length"() -> (w329:i32)
                    n247 = local read "background start"() -> (w330:u32)
                    n248 = Array Size(array=w351) -> (size(s)=w348:i32)
                    n249 = Array Size(array=w343) -> (size(s)=w340:i32)
                    n250 = Initialize Array(1.0 ("element"), w348) -> (w350:dbl[])
                    n251 = Initialize Array(1.0 ("element"), w340) -> (w342:dbl[])
                    n252 = Multiply(x=w351, y=w350) -> (x*y=w352:dbl[])
                    "CH 0 Bin Readings" <- w352
                    n253 = Multiply(x=w343, y=w342) -> (x*y=w333:dbl[])
                    "CH 2 Bin Readings" <- w333
                    n254 = local read "Total DIAL Integration Time (Minutes)"() -> (w355:i32)
                    n255 = local read "Time Resolution Per Bin(ns)"() -> (w325:u32)
                    n256 = Array Subset(array=w352, index=w330, length=w329) -> (w361:dbl[])
                    n257 = Array Subset(array=w333, index=w330, length=w329) -> (w335:dbl[])
                    n258 = call-poly <vilib>:"Mean.vi"("X"=w361) -> ("mean"=w360:dbl)  [unwired: 1 out]
                    n259 = call-poly <vilib>:"Mean.vi"("X"=w335) -> ("mean"=w336:dbl)  [unwired: 1 out]
                    n260 = Divide(x=w355, y=w347) -> (x/y=w353:dbl)
                    n261 = local read "Index"() -> (w334:i32)
                    n262 = Subtract(x=w352, y=w360) -> (x-y=w357:dbl[])
                    n263 = Subtract(x=w333, y=w336) -> (x-y=w337:dbl[])
                    n264 = To Double Precision Float(number=w325) -> (double precision float=w326:dbl)
                    n265 = Multiply(x=w353, y=60.0) -> (x*y=w331:dbl)
                    n266 = Multiply(x=w326, y=0.15) -> (x*y=w328:dbl)
                    n267 = call "Ring Buffer Online Near.vi"("Index"=w334, "Profiles to Average"=w331, "Input Array"=w337) -> ("AvgArray"=w338:dbl[])  [unwired: 7 in, 1 out]
                    n268 = call "Ring Buffer Online Far.vi"("Index"=w334, "Profiles to Average"=w331, "Input Array"=w357) -> ("AvgArray"=w356:dbl[])  [unwired: 7 in, 1 out]
                    n269 = Divide(x="Smoothing Range", y=w328) -> (x/y=w323:dbl)
                    "Smoothed Bins" <- w323
                    n270 = call "Smooth Arrray.vi"("smooth size"=w323, "Raw Array"=w356) -> ("Smoothed Array"=→"CH0 (WV on) smoothed":dbl[])  [unwired: 9 in]
                    n271 = call "Smooth Arrray.vi"("smooth size"=w323, "Raw Array"=w338) -> ("Smoothed Array"=→"CH2 (molecular) smoothed":dbl[])  [unwired: 9 in]
                    n272 = disable-structure shown="Disabled" {
                      frame Disabled {
                        n273 = script code="format long;\ncounts=sum(Online);\nif counts >=0.5e6\ntime=time;\nelse\ntime=time\nend"() -> ()  [unwired: 3 in, 2 out]
                      }
                      frame Enabled {
                      }
                    }
                  }
                  frame #4 {
                    # "Toggling the Agiltron switch to the offline DBR seed laser"
                    n274 = disable-structure shown="Disabled" {
                      frame Disabled {
                        n275 = flat-sequence {
                          frame #0 {
                            # "Second one"
                            # "Command the switch to switch to position 2\ncorresponding to the offline DBR"
                            # "Hex string command \ncorrespond to offline"
                            n276 = VISA Write(VISA resource name="Switch Comm Port", write buffer="\u0001\u0012\u0000\u0001") -> ()  [unwired: 1 in, 3 out]
                          }
                        }
                      }
                      frame Enabled {
                      }
                    }
                  }
                  frame #5 {
                    # "Save the recently collected online data if 'Save Data?' is true"
                    n277 = case shown="True" "Save Data?" {
                      frame False {
                        # "'Save Data?' is false, do nothing"
                      }
                      frame True {
                        # "'Save Data?' is true, save onfline data to the Data Disk"
                        # "Write only one copy of data at this time"
                        # "Retrieve Julian Date"
                        n278 = local read "Readings"() -> (w379:T7)
                        n279 = local read "Time Resolution Per Bin(ns)"() -> (w387:u32)
                        n280 = Unbundle By Name(w379) -> ("WV OnLine TEC"=w378:dbl)
                        n281 = local read "Number of Accumulates"() -> (w385:u32)
                        n282 = Unbundle By Name(w379) -> ("HSRL TEC"=w377:dbl)
                        n283 = local read "WV Online Read (nm)"() -> (w380:dbl)
                        n284 = local write "DataOpen"(TRUE ("DataOpen")) -> ()
                        n285 = local read "Number of Bins"() -> (w386:u32)
                        n286 = local read "HSRL Read (nm)"() -> (w381:dbl)
                        n287 = local read "Online Pulse Energy"() -> (w408:dbl)
                        n288 = local read "CH 0 Bin Readings"() -> (w410:dbl[])
                        n289 = To Double Precision Float(number=w387) -> (double precision float=w382:dbl)
                        n290 = To Double Precision Float(number=w386) -> (double precision float=w383:dbl)
                        n291 = To Double Precision Float(number=w385) -> (double precision float=w384:dbl)
                        n292 = local read "CH 2 Bin Readings"() -> (w407:dbl[])
                        n293 = call "Julian_Date_2.vi"() -> ("Julian Date"=w409:dbl)  [unwired: 11 in]
                        n294 = Build Array (concatenate)(w409, w380, w378, w408, w382, w383, w384, w410) -> (w402:dbl[])
                        n295 = Build Array (concatenate)(w409, w381, w377, w408, w382, w383, w384, w407) -> (w392:dbl[])
                        n296 = local read "NF_On_Ref"() -> (w390:refnum<file>)
                        n297 = local read "FF_On_Ref"() -> (w406:refnum<file>)
                        n298 = local read "NF_On_Ptr"() -> (w391:i64)
                        n299 = local read "FF_On_Ptr"() -> (w405:i64)
                        n300 = Set File Position(offset (in bytes) (0)=w405, refnum=w406) -> (refnum out=w403:refnum<file>, error out=w400:errorcluster)  [unwired: 2 in]
                        n301 = Set File Position(offset (in bytes) (0)=w391, refnum=w390) -> (refnum out=w396:refnum<file>, error out=w394:errorcluster)  [unwired: 2 in]
                        n302 = Write to Binary File(file (use dialog)=w396, data=w392, error in=w394, 5:FALSE ("prepend array or string size? (T)")) -> (refnum out=w395:refnum<file>, error out=w393:errorcluster)  [unwired: 2 in, 1 out]
                        n303 = Write to Binary File(file (use dialog)=w403, data=w402, error in=w400, 5:FALSE ("prepend array or string size? (T)")) -> (refnum out=w401:refnum<file>, error out=w399:errorcluster)  [unwired: 2 in, 1 out]
                        n304 = Get File Position(4:w393, 7:w395) -> (2:w389:i64)  [unwired: 2 out]
                        n305 = Get File Position(4:w399, 7:w401) -> (2:w398:i64)  [unwired: 2 out]
                        n306 = local write "NF_On_Ptr"(w389) -> ()
                        n307 = local write "FF_On_Ptr"(w398) -> ()
                      }
                    }
                  }
                }
              }
              frame #3 {
                # "Frame 3: Read offline data, calculate aerosol data, and plot offline and normalized relative backscatter\nFrame 4:\nFrame 5: Save the offline data and related information"
                # "Frame 0: Read the offline wavelength and lock if necessary, Switch to online DBR\nFrame 1: Read the output power from the Newport power meter\nFrame 2: Wait 'Scalar Wait Time' for buffers to clear of online contiminated data"
                # "offline"
                n308 = stacked-sequence {
                  frame #0 {
                    # "Following Locking the Offline wavelength, check and lock the HSRL 780 nm wavelength"
                    # "Every 60 data collection cycles, read the offline DBR wavelength, and if outside of wavelength tolerance, adjust DBR current until within tolerance"
                    n309 = local read "L_Count"() -> (w412:i32)
                    n310 = Quotient & Remainder(x=w412, y=60.0) -> (x-y*floor(x/y)=w413:dbl)  [unwired: 1 out]
                    n311 = Equal To 0?(x=w413) -> (x = 0?=w411:bool)
                    n312 = case shown="True" w411 {
                      frame False {
                      }
                      frame True {
                        n313 = flat-sequence {
                          frame #0 {
                            n314 = while {
                              i -> [w418]
                              stop <- w416 stop-if-true
                              # "If WL difference is within tolerance, stop looping, and illuminate 'Wavelength Lock Offline' indicator"
                              # "Frame 2: Decrement DBR if above tolerance\nFrame 3: Increment DBR if below tolerance"
                              # "Frame 0: Read the wavelength from the wavemeter\nFrame 1: Calculate the difference between desired and actual wavelength"
                              # "Continue reading and adjusting offline DBR until within locking tolerance"
                              n315 = stacked-sequence {
                                tunnel: w418 -> [w420 _ _ _ _]
                                tunnel: [_ _ w434 _ _] -> w415
                                frame #0 {
                                n316 = Equal To 0?(x=w420) -> (x = 0?=w419:bool)
                                n317 = case shown="True" w419 {
                                frame False {
                                }
                                frame True {
                                # "Set the TSOA switch to\namplify the offline wavelength"
                                n318 = Build Array(TRUE ("Boolean")) -> (w422:bool[])
                                n319 = call-poly <vilib>:"DAQmx Write.vi"("task/channels in"=refnum<k21> "BristolWM", "data"=w422) -> ()  [unwired: 11 in, 3 out]
                                n320 = Wait (ms)(milliseconds to wait=u32 3200) -> ()  [unwired: 1 out]
                                }
                                }
                                }
                                frame #1 {
                                # "Reading the wavelength from the wavemeter"
                                n321 = flat-sequence {
                                tunnel: [w427] -> w426
                                tunnel: w426 -> [w430]
                                tunnel: [w429] -> w425
                                tunnel: w425 -> [w433]
                                frame #0 {
                                n322 = local read "Bristol In"() -> (w428:i32)
                                n323 = dll-call lib="C:/Users/H2ODial/Desktop/Shared Telescope WV DIAL Code/bristol/CLDevIface.dll" fn="CLOpenUSBSerialDevice"("commPort"=w428) -> ("return type"=w427:i32)  [unwired: 4 in, 2 out]
                                }
                                frame #1 {
                                n324 = dll-call lib="C:/Users/H2ODial/Desktop/Shared Telescope WV DIAL Code/bristol/CLDevIface.dll" fn="CLGetLambdaReading"("devHandle"=w430) -> ("return type"=→"WV Offline Read (nm)":dbl, "devHandle"=w429:i32)  [unwired: 3 in, 2 out]
                                }
                                frame #2 {
                                n325 = dll-call lib="C:/Users/H2ODial/Desktop/Shared Telescope WV DIAL Code/bristol/CLDevIface.dll" fn="CLCloseDevice"("commPort"=w433) -> ("return type"=w432:i32)  [unwired: 4 in, 2 out]
                                n326 = local write "Bristol Out"(w432) -> ()
                                }
                                }
                                }
                                frame #2 {
                                # "Calculating the difference between the actual and desired online wavelength"
                                n327 = local read "Offline_Tol"() -> (w436:dbl)
                                n328 = local read "WV Offline Read (nm)"() -> (w442:dbl)
                                n329 = Multiply(x=-1.0, y=w436) -> (x*y=w435:dbl)
                                n330 = Subtract(x=w442, y="WV Offline Set (nm)") -> (x-y=w438:dbl)
                                "Oflline_Diff" <- w438
                                n331 = Greater?(x=w438, y=w435) -> (0:w439:bool)
                                n332 = Less?(x=w438, y=w436) -> (x < y?=w440:bool)
                                n333 = And(x=w439, y=w440) -> (x .and. y?=w434:bool)
                                "WV Oflline Locked" <- w434
                                n334 = case shown="True" w434 {
                                frame False {
                                }
                                frame True {
                                # "Set the Wavemeter switch to\nthe HSRL wavelength"
                                n335 = Build Array(TRUE ("Boolean")) -> (w444:bool[])
                                n336 = call-poly <vilib>:"DAQmx Write.vi"("task/channels in"=refnum<k21> "HSRL_WV_switch", "data"=w444) -> ()  [unwired: 11 in, 3 out]
                                n337 = Wait (ms)(milliseconds to wait=u32 3200) -> ()  [unwired: 1 out]
                                }
                                }
                                }
                                frame #3 {
                                # "If the wavelength difference is greater that 0.0002 nm, decrement the \nDBR current by 0.01 mA"
                                n338 = local read "Oflline_Diff"() -> (w449:dbl)
                                n339 = Greater Or Equal?(x=w449, y="Offline_Tol") -> (x >= y?=w448:bool)
                                n340 = case shown="True" w448 {
                                frame False {
                                # "Wavelength difference is not greater than 0.0002 nm, do nothing"
                                }
                                frame True {
                                # "Generating a command string\nto decrement the current"
                                n341 = local read "Settings"() -> (w456:T6)
                                n342 = Unbundle By Name(w456) -> ("WV Offline TEC"=w454:dbl)
                                n343 = Subtract(x=w454, y="temp step size") -> (x-y=w453:dbl)
                                n344 = local read "Device In"() -> (w451:refnum<visa-resource-name>)
                                n345 = Bundle By Name(cluster=w456, "WV Offline TEC"=w453, "Module"=T12."WV Offline TEC") -> (w457:T6)
                                n346 = call "TL_Driver_v2.vi"("Device In"=w451, "Commands"=T9."SET", "Settings"=w457) -> ("Readings"=w458:T7)  [unwired: 9 in, 3 out]
                                n347 = local write "Settings"(w457) -> ()
                                n348 = local write "Readings"(w458) -> ()
                                }
                                }
                                }
                                frame #4 {
                                # "If WL difference is < 0.0002 nm, increment the DBR temperature"
                                n349 = local read "Oflline_Diff"() -> (w461:dbl)
                                n350 = Less Or Equal?(x=w461, y=-0.0001) -> (x <= y?=w459:bool)
                                n351 = case shown="True" w459 {
                                frame False {
                                # "WL difference is no <= to -0.0002 nm, do nothing"
                                }
                                frame True {
                                # "Generating a command string\nto decrement the current"
                                # "WL difference is less than 0.0002 nm,\nincrement the DBR current by 0.01 mA"
                                n352 = local read "Settings"() -> (w469:T6)
                                n353 = Unbundle By Name(w469) -> ("WV Offline TEC"=w467:dbl)
                                n354 = local read "temp step size"() -> (w463:dbl)
                                n355 = Add(x=w467, y=w463) -> (x+y=w466:dbl)
                                n356 = local read "Device In"() -> (w464:refnum<visa-resource-name>)
                                n357 = Bundle By Name(cluster=w469, "WV Offline TEC"=w466, "Module"=T12."WV Offline TEC") -> (w470:T6)
                                n358 = call "TL_Driver_v2.vi"("Device In"=w464, "Commands"=T9."SET", "Settings"=w470) -> ("Readings"=w468:T7)  [unwired: 9 in, 3 out]
                                n359 = local write "Settings"(w470) -> ()
                                n360 = local write "Readings"(w468) -> ()
                                }
                                }
                                }
                              }
                              n361 = Or(x=w415, y="Cancel Offline") -> (x .or. y?=w416:bool)
                            }
                          }
                          frame #1 {
                            n362 = while {
                              i -> [w474]
                              stop <- w472 stop-if-true
                              # "If WL difference is within tolerance, stop looping, and illuminate 'Wavelength Lock Offline' indicator"
                              # "Frame 2: Decrement DBR if above tolerance\nFrame 3: Increment DBR if below tolerance"
                              # "Frame 0: Read the wavelength from the wavemeter\nFrame 1: Calculate the difference between desired and actual wavelength"
                              # "Continue reading and adjusting offline DBR until within locking tolerance"
                              n363 = stacked-sequence {
                                tunnel: w474 -> [w476 _ _ _ _]
                                tunnel: [_ _ w489 _ _] -> w471
                                frame #0 {
                                n364 = Equal To 0?(x=w476) -> (x = 0?=w475:bool)
                                n365 = case shown="True" w475 {
                                frame False {
                                }
                                frame True {
                                # "Set the Wavemeter to\nthe non HSRL wavelength"
                                n366 = Build Array(TRUE ("Boolean")) -> (w477:bool[])
                                n367 = call-poly <vilib>:"DAQmx Write.vi"("task/channels in"=refnum<k21> "HSRL_WV_switch", "data"=w477) -> ()  [unwired: 11 in, 3 out]
                                }
                                }
                                }
                                frame #1 {
                                # "Reading the wavelength from the wavemeter"
                                n368 = flat-sequence {
                                tunnel: [w482] -> w481
                                tunnel: w481 -> [w485]
                                tunnel: [w484] -> w480
                                tunnel: w480 -> [w488]
                                frame #0 {
                                n369 = local read "Bristol In"() -> (w483:i32)
                                n370 = dll-call lib="C:/Users/H2ODial/Desktop/Shared Telescope WV DIAL Code/bristol/CLDevIface.dll" fn="CLOpenUSBSerialDevice"("commPort"=w483) -> ("return type"=w482:i32)  [unwired: 4 in, 2 out]
                                }
                                frame #1 {
                                n371 = dll-call lib="C:/Users/H2ODial/Desktop/Shared Telescope WV DIAL Code/bristol/CLDevIface.dll" fn="CLGetLambdaReading"("devHandle"=w485) -> ("return type"=→"HSRL Read (nm)":dbl, "devHandle"=w484:i32)  [unwired: 3 in, 2 out]
                                }
                                frame #2 {
                                n372 = dll-call lib="C:/Users/H2ODial/Desktop/Shared Telescope WV DIAL Code/bristol/CLDevIface.dll" fn="CLCloseDevice"("commPort"=w488) -> ("return type"=w487:i32)  [unwired: 4 in, 2 out]
                                n373 = local write "Bristol Out"(w487) -> ()
                                }
                                }
                                }
                                frame #2 {
                                # "Calculating the difference between the actual and desired online wavelength"
                                n374 = local read "HSRL_Tol"() -> (w491:dbl)
                                n375 = local read "HSRL Read (nm)"() -> (w497:dbl)
                                n376 = Multiply(x=-1.0, y=w491) -> (x*y=w490:dbl)
                                n377 = Subtract(x=w497, y="HSRL Set (nm)") -> (x-y=w493:dbl)
                                "HSRL_Diff" <- w493
                                n378 = Greater?(x=w493, y=w490) -> (0:w494:bool)
                                n379 = Less?(x=w493, y=w491) -> (x < y?=w495:bool)
                                n380 = And(x=w494, y=w495) -> (x .and. y?=w489:bool)
                                "HSRL Locked" <- w489
                                n381 = case shown="True" w489 {
                                frame False {
                                }
                                frame True {
                                # "Set the Wavementer switch to WV Online"
                                n382 = Build Array(FALSE ("Boolean")) -> (w499:bool[])
                                n383 = Build Array(FALSE ("Boolean")) -> (w503:bool[])
                                n384 = call-poly <vilib>:"DAQmx Write.vi"("task/channels in"=refnum<k21> "BristolWM", "data"=w503) -> ("error out"=w498:errorcluster)  [unwired: 11 in, 2 out]
                                n385 = call-poly <vilib>:"DAQmx Write.vi"("task/channels in"=refnum<k21> "HSRL_WV_switch", "data"=w499, "error in"=w498) -> ()  [unwired: 10 in, 3 out]
                                n386 = Wait (ms)(milliseconds to wait=u32 3200) -> ()  [unwired: 1 out]
                                }
                                }
                                }
                                frame #3 {
                                # "If the wavelength difference is greater that 0.0002 nm, decrement the \nDBR current by 0.01 mA"
                                n387 = local read "HSRL_Diff"() -> (w508:dbl)
                                n388 = Greater Or Equal?(x=w508, y="HSRL_Tol") -> (x >= y?=w507:bool)
                                n389 = case shown="True" w507 {
                                frame False {
                                # "Wavelength difference is not greater than 0.0002 nm, do nothing"
                                }
                                frame True {
                                # "Generating a command string\nto decrement the current"
                                n390 = local read "Settings"() -> (w515:T6)
                                n391 = local read "temp step size"() -> (w509:dbl)
                                n392 = Unbundle By Name(w515) -> ("HSRL TEC"=w514:dbl)
                                n393 = Subtract(x=w514, y=w509) -> (x-y=w513:dbl)
                                n394 = local read "Device In"() -> (w511:refnum<visa-resource-name>)
                                n395 = Bundle By Name(cluster=w515, "HSRL TEC"=w513, "Module"=T12."HSRL TEC") -> (w516:T6)
                                n396 = call "TL_Driver_v2.vi"("Device In"=w511, "Commands"=T9."SET", "Settings"=w516) -> ("Readings"=w517:T7)  [unwired: 9 in, 3 out]
                                n397 = local write "Settings"(w516) -> ()
                                n398 = local write "Readings"(w517) -> ()
                                }
                                }
                                }
                                frame #4 {
                                # "If WL difference is < 0.0002 nm, increment the DBR temperature"
                                n399 = local read "HSRL_Diff"() -> (w520:dbl)
                                n400 = Less Or Equal?(x=w520, y=-0.0001) -> (x <= y?=w518:bool)
                                n401 = case shown="True" w518 {
                                frame False {
                                # "WL difference is no <= to -0.0002 nm, do nothing"
                                }
                                frame True {
                                # "Generating a command string\nto decrement the current"
                                # "WL difference is less than 0.0002 nm,\nincrement the DBR current by 0.01 mA"
                                n402 = local read "Settings"() -> (w528:T6)
                                n403 = local read "temp step size"() -> (w521:dbl)
                                n404 = Unbundle By Name(w528) -> ("HSRL TEC"=w526:dbl)
                                n405 = Add(x=w526, y=w521) -> (x+y=w525:dbl)
                                n406 = local read "Device In"() -> (w523:refnum<visa-resource-name>)
                                n407 = Bundle By Name(cluster=w528, "HSRL TEC"=w525, "Module"=T12."HSRL TEC") -> (w529:T6)
                                n408 = call "TL_Driver_v2.vi"("Device In"=w523, "Commands"=T9."SET", "Settings"=w529) -> ("Readings"=w527:T7)  [unwired: 9 in, 3 out]
                                n409 = local write "Settings"(w529) -> ()
                                n410 = local write "Readings"(w527) -> ()
                                }
                                }
                                }
                              }
                              n411 = Or(x=w471, y="Cancel HSRL") -> (x .or. y?=w472:bool)
                            }
                          }
                        }
                      }
                    }
                  }
                  frame #1 {
                    # "Reading the power meter"
                    # "Updating the pulse energy plot"
                    # "Converting to pulse energy"
                    # "Reading the offline output power, converting to pulse energy,  and updating the Pulse energy plot"
                    n412 = local read "SampleSize"() -> (w532:i32)
                    n413 = local read "Newport Device Key"() -> (w533:string)
                    n414 = local read "Online Pulse Energy"() -> (w539:dbl)
                    n415 = local read "Offline Pulse Energy"() -> (w538:dbl)
                    n416 = local read "NewportRef"() -> (w530:refnum<k24>)
                    n417 = Number To Decimal String(number=w532) -> (decimal integer string=w534:string)  [unwired: 1 in]
                    n418 = invoke class="PowerMeterCommands" method="PerformDAQ"(reference=w530, "deviceKey"=w533, "interval"="1", "sampleSize"=w534) -> ("PerformDAQ"=w535:dbl[])  [unwired: 2 in, 5 out]
                    n419 = Bundle("Online Pulse Energy"=w539, "Offline Pulse Energy"=w538) -> (w537:T15)  [unwired: 1 in]
                    n420 = local write "Pulse Energy (Micro Joule)"(w537) -> ()
                    n421 = call-poly <vilib>:"Mean.vi"("X"=w535) -> ("mean"=w531:dbl)  [unwired: 1 out]
                    n422 = Multiply(x=w531, y=1000.0) -> (x*y=w544:dbl)
                    n423 = Divide(x=w544, y=0.05) -> (x/y=w542:dbl)
                    n424 = Divide(x=w542, y=7.0) -> (x/y=→"Offline Pulse Energy":dbl)
                  }
                  frame #2 {
                    # "Added in the ability to interactively control the ThorLab  setting (just etalon temp for now)"
                    # "Wait 'Scalar Wait Time' for buffers to clear of online contiminated offline data"
                    n425 = disable-structure shown="Disabled" {
                      frame Disabled {
                        # "Wait 'Scalar Wait Time'"
                        n426 = local read "Scalar Wait Time"() -> (w561:u32)
                        n427 = Wait (ms)(milliseconds to wait=w561) -> ()  [unwired: 1 out]
                      }
                      frame Enabled {
                      }
                    }
                    n428 = event shown="[2] \"Settings.HSRL Etalon TEC\": Value Change" {
                      selector: _ -> [_ _ _]
                      dyn-events: _ -> [_ _ _]
                      timeout: 1 -> [_ _ _]
                      event Timeout {
                        n429 = event-data() -> ()  [unwired: 1 in, 2 out]
                      }
                      event "Settings.WV Etalon TEC": Value Change {
                        # "Generating a command string\nto update the etalon"
                        n430 = event-data() -> ()  [unwired: 1 in, 5 out]
                        n431 = local read "Settings"() -> (w551:T6)
                        n432 = Unbundle By Name(w551) -> ("WV Etalon TEC"=w553:dbl)
                        n433 = local read "Device In"() -> (w547:refnum<visa-resource-name>)
                        n434 = Bundle By Name(cluster=w551, "WV Etalon TEC"=w553, "Module"=T12."WV Etalon TEC") -> (w549:T6)
                        n435 = call "TL_Driver_v2.vi"("Device In"=w547, "Commands"=T9."SET", "Settings"=w549) -> ("Readings"=w550:T7)  [unwired: 9 in, 3 out]
                        n436 = local write "Readings"(w550) -> ()
                        n437 = local write "Settings"(w549) -> ()
                      }
                      event "Settings.HSRL Etalon TEC": Value Change {
                        # "Generating a command string\nto update the etalon"
                        n438 = event-data() -> ()  [unwired: 1 in, 5 out]
                        n439 = local read "Settings"() -> (w558:T6)
                        n440 = Unbundle By Name(w558) -> ("HSRL Etalon TEC"=w560:dbl)
                        n441 = local read "Device In"() -> (w554:refnum<visa-resource-name>)
                        n442 = Bundle By Name(cluster=w558, "HSRL Etalon TEC"=w560, "Module"=T12."HSRL Etalon TEC") -> (w556:T6)
                        n443 = call "TL_Driver_v2.vi"("Device In"=w554, "Commands"=T9."SET", "Settings"=w556) -> ("Readings"=w557:T7)  [unwired: 9 in, 3 out]
                        n444 = local write "Readings"(w557) -> ()
                        n445 = local write "Settings"(w556) -> ()
                      }
                    }
                  }
                  frame #3 {
                    w588 = 1 ("dimension size")
                    # "Read in latest scalar card data from \n'Scalar Data' global variable that \nscaler.vi is writing to, then wait 1 sec\nfor next batch of data"
                    # "Calculating/Plotting smoothed data,\ncross sections etc."
                    # "Pick off data with\nout header"
                    # "Calculate mean bin by bin mean"
                    # "Reading in 'Integration Period (Seconds)' of data"
                    # "Read the offline data from the scalar card, perform smoothing, calculate normalized relative backscatter, and plot"
                    # "Collects Data From Card,\nSends It To The Chart,\nAnd Saves A Copy As A\nFile If Option Selected On\nFront Panel"
                    n446 = for {
                      N: "Data Reads (number of loops)" -> [_]
                      tunnel: [w646] -> w577 mode=indexing
                      tunnel: [w645] -> w576 mode=indexing
                      n447 = global read "AMCS_Data.vi" "AMCS_Data"() -> (w647:u16[][])
                      n448 = disable-structure shown="Disabled" {
                        frame Disabled {
                          n449 = global read "Scalar_Data_4.vi" "Scalar Data 4"() -> ()  [unwired: 1 out]
                          n450 = global read "Scalar_Data_2.vi" "Scalar Data 2"() -> ()  [unwired: 1 out]
                        }
                        frame Enabled {
                        }
                      }
                      n451 = Index Array(array=w647, index (row) #1=1 ("index (row)"), index (row) #2=3 ("index (row)")) -> (element #1=w646:u16[], element #2=w645:u16[])  [unwired: 2 in]
                    }
                    n452 = local read "Total DIAL Integration Time (Minutes)"() -> (w608:i32)
                    n453 = Divide(x=w608, y="Data Reads (number of loops)") -> (x/y=w606:dbl)
                    n454 = local read "Total Aerosol Integration Time (Minutes)"() -> (w610:dbl)
                    n455 = Multiply(x=w606, y=60.0) -> (x*y=w594:dbl)
                    n456 = local read "background length"() -> (w581:i32)
                    n457 = local read "background start"() -> (w582:u32)
                    n458 = Transpose 2D Array(2D array=w577) -> (transposed array=w616:u16[][])
                    n459 = Transpose 2D Array(2D array=w576) -> (transposed array=w600:u16[][])
                    n460 = Divide(x=w610, y="Data Reads (number of loops)") -> (x/y=w611:dbl)
                    n461 = for {
                      tunnel: w616 -> [w653] mode=indexing
                      tunnel: [w652] -> w617 mode=indexing
                      tunnel: w600 -> [w651] mode=indexing
                      tunnel: [w650] -> _ mode=indexing
                      tunnel: [w650] -> w597 mode=indexing
                      n462 = call-poly <vilib>:"Mean.vi"("X"=w653) -> ("mean"=w652:dbl)  [unwired: 1 out]
                      n463 = call-poly <vilib>:"Mean.vi"("X"=w651) -> ("mean"=w650:dbl)  [unwired: 1 out]
                    }
                    n464 = local read "bins"() -> (w589:u32)
                    n465 = Multiply(x=w611, y=60.0) -> (x*y=w573:dbl)
                    n466 = Array Subset(array=w597, index=w588, length=w589) -> (w598:dbl[])
                    "CH3 Bin Readings" <- w598
                    n467 = Array Subset(array=w617, index=w588, length=w589) -> (w596:dbl[])
                    "CH1  Bin Readings" <- w596
                    n468 = Array Subset(array=w598, index=w582, length=w581) -> (w599:dbl[])
                    n469 = Array Subset(array=w596, index=w582, length=w581) -> (w615:dbl[])
                    n470 = local read "Smoothed Bins"() -> (w578:dbl)
                    n471 = call-poly <vilib>:"Mean.vi"("X"=w599) -> ("mean"=w563:dbl)  [unwired: 1 out]
                    n472 = call-poly <vilib>:"Mean.vi"("X"=w615) -> ("mean"=w566:dbl)  [unwired: 1 out]
                    n473 = local read "Index"() -> (w574:i32)
                    n474 = Subtract(x=w598, y=w563) -> (x-y=w575:dbl[])
                    n475 = Subtract(x=w596, y=w566) -> (x-y=w592:dbl[])
                    n476 = call "Ring Buffer Offline Far.vi"("Index"=w574, "Profiles to Average"=w594, "Input Array"=w592) -> ("AvgArray"=w613:dbl[], "RingBufferOut"=→"CH1 RingBuffer long":dbl[][])  [unwired: 7 in]
                    n477 = call "Ring Buffer Aerosol Far.vi"("Index"=w574, "Profiles to Average"=w573, "Input Array"=w592) -> ("AvgArray"=w609:dbl[], "RingBufferOut"=→"CH1 RingBuffer short":dbl[][])  [unwired: 7 in]
                    n478 = call "Ring Buffer Offline Near.vi"("Index"=w574, "Profiles to Average"=w594, "Input Array"=w575) -> ("AvgArray"=w595:dbl[], "RingBufferOut"=→"CH3 RingBuffer long":dbl[][])  [unwired: 7 in]
                    n479 = call "Ring Buffer Aerosol Near.vi"("Index"=w574, "Profiles to Average"=w573, "Input Array"=w575) -> ("AvgArray"=w585:dbl[], "RingBufferOut"=→"CH3 RingBuffer short":dbl[][])  [unwired: 7 in]
                    n480 = Reshape Array(w592, w588, w589) -> (→"CH 1 (WV off) counts display":dbl[][])
                    n481 = Reshape Array(w575, w588, w589) -> (→"CH 3 (HSRL comb) counts display":dbl[][])
                    n482 = call "Smooth Arrray.vi"("smooth size"=w578, "Raw Array"=w613) -> ("Smoothed Array"=→"CH1 (WV off) smooth S":dbl[])  [unwired: 9 in]
                    n483 = call "Smooth Arrray.vi"("smooth size"=w578, "Raw Array"=w609) -> ("Smoothed Array"=w587:dbl[])  [unwired: 9 in]
                    "CH1 (WV off) smooth L" <- w587
                    n484 = call "Smooth Arrray.vi"("smooth size"=w578, "Raw Array"=w595) -> ("Smoothed Array"=→"CH3 (HSRL combined) smooth L":dbl[])  [unwired: 9 in]
                    n485 = call "Smooth Arrray.vi"("smooth size"=w578, "Raw Array"=w585) -> ("Smoothed Array"=w580:dbl[])  [unwired: 9 in]
                    "CH3 (HSRL combined) smooth S" <- w580
                    n486 = local read "Time Resolution Per Bin(ns)"() -> (w571:u32)
                    n487 = local read "Number of Accumulates"() -> (w569:u32)
                    n488 = local read "Temperature (C)"() -> (w605:dbl)
                    n489 = local read "Pressure (mb)"() -> (w604:dbl)
                    n490 = Reciprocal(x=w571) -> (1/x=w570:dbl)
                    n491 = disable-structure shown="Disabled" {
                      disable-tunnel: w605 -> [w644 _]
                      disable-tunnel: w604 -> [w643 _]
                      disable-tunnel: w587 -> [w637 _]
                      disable-tunnel: w566 -> [w624 _]
                      disable-tunnel: w563 -> [w623 _]
                      disable-tunnel: w569 -> [w622 _]
                      disable-tunnel: "dead time" -> [w621 _]
                      disable-tunnel: w580 -> [w620 _]
                      disable-tunnel: 6.0 ("Real") -> [w619 _]
                      disable-tunnel: w571 -> [w618 _]
                      frame Disabled {
                        w640 = 1
                        # "Plotting the normalized relative \nbackscatter"
                        # "Calculating the normalized relative backscatter"
                        # "File path in MATLAB script is of old dial is:\nF:\\Micropulse DIAL\\Micropulse DIAL Matlab\\\nFinal Overlap Function.mat')];"
                        n492 = script code="%accum_num=10000;     % scaler card setting number of accumulations\nt_bin = t_bin/1e9                 % scaler card setting time per bin\n%t_d = 37.3e-9;                % APD dead time from spec sheet\n\n% conversion from accumulated counts to count rate  (c/s)\nc_convert = 1./t_bin./accum_num;\nCR_far = p_raw_far.*c_convert;\nCR_near = p_raw_near.*c_convert;\nCR_total_far = (p_raw_far+b_far).*c_convert;\nCR_total_near = (p_raw_near+b_near).*c_convert;\nb_CR_far =b_far.*c_convert;\nb_CR_near =b_near.*c_convert;\n \n% create a range array\nsize_p =  size(p_raw_far,2);\ngate = t_bin*3e8/2;\nr = (gate:gate:size_p*gate)./1e3; \n   \n%APD correction factor\n D_far = 1./(1-(t_d*CR_total_far));\n D_near = 1./(1-(t_d*CR_total_near));\n\n %Calculating normalize relative backscatter profile\n nrb_far = CR_far.*D_far.*r.^2.*1e-6;\n nrb_near = CR_near.*D_near.*r.^2.*1e-6;"("E"=w619, "temp"=w644, "press"=w643, "p_raw_far"=w637, "b_far"=w624, "b_near"=w623, "p_raw_near"=w620, "accum_num"=w622, "t_d"=w621, "t_bin"=w618) -> ("nrb_far"=w632:cdb[], "D_far"=w629:dbl[], "nrb_near"=w631:cdb[], "D_near"=w628:dbl[])  [unwired: 1 in, 1 out]
                        n493 = local read "bins"() -> (w639:u32)
                        n494 = local read "Altitude Array (km)"() -> (w634:dbl[])
                        n495 = Build Array(w632, w631) -> (w636:cdb[][])
                        n496 = Build Array(w629, w628) -> (w627:dbl[][])
                        n497 = Reshape Array(w631, w640, w639) -> (→"NRB 2":cdb[][])
                        n498 = Reshape Array(w632, w640, w639) -> (→"NRB":cdb[][])
                        n499 = Build Array(w634, w634) -> (w633:dbl[][])
                        n500 = call "Convert to Dynamic Data7"("2D Array"=w627) -> ("Dynamic Data Type"=w626:dynamicdata)  [unwired: 3 in]
                        n501 = call "Convert to Dynamic Data3"("2D Array"=w636) -> ("Dynamic Data Type"=w635:dynamicdata)  [unwired: 3 in]
                        n502 = call "Convert to Dynamic Data4"("2D Array"=w633) -> ("Dynamic Data Type"=w630:dynamicdata)  [unwired: 3 in]
                        n503 = call "Build XY Graph2"("Y Input"=w630, "X Input"=w635) -> ("XY Graph"=→"NRB plot":cluster{"Y":dbl[], "Y":dbl[]}[])  [unwired: 3 in, 6 out]
                        n504 = call "Build XY Graph4"("Y Input"=w630, "X Input"=w626) -> ("XY Graph"=→"Correction":cluster{"Y":dbl[], "Y":dbl[]}[])  [unwired: 3 in, 6 out]
                      }
                      frame Enabled {
                      }
                    }
                    n505 = Divide(x=w570, y=w569) -> (x/y=w567:dbl)
                    n506 = Multiply(x=1000000000.0, y=w567) -> (x*y=w564:dbl)
                    n507 = Multiply(x=w564, y=w566) -> (x*y=w565:dbl)
                    n508 = Multiply(x=w564, y=w563) -> (x*y=w562:dbl)
                    n509 = Bundle(w565, w562) -> (→"?":cluster{dbl, dbl})  [unwired: 1 in]
                  }
                  frame #4 {
                    # "REPLACE WITH NEW AGILTRON TASK!"
                    # "Toggle Agiltron switch to online DBR"
                    n510 = disable-structure shown="Disabled" {
                      frame Disabled {
                        # "ABSORBING"
                        n511 = flat-sequence {
                          frame #0 {
                            # "Third one"
                            # "Command the switch to switch to position 1\ncorresponding to the online DBR"
                            # "Hex string command \ncorrespond to online"
                            n512 = local read "Switch Comm Port"() -> (w657:refnum<visa-resource-name>)
                            n513 = VISA Write(VISA resource name=w657, write buffer="\u0001\u0012\u0000\u0002") -> ()  [unwired: 1 in, 3 out]
                          }
                        }
                        n514 = Build Array(FALSE ("Boolean")) -> (w656:bool[])
                        n515 = call-poly <vilib>:"DAQmx Write.vi"("task/channels in"=refnum<k21> "AgiltronSwitch", "data"=w656) -> ()  [unwired: 11 in, 3 out]
                      }
                      frame Enabled {
                      }
                    }
                  }
                  frame #5 {
                    # "If 'Save Data?' is true, save all relavant offline info"
                    n516 = local read "Save Data?"() -> (w659:bool)
                    n517 = case shown="True" w659 {
                      frame False {
                        # "'Save Data?' is false, do nothing"
                      }
                      frame True {
                        # "Write only one data file at this time"
                        # "Retrive Julian Date"
                        # "'Save Data?' is true, save offline data to the Data Disk"
                        n518 = local read "Readings"() -> (w660:T7)
                        n519 = Unbundle By Name(w660) -> ("WV Offline TEC"=w661:dbl)
                        n520 = Unbundle By Name(w660) -> ("HSRL TEC"=w662:dbl)
                        n521 = local read "HSRL Read (nm)"() -> (w663:dbl)
                        n522 = local read "WV Offline Read (nm)"() -> (w684:dbl)
                        n523 = local read "Relative Humdity (%)"() -> (w688:dbl)
                        n524 = local read "CH3 Bin Readings"() -> (w682:dbl[])
                        n525 = local read "CH1  Bin Readings"() -> (w689:dbl[])
                        n526 = local read "Offline Pulse Energy"() -> (w685:dbl)
                        n527 = local read "Temperature (C)"() -> (w686:dbl)
                        n528 = local read "Pressure (mb)"() -> (w687:dbl)
                        n529 = call "Julian_Date_2.vi"() -> ("Julian Date"=w683:dbl)  [unwired: 11 in]
                        n530 = Build Array (concatenate)(w683, w684, w661, w685, w686, w687, w688, w689) -> (w668:dbl[])
                        n531 = Build Array (concatenate)(w683, w663, w662, w685, w686, w687, w688, w682) -> (w665:dbl[])
                        n532 = local read "FF_Off_Ref"() -> (w670:refnum<file>)
                        n533 = local read "NF_Off_Ref"() -> (w667:refnum<file>)
                        n534 = local read "FF_Off_Ptr"() -> (w669:i64)
                        n535 = local read "NF_Off_Ptr"() -> (w666:i64)
                        n536 = Set File Position(offset (in bytes) (0)=w669, refnum=w670) -> (refnum out=w681:refnum<file>, error out=w679:errorcluster)  [unwired: 2 in]
                        n537 = Set File Position(offset (in bytes) (0)=w666, refnum=w667) -> (refnum out=w677:refnum<file>, error out=w675:errorcluster)  [unwired: 2 in]
                        n538 = Write to Binary File(file (use dialog)=w681, data=w668, error in=w679, 5:FALSE ("prepend array or string size? (T)")) -> (refnum out=w680:refnum<file>, error out=w678:errorcluster)  [unwired: 2 in, 1 out]
                        n539 = Write to Binary File(file (use dialog)=w677, data=w665, error in=w675, 5:FALSE ("prepend array or string size? (T)")) -> (refnum out=w676:refnum<file>, error out=w674:errorcluster)  [unwired: 2 in, 1 out]
                        n540 = Get File Position(4:w678, 7:w680) -> (2:w671:i64)  [unwired: 2 out]
                        n541 = Get File Position(4:w674, 7:w676) -> (2:w664:i64)  [unwired: 2 out]
                        n542 = local write "FF_Off_Ptr"(w671) -> ()
                        n543 = local write "NF_Off_Ptr"(w664) -> ()
                      }
                    }
                  }
                }
              }
              frame #4 {
                n544 = First Call?() -> (First Call?: T/F=w692:bool)
                n545 = Or(x="calculate absorption cross sections", y=w692) -> (x .or. y?=w690:bool)
                n546 = case shown="True" w690 {
                  frame False {
                  }
                  frame True {
                    # "calculate absorption cross sections from HITRAN data base"
                  }
                }
              }
              frame #5 {
                # "Data Processing Far Channel"
                # "Calculating the range resolved water vapor number density and plotting"
              }
            }
          }
        }
        "L_Count" <- w129
      }
    }
  }
  n547 = case shown="True" w3 {
    frame False {
    }
    frame True {
      # "close data files"
      n548 = local read "NF_Off_Ref"() -> (w694:refnum<file>)
      n549 = local read "NF_On_Ref"() -> (w695:refnum<file>)
      n550 = local read "FF_Off_Ref"() -> (w696:refnum<file>)
      n551 = local read "FF_On_Ref"() -> (w697:refnum<file>)
      n552 = local read "WS_On/Off"() -> (w693:bool)
      n553 = case shown="True" w693 {
        frame False {
        }
        frame True {
          n554 = local read "WS visa"() -> (w698:refnum<visa-resource-name>)
          n555 = call "T_RH_P.vi"("VISA in"=w698, "WS_Commands"=enum16{"OpenWS", "ReadTRHP", "CloseWS"}."CloseWS") -> ()  [unwired: 11 in, 3 out]
        }
      }
      n556 = Close File(refnum=w697) -> ()  [unwired: 1 in, 2 out]
      n557 = Close File(refnum=w696) -> ()  [unwired: 1 in, 2 out]
      n558 = Close File(refnum=w695) -> ()  [unwired: 1 in, 2 out]
      n559 = Close File(refnum=w694) -> ()  [unwired: 1 in, 2 out]
    }
  }
  "FileHour" <- -1 ("FileHour")
  "DataOpen" <- FALSE
